vi "Advanced Auto Code.vi"   [LabVIEW 2017]
uses:
  <vilib>/Rock Robotics/WPI/ThirdParty/Phoenix-LabVIEW/Motor Controller/Controls/CTRE_Phoenix_MotorControl_RemoteSourceType.ctl
  <vilib>/Rock Robotics/WPI/ThirdParty/Phoenix-LabVIEW/Motor Controller/Controls/CTRE_Phoenix_MotorControl_ControlMode.ctl
  <vilib>/Rock Robotics/WPI/Utilities/WPI_GetSetVariantRefNum.vi
  <vilib>/Rock Robotics/Network Tables/NT Read String.vi
  Robot Global Data.vi
  <vilib>/Rock Robotics/WPI/RobotDrive/WPI_RobotDriveArcadeDrive_Standard(NoSaturation).vi
  <vilib>/addons/control/pid/pid.llb/PID (DBL).vi
  <vilib>/Rock Robotics/WPI/ThirdParty/Phoenix-LabVIEW/Motor Controller/Get/CTRE_Phoenix_MotorController_GetPulseWidthAll.vi
  <vilib>/addons/control/pid/NI_PID_pid.lvlib
types:
  T1 = cluster{"proportional gain (Kc)":dbl, "integral time (Ti, min)":dbl, "derivative time (Td, min)":dbl}
  T2 = enum16{"DemandType_Neutral", "DemandType_AuxPID", "DemandType_ArbitraryFeedForward"}
  T3 = typedef "CTRE_Phoenix_MotorControl_RemoteSourceType.ctl" = enum16{"Off", "Talon SRX Selected Sensor", "Pigeon IMU Yaw", "Pigeon IMU Pitch", "Pigeon IMU Roll", "CANifier Quadrature", "CANifier PWM Input 0", "CANifier PWM Input 1", "CANifier PWM Input 2", "CANifier PWM Input 3", "Gadgeteer Pigeon Yaw", "Gadgeteer Pigeon Pitch", "Gadgeteer Pigeon Roll"}
  T4 = typedef "WPI_MotorControlDeviceRef.ctl" = cluster{"DeviceStatus":errorcluster, "Type":T5, "PWM":cluster{"PWM Channel":T6, "DeadBand":T7}, "CAN":cluster{"Device Number":u8, "SetOutput VI Ref":variant, "GetOutput VI Ref":variant, "Enable VI Ref":variant, "Disable VI Ref":variant, "Data":variant}, "Invert":bool, "DIO PWM":cluster{"PWM \"Enable\" Channel":T6, "DIOChannel":T8, "PWM Rate":dbl}}
  T5 = typedef "WPI_MotorControlType.ctl" = enum16{"PWM", "CAN", "DIO PWM"}
  T6 = typedef "FPGA_DIOPWMChannel.ctl" = enum8{"PWM 0", "PWM 1", "PWM 2", "PWM 3", "PWM 4", "PWM 5", "PWM 6", "PWM 7", "PWM 8", "PWM 9", "PWM MXP 0", "PWM MXP 1", "PWM MXP 2", "PWM MXP 3", "PWM MXP 4", "PWM MXP 5", "PWM MXP 6", "PWM MXP 7", "PWM MXP 8", "PWM MXP 9", "Invalid"}
  T7 = typedef "WPI_PWMDeadband.ctl" = cluster{"Name":string, "maxPositivePwm":i32, "minPositivePwm":i32, "centerPwm":i32, "maxNegativePwm":i32, "minNegativePwm":i32, "angularRange":u16}
  T8 = typedef "FPGA_DIOChannel.ctl" = enum8{"DIO 0", "DIO 1", "DIO 2", "DIO 3", "DIO 4", "DIO 5", "DIO 6", "DIO 7", "DIO 8", "DIO 9", "DIO MXP 0", "DIO MXP 1", "DIO MXP 2", "DIO MXP 3", "DIO MXP 4", "DIO MXP 5", "DIO MXP 6", "DIO MXP 7", "DIO MXP 8", "DIO MXP 9", "DIO MXP 10", "DIO MXP 11", "DIO MXP 12", "DIO MXP 13", "DIO MXP 14", "DIO MXP 15", "SPI Port CS1", "SPI Port CS2", "SPI Port CS3", "SPI Port MISO", "SPI Port MOSI", "Invalid"}
  T9 = typedef "WPI_AnalogChannelDevRef.ctl" = cluster{"DevStatus":errorcluster, "Analog Channel":T10}
  T10 = typedef "FPGA_AIChannel.ctl" = enum8{"AI 0", "AI 1", "AI 2", "AI 3", "AI MXP 0", "AI MXP 1", "AI MXP 2", "AI MXP 3", "Invalid"}
  T11 = typedef "WPI_SwitchDevRef.ctl" = cluster{"DevStatus":errorcluster, "DIO Channel":T8, "CntIndex":T12, "Normally Closed":bool}
  T12 = typedef "FPGA_CounterCtrSystemIndex.ctl" = enum8{"Ctr 0", "Ctr 1", "Ctr 2", "Ctr 3", "Ctr 4", "Ctr 5", "Ctr 6", "Ctr 7", "Invalid"}
  T13 = typedef "WPI_RobotDriveDevRef.ctl" = cluster{"DevStatus":errorcluster, "Motors[]":T4[], "Square Inputs":bool, "Max Output":dbl}
  T14 = typedef "CTRE_Phoenix_MotorControl_ControlMode.ctl" = u16
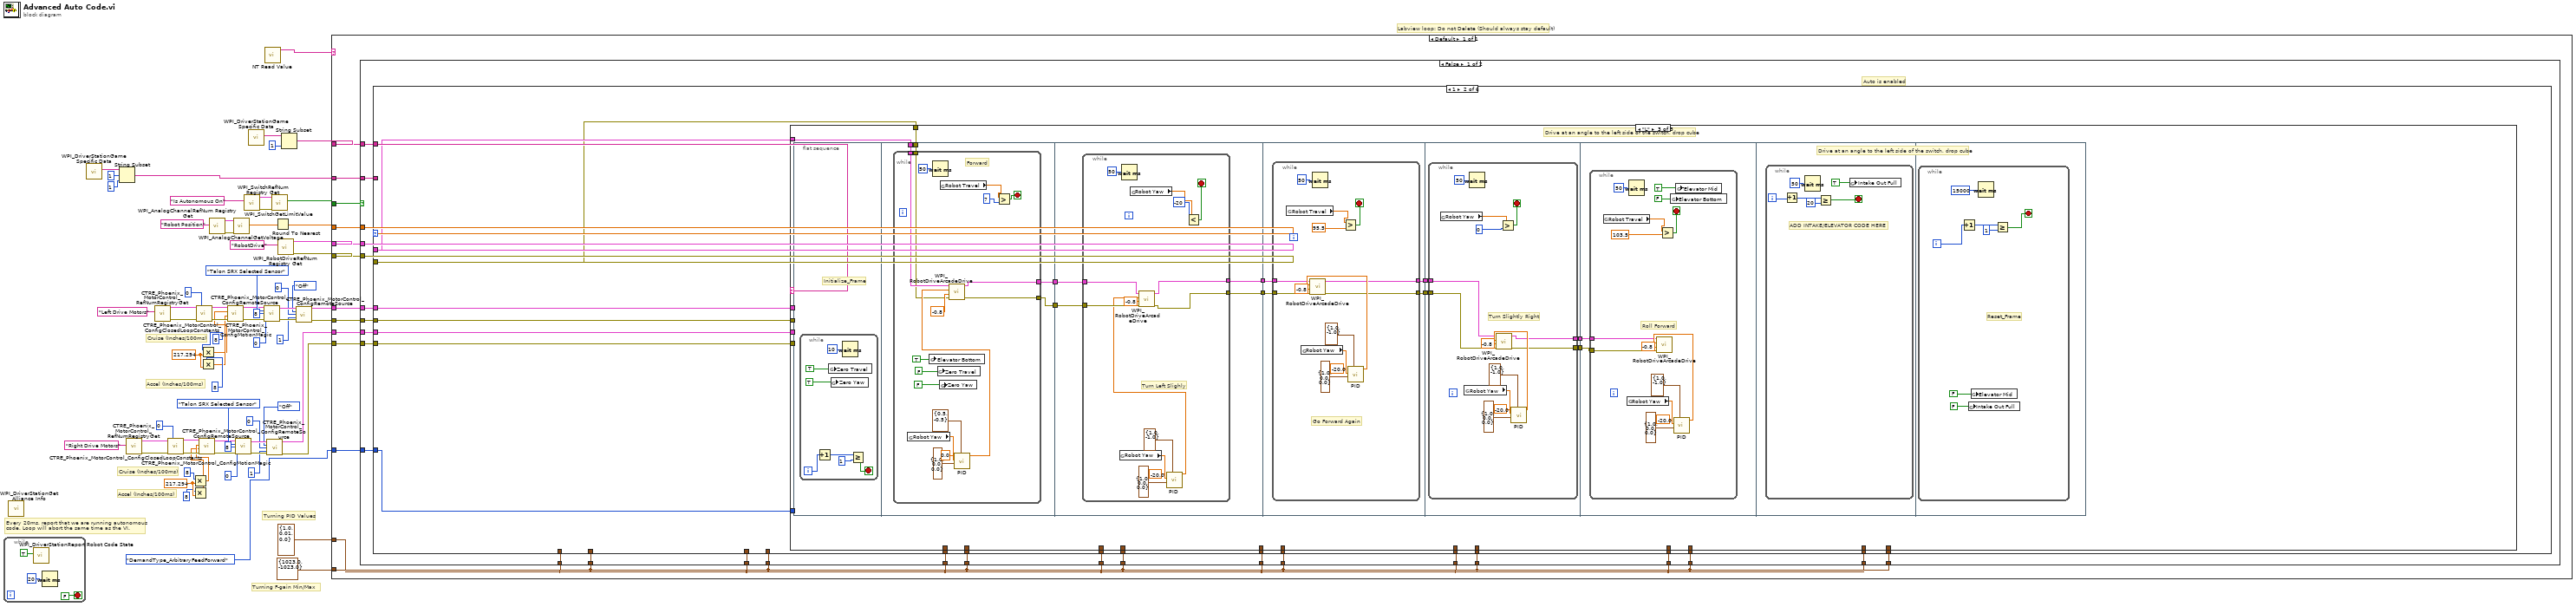
[diagram p0: block diagram]
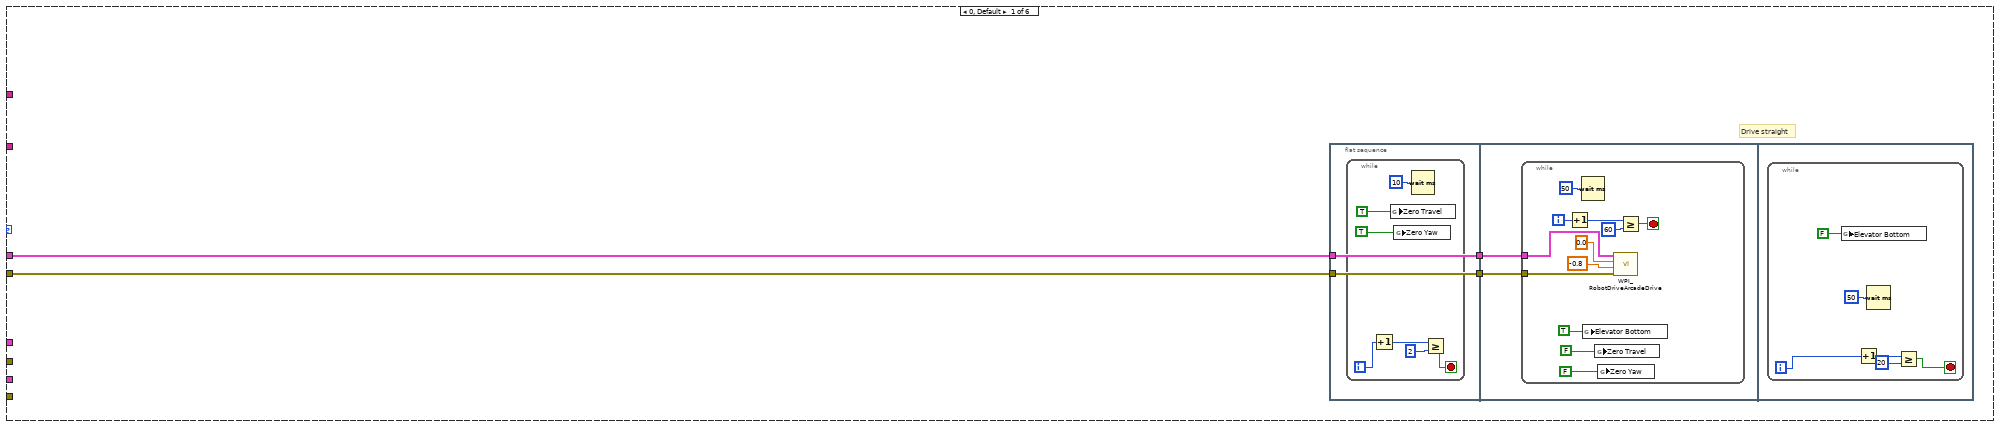
[diagram p2: hidden frame]
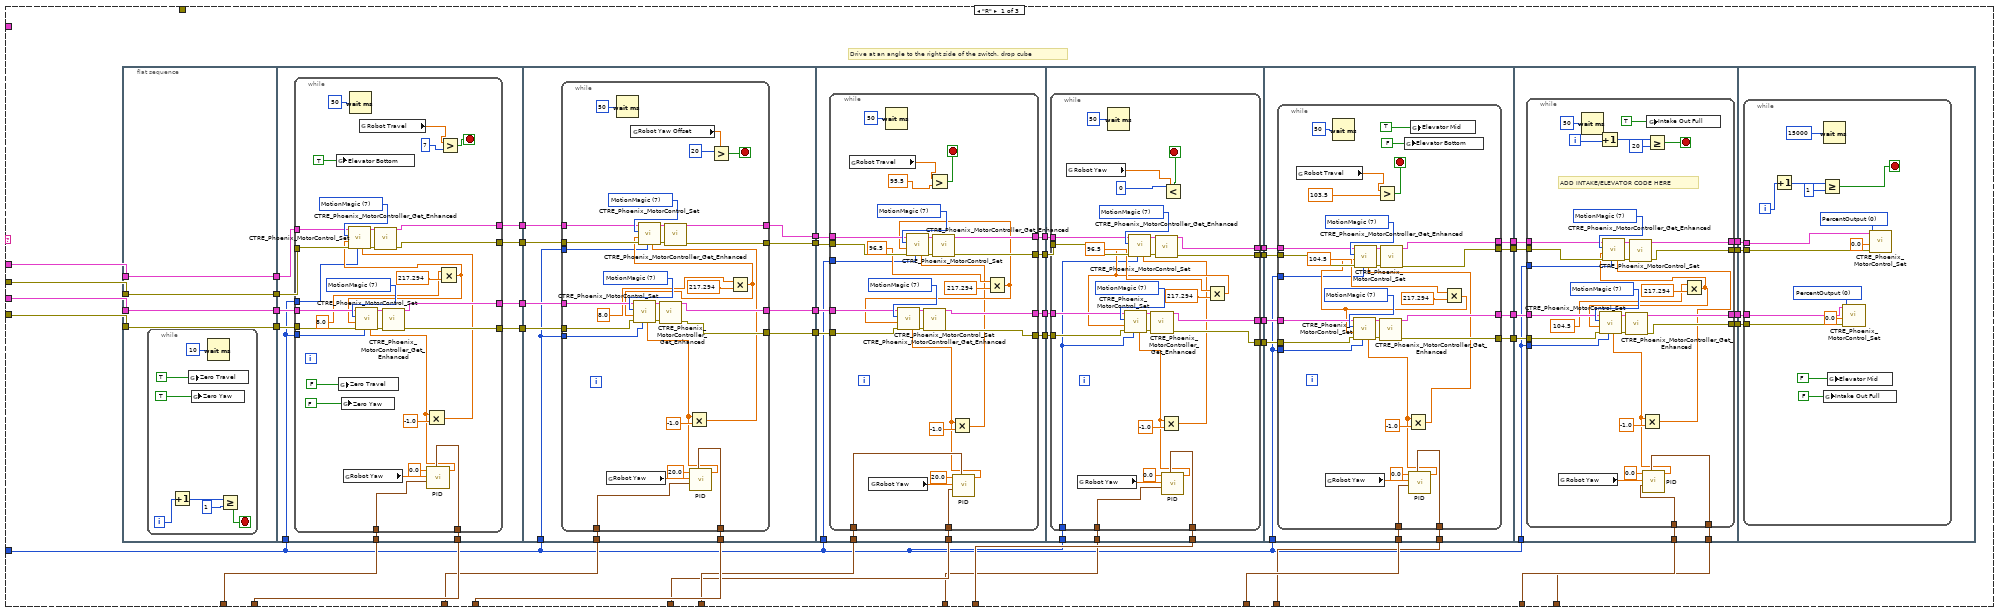
[diagram p3: hidden frame]
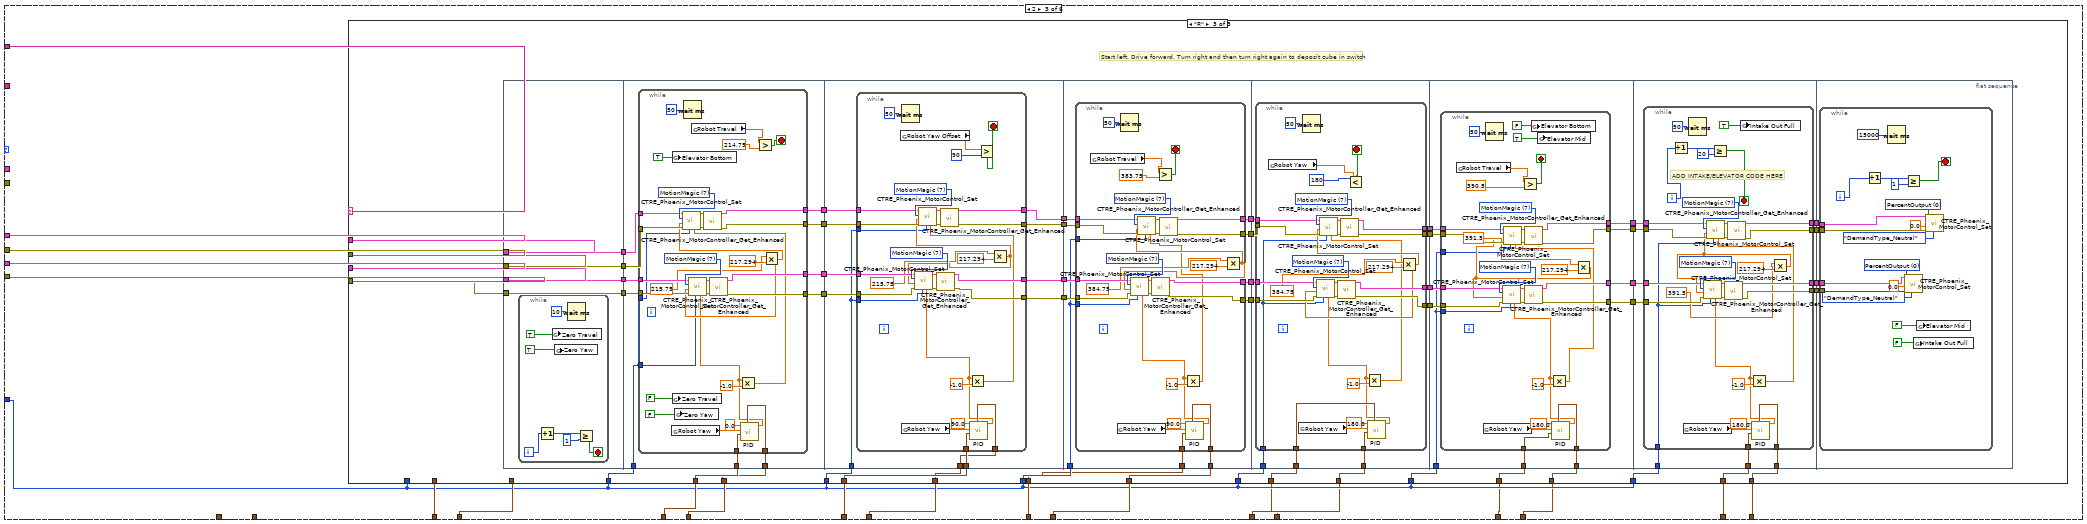
[diagram p5: hidden frame]
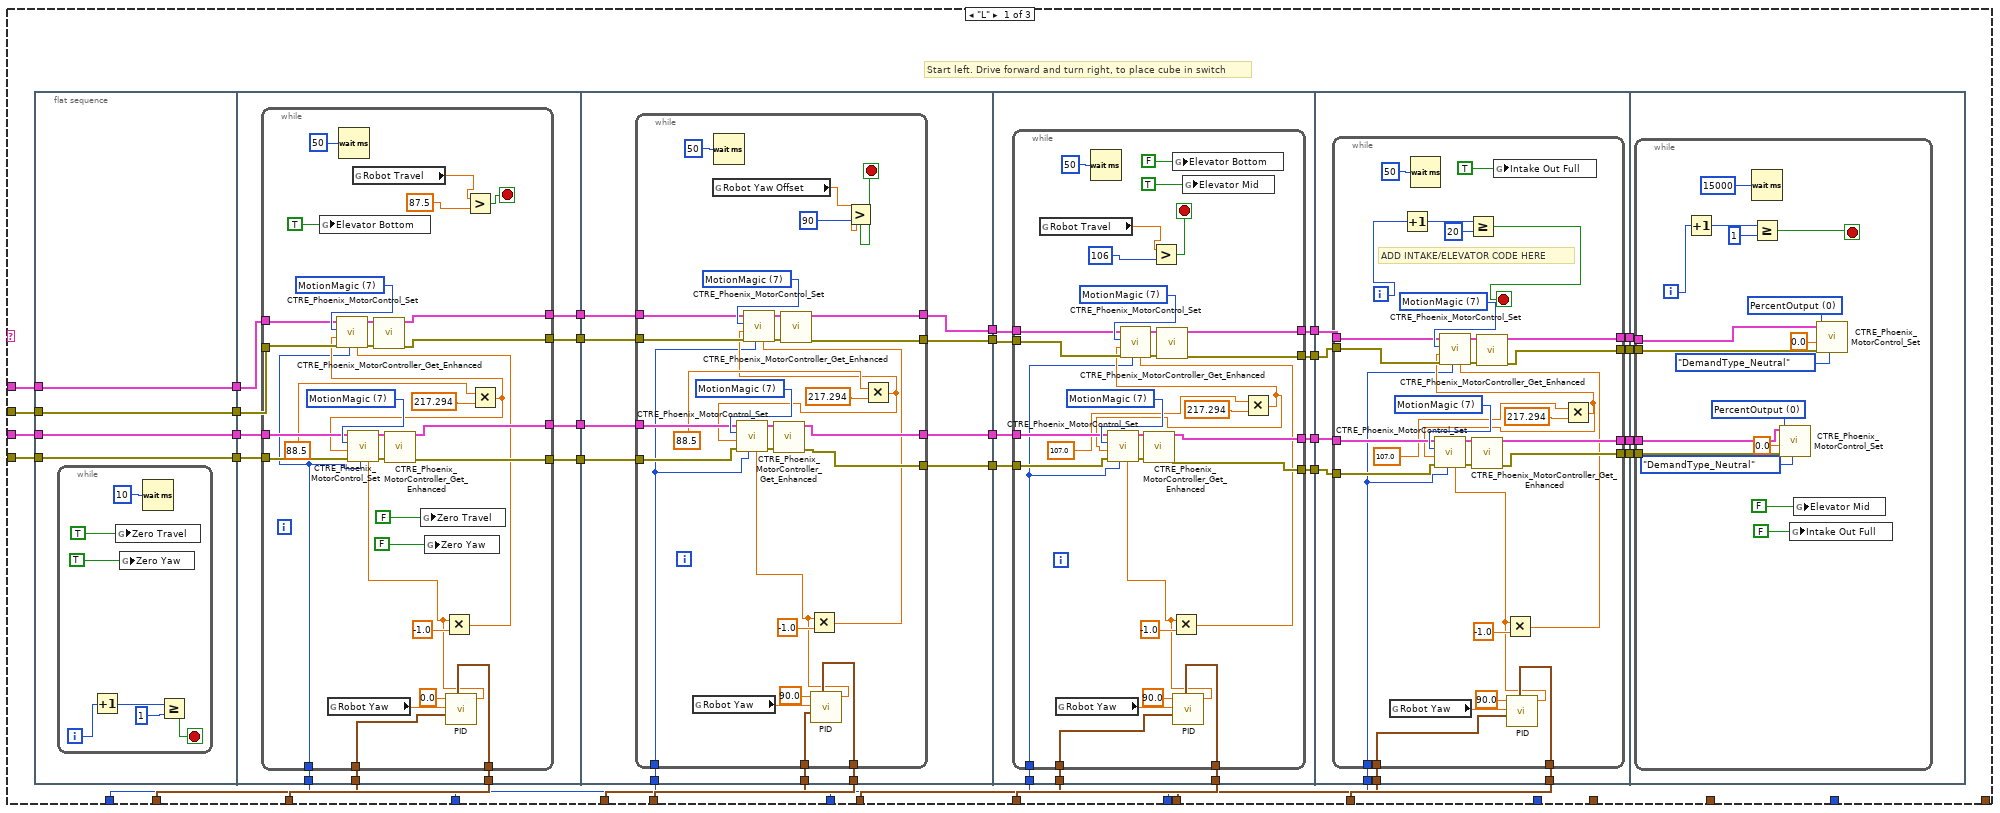
[diagram p6: hidden frame]
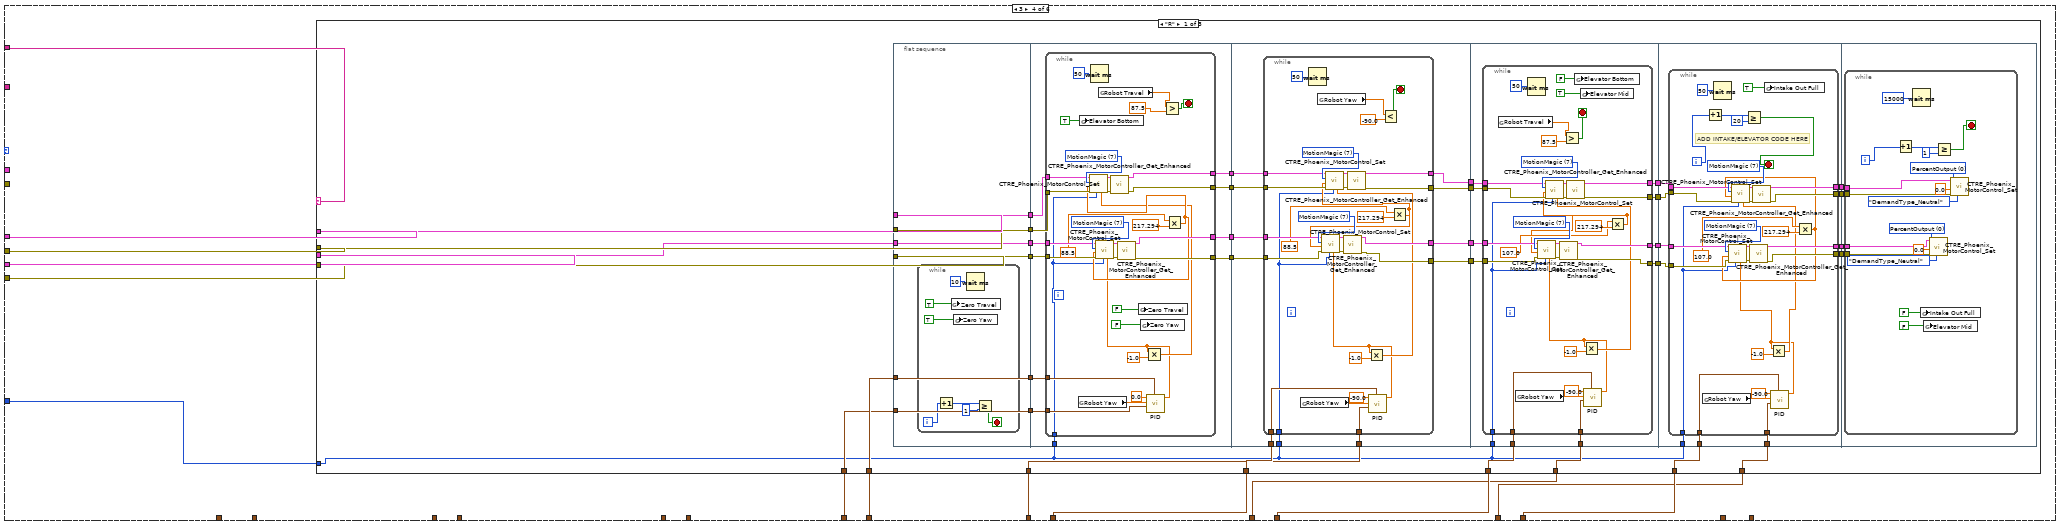
[diagram p8: hidden frame]
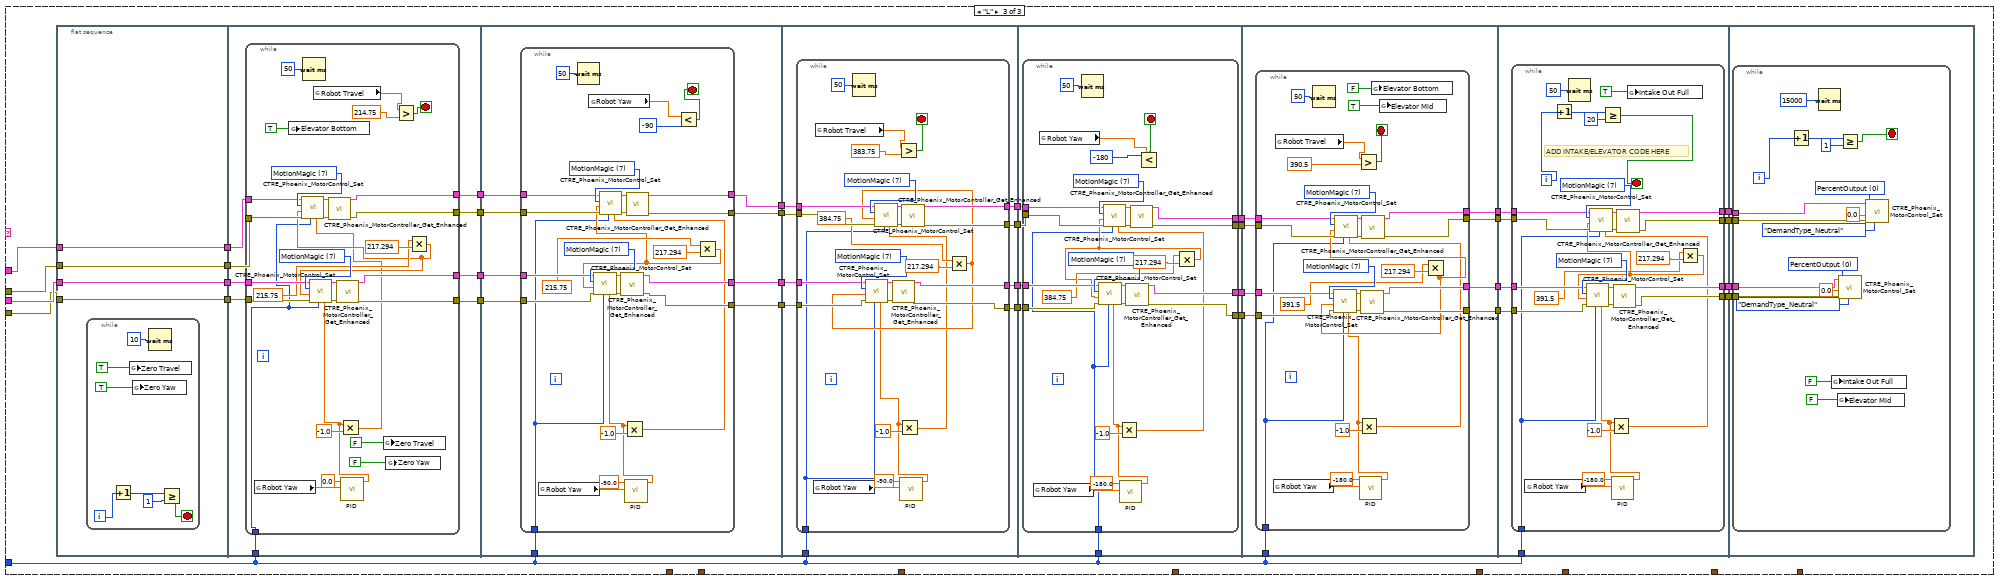
[diagram p10: hidden frame]
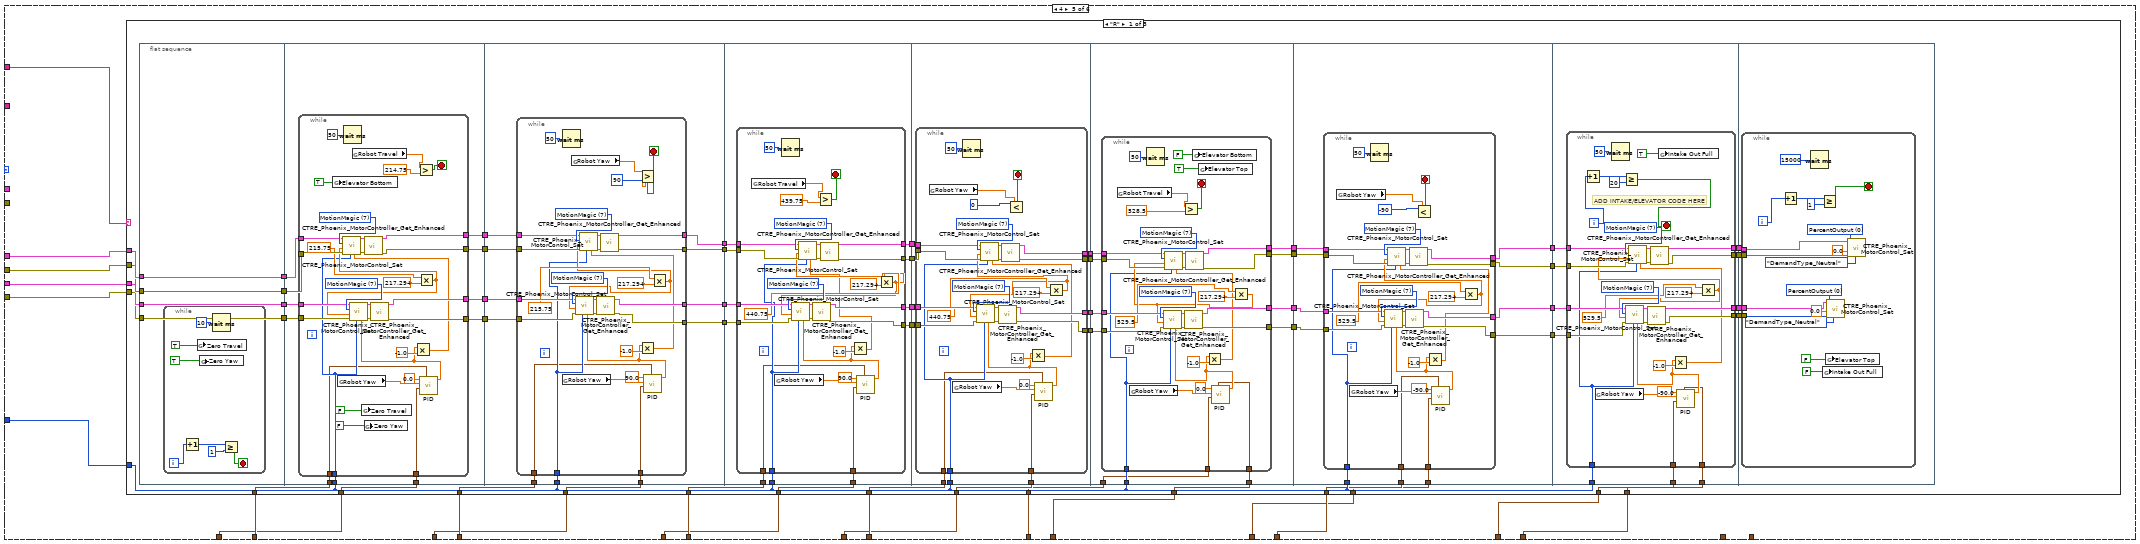
[diagram p11: hidden frame]
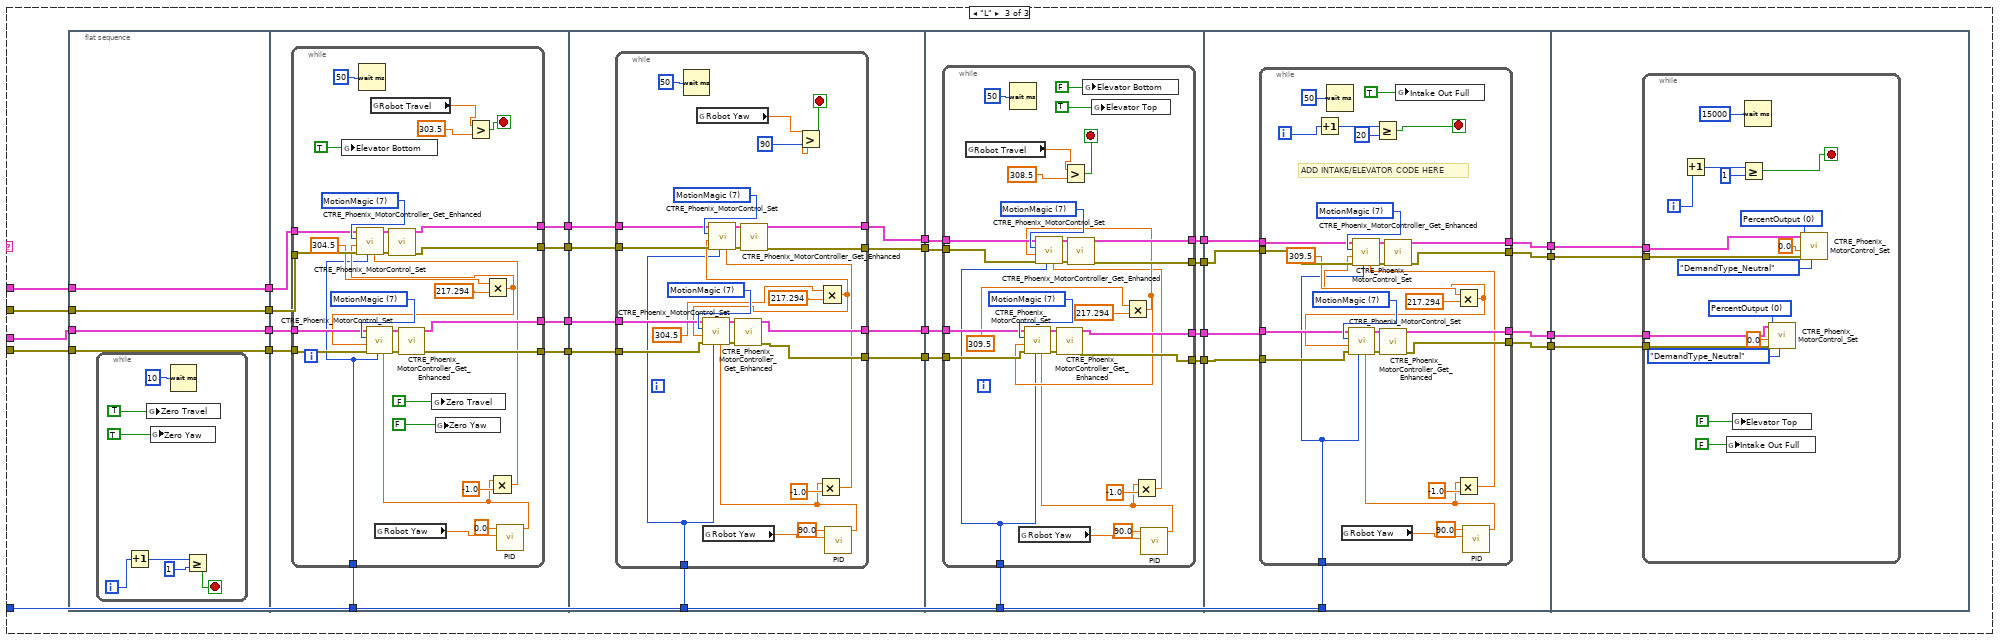
[diagram p13: hidden frame]
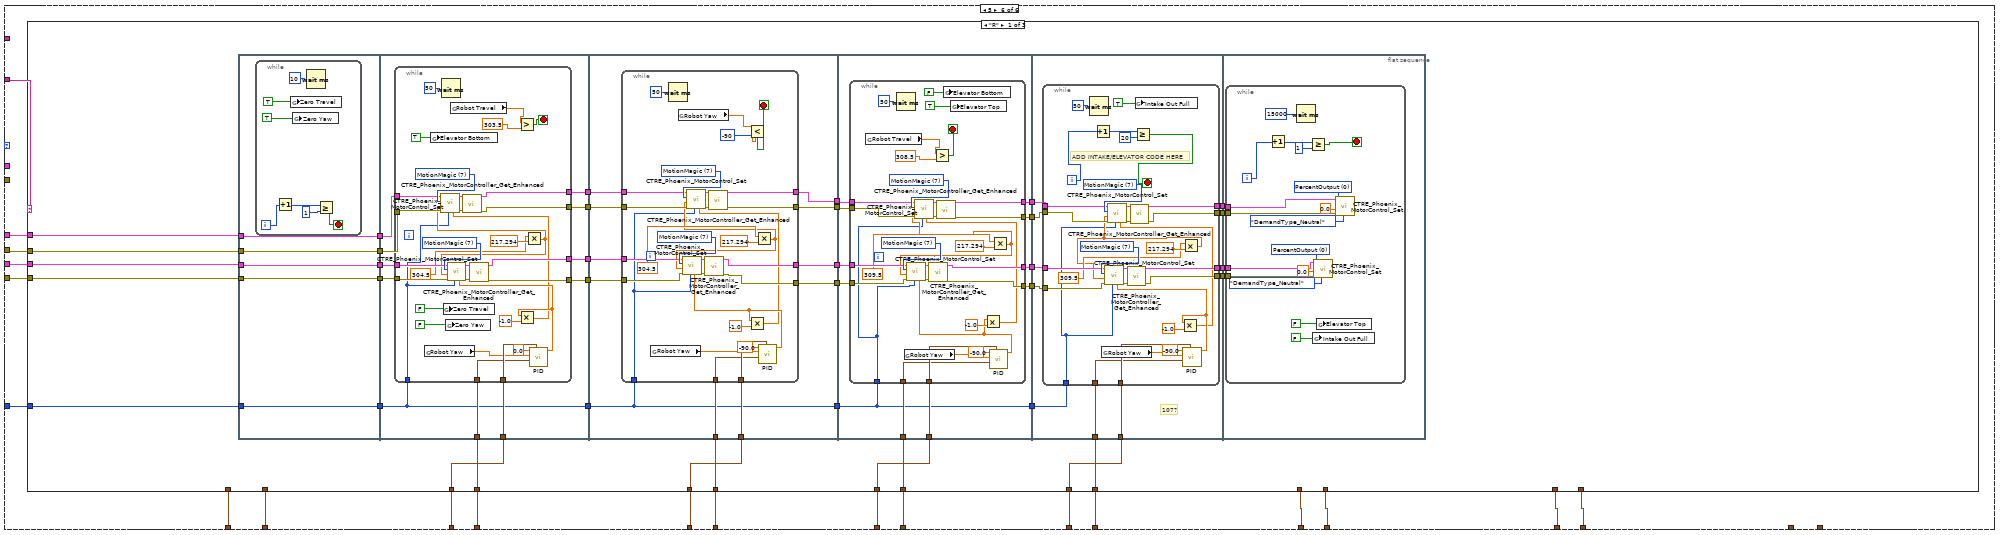
[diagram p14: hidden frame]
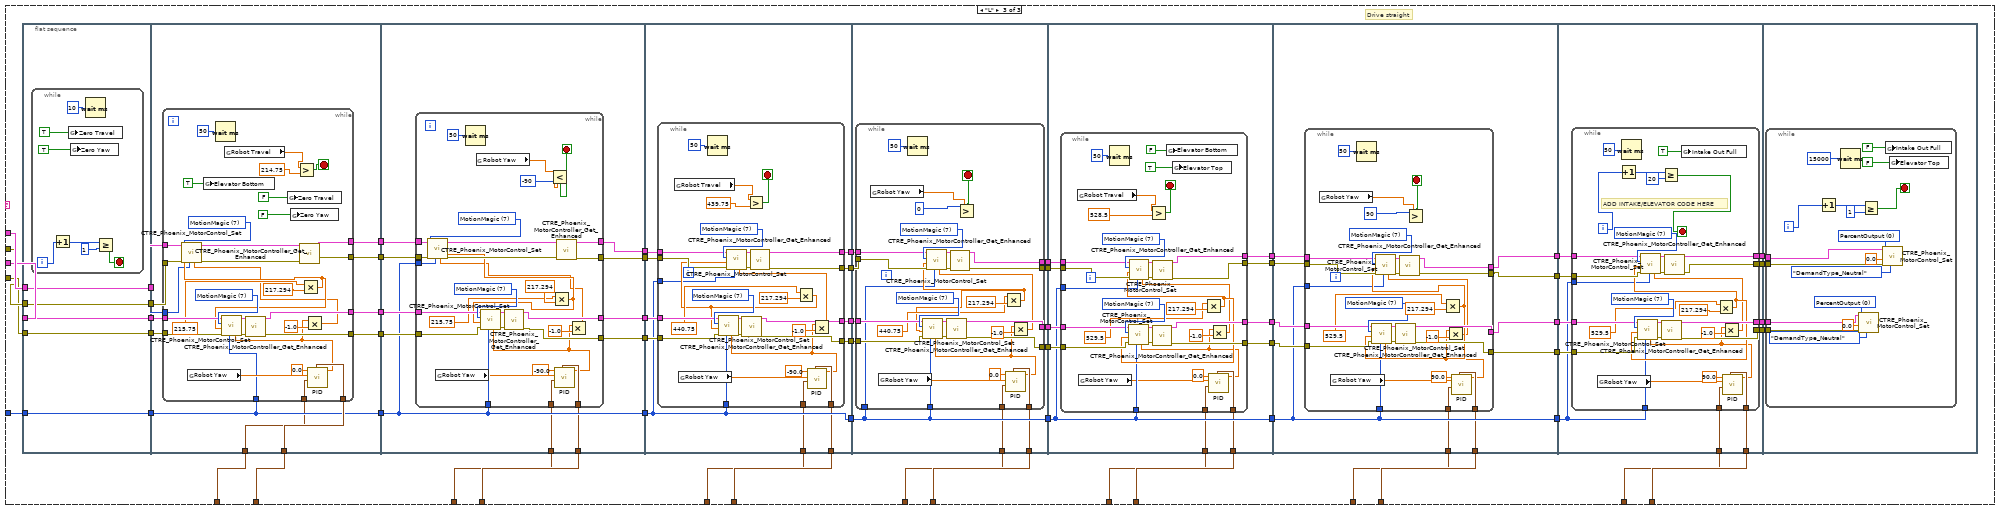
[diagram p16: hidden frame]
diagram:
  w8 = 217.294 ("y")
  w12 = 217.294 ("y")
  # "Turning F-gain Min/Max"
  # "Turning PID Values"
  # "Cruise (Inches/100ms)"
  # "Accel (Inches/100ms)"
  # "Cruise (Inches/100ms)"
  # "Accel (Inches/100ms)"
  # "Labview loop: Do not Delete (Should always stay default)"
  # "Every 20ms, report that we are running autonomous\ncode. Loop will abort the same time as the VI."
  n1 = while {
    stop <- FALSE stop-if-true
    n2 = call <vilib>:"WPI_DriverStationReport Robot Code State.vi"("Autonomous"=TRUE) -> ()  [unwired: 10 in, 1 out]
    n3 = Wait (ms)(milliseconds to wait=u32 20) -> ()  [unwired: 1 out]
  }
  n4 = call <vilib>:"WPI_DriverStationGet Alliance Info.vi"() -> ()  [unwired: 12 out]
  n5 = call <vilib>:"WPI_DriverStationGame Specific Data.vi"() -> ("Game Specific Data"=w60:string)  [unwired: 11 in]
  n6 = String Subset(string=w60, offset (0)=1, length (rest)=1 ("length (rest)")) -> (substring=w59:string)
  n7 = call <vilib>:"CTRE_Phoenix_MotorControl_RefNumRegistryGet.vi"("refnum name"="Right Drive Motors") -> ("error out"=w30:errorcluster, "PhoenixMotorControlDevRef"=w28:T4)  [unwired: 9 in]
  n8 = call <vilib>:"CTRE_Phoenix_MotorControl_RefNumRegistryGet.vi"("refnum name"="Left Drive Motors") -> ("error out"=w48:errorcluster, "PhoenixMotorControlDevRef"=w46:T4)  [unwired: 9 in]
  n9 = call <vilib>:"CTRE_Phoenix_MotorControl_ConfigClosedLoopConstants.vi"("PhoenixMotorControlDevRef"=w28, "slotIdx"=0, "error in (no error)"=w30) -> ("PhoenixMotorControlDevRef"=w27:T4, "error out"=w29:errorcluster)  [unwired: 11 in]
  n10 = Multiply(x=8 ("Cruise Velocity"), y=w8) -> (x*y=w5:dbl)
  n11 = Multiply(x=8 ("Acceleration"), y=w8) -> (x*y=w4:dbl)
  n12 = call <vilib>:"CTRE_Phoenix_MotorControl_ConfigClosedLoopConstants.vi"("PhoenixMotorControlDevRef"=w46, "slotIdx"=0, "error in (no error)"=w48) -> ("PhoenixMotorControlDevRef"=w45:T4, "error out"=w47:errorcluster)  [unwired: 11 in]
  n13 = call <vilib>:"CTRE_Phoenix_MotorControl_ConfigMotionMagic.vi"("error in (no error)"=w29, "Acceleration"=w4, "Cruise Velocity"=w5, "PhoenixMotorControlDevRef"=w27) -> ("error out"=w16:errorcluster, "PhoenixMotorControlDevRef"=w17:T4)  [unwired: 6 in]
  n14 = Multiply(x=8 ("Cruise Velocity"), y=w12) -> (x*y=w9:dbl)
  n15 = Multiply(x=8 ("Acceleration"), y=w12) -> (x*y=w10:dbl)
  n16 = call <vilib>:"WPI_AnalogChannelRefNum Registry Get.vi"("refnum name"="Robot Position") -> ("error out"=w58:errorcluster, "AIDeviceRef"=w57:T9)  [unwired: 9 in]
  n17 = call <vilib>:"CTRE_Phoenix_MotorControl_ConfigMotionMagic.vi"("error in (no error)"=w47, "Acceleration"=w10, "Cruise Velocity"=w9, "PhoenixMotorControlDevRef"=w45) -> ("error out"=w34:errorcluster, "PhoenixMotorControlDevRef"=w35:T4)  [unwired: 6 in]
  n18 = call <vilib>:"WPI_AnalogChannelGetVoltage.vi"("error in (no error)"=w58, "AIDeviceRef"=w57) -> ("Voltage"=w56:dbl)  [unwired: 7 in, 2 out]
  n19 = call <vilib>:"CTRE_Phoenix_MotorControl_ConfigRemoteSource.vi"("PhoenixMotorControlDevRef"=w17, "Remote Device Type"=CTRE_Phoenix_MotorControl_RemoteSourceType."Talon SRX Selected Sensor", "Remote Device ID"=u8 8, "Source Index (0/1)"=u32 0, "error in (no error)"=w16) -> ("PhoenixMotorControlDevRef"=w22:T4, "error out"=w21:errorcluster)  [unwired: 9 in]
  n20 = call <vilib>:"WPI_SwitchRefNum Registry Get.vi"("refnum name"="Is Autonomous On") -> ("error out"=w65:errorcluster, "SwitchDevRef"=w64:T11)  [unwired: 9 in]
  n21 = call <vilib>:"WPI_DriverStationGame Specific Data.vi"() -> ("Game Specific Data"=w62:string)  [unwired: 11 in]
  n22 = call <vilib>:"CTRE_Phoenix_MotorControl_ConfigRemoteSource.vi"("PhoenixMotorControlDevRef"=w35, "Remote Device Type"=CTRE_Phoenix_MotorControl_RemoteSourceType."Talon SRX Selected Sensor", "Remote Device ID"=u8 8, "Source Index (0/1)"=u32 0, "error in (no error)"=w34) -> ("PhoenixMotorControlDevRef"=w40:T4, "error out"=w39:errorcluster)  [unwired: 9 in]
  n23 = call-poly <vilib>:"NT Read Value.vi"() -> ("String"=w68:string)  [unwired: 10 in, 1 out]
  n24 = call <vilib>:"CTRE_Phoenix_MotorControl_ConfigRemoteSource.vi"("PhoenixMotorControlDevRef"=w22, "Remote Device Type"=CTRE_Phoenix_MotorControl_RemoteSourceType."Off", "Remote Device ID"=u8 0, "Source Index (0/1)"=u32 1, "error in (no error)"=w21) -> ("PhoenixMotorControlDevRef"=w15:T4, "error out"=w14:errorcluster)  [unwired: 9 in]
  n25 = call <vilib>:"WPI_SwitchGetLimitValue.vi"("error in (no error)"=w65, "SwitchDevRef"=w64) -> ("Switch Pressed"=w54:bool)  [unwired: 7 in, 2 out]
  n26 = Round To Nearest(number=w56) -> (nearest integer value=w55:dbl)
  n27 = call <vilib>:"WPI_RobotDriveRefNum Registry Get.vi"("refnum name"="RobotDrive") -> ("error out"=w50:errorcluster, "RobotDriveDevRef"=w51:T13)  [unwired: 1 in, 8 out]
  n28 = String Subset(string=w62, length (rest)=1 ("length (rest)")) -> (substring=w66:string)  [unwired: 1 in]
  n29 = call <vilib>:"CTRE_Phoenix_MotorControl_ConfigRemoteSource.vi"("PhoenixMotorControlDevRef"=w40, "Remote Device Type"=CTRE_Phoenix_MotorControl_RemoteSourceType."Off", "Remote Device ID"=u8 0, "Source Index (0/1)"=u32 1, "error in (no error)"=w39) -> ("PhoenixMotorControlDevRef"=w33:T4, "error out"=w32:errorcluster)  [unwired: 9 in]
  n30 = case shown="Default" w68 {
    tunnel: w66 -> [w85]
    tunnel: w54 -> [w84]
    tunnel: w59 -> [w83]
    tunnel: w55 -> [w82]
    tunnel: w51 -> [w81]
    tunnel: w50 -> [w80]
    tunnel: w33 -> [w79]
    tunnel: w32 -> [w78]
    tunnel: w15 -> [w77]
    tunnel: w14 -> [w76]
    tunnel: cluster{"output high":dbl, "output low":dbl} {"output high"=1023.0, "output low"=-1023.0} ("output range") -> [w74]
    tunnel: T2."DemandType_ArbitraryFeedForward" ("DemandType") -> [w75]
    tunnel: T1 {"proportional gain (Kc)"=1.0, "integral time (Ti, min)"=0.01, "derivative time (Td, min)"=0.0} ("PID gains") -> [w73]
    frame Default {
      n31 = case shown="False" w84 {
        tunnel: w85 -> [w108 _]
        tunnel: w83 -> [w103 _]
        tunnel: w82 -> [w111 _]
        tunnel: w81 -> [w110 _]
        tunnel: w80 -> [w109 _]
        tunnel: w79 -> [w107 _]
        tunnel: w78 -> [w106 _]
        tunnel: w77 -> [w105 _]
        tunnel: w76 -> [w104 _]
        tunnel: w74 -> [w102 _]
        tunnel: w75 -> [w101 _]
        tunnel: w74 -> [w100 _]
        tunnel: w74 -> [w99 _]
        tunnel: w74 -> [w98 _]
        tunnel: w74 -> [w97 _]
        tunnel: w74 -> [w96 _]
        tunnel: w74 -> [w95 _]
        tunnel: w73 -> [w94 _]
        tunnel: w73 -> [w93 _]
        tunnel: w73 -> [w92 _]
        tunnel: w73 -> [w91 _]
        tunnel: w73 -> [w90 _]
        tunnel: w73 -> [w89 _]
        tunnel: w73 -> [w88 _]
        tunnel: w74 -> [w87 _]
        tunnel: w73 -> [w86 _]
        frame False {
          # "Auto is enabled"
          n32 = case shown="1" w111 {
            tunnel: w110 -> [w115 w146 _ _ _ _]
            tunnel: w109 -> [w114 w145 _ _ _ _]
            tunnel: w108 -> [_ w164 w631 w1213 w1757 _]
            tunnel: w107 -> [_ w163 w630 w1212 w1756 w2354]
            tunnel: w106 -> [_ w162 w629 w1211 w1755 w2353]
            tunnel: w105 -> [_ w161 w628 w1210 w1754 w2352]
            tunnel: w104 -> [_ w160 w627 w1209 w1753 w2351]
            tunnel: w103 -> [_ _ _ _ _ w2355]
            tunnel: w102 -> [_ w158 w625 _ w1747 w2350]
            tunnel: w101 -> [_ w159 w618 w1208 w1752 w2349]
            tunnel: w100 -> [_ w156 w624 w1201 w1745 w2348]
            tunnel: w99 -> [_ w154 w623 w1203 w1743 w2347]
            tunnel: w98 -> [_ w152 w616 w1205 w1741 w2346]
            tunnel: w97 -> [_ w149 w614 w1207 w1739 w2345]
            tunnel: w96 -> [_ _ _ _ w1751 w2344]
            tunnel: w95 -> [_ _ w626 _ w1749 w2343]
            tunnel: w94 -> [_ w150 w615 w1206 w1738 w2342]
            tunnel: w93 -> [_ _ _ _ w1750 w2341]
            tunnel: w92 -> [_ _ w619 _ w1748 w2340]
            tunnel: w91 -> [_ w155 w621 w1200 w1744 w2339]
            tunnel: w90 -> [_ w153 w622 w1202 w1742 w2338]
            tunnel: w89 -> [_ w151 w617 w1204 w1740 w2337]
            tunnel: w88 -> [_ w157 w620 _ w1746 w2336]
            tunnel: w87 -> [_ w147 w613 _ _ _]
            tunnel: w86 -> [_ w148 w612 _ _ _]
            frame 0, Default {
              # "Drive straight"
              n33 = flat-sequence {
                tunnel: w114 -> [w116]
                tunnel: w115 -> [w117]
                tunnel: [w117] -> w113
                tunnel: [w116] -> w112
                tunnel: w113 -> [w126]
                tunnel: w112 -> [w125]
                frame #0 {
                  n34 = while {
                    i -> [w119]
                    stop <- w120 stop-if-true
                    n35 = Increment(x=w119) -> (x+1=w121:i32)
                    n36 = global write "Robot Global Data.vi" "Zero Travel"(TRUE) -> ()
                    n37 = global write "Robot Global Data.vi" "Zero Yaw"(TRUE) -> ()
                    n38 = Wait (ms)(milliseconds to wait=u32 10) -> ()  [unwired: 1 out]
                    n39 = Greater Or Equal?(x=w121, y=2) -> (x >= y?=w120:bool)
                  }
                }
                frame #1 {
                  n40 = while {
                    tunnel: w126 -> [w133]
                    tunnel: w125 -> [w132]
                    i -> [w136]
                    stop <- w137 stop-if-true
                    n41 = Increment(x=w136) -> (x+1=w134:i32)
                    n42 = Wait (ms)(milliseconds to wait=u32 50) -> ()  [unwired: 1 out]
                    n43 = global write "Robot Global Data.vi" "Elevator Bottom"(TRUE) -> ()
                    n44 = global write "Robot Global Data.vi" "Zero Travel"(FALSE) -> ()
                    n45 = global write "Robot Global Data.vi" "Zero Yaw"(FALSE) -> ()
                    n46 = call-poly <vilib>:"WPI_RobotDriveArcadeDrive.vi"("error in (no error)"=w132, "Y axis value"=-0.8, "X axis value"=0.0, "RobotDriveDevRef"=w133) -> ()  [unwired: 5 in, 3 out]
                    n47 = Greater Or Equal?(x=w134, y=60) -> (x >= y?=w137:bool)
                  }
                }
                frame #2 {
                  n48 = while {
                    i -> [w142]
                    stop <- w140 stop-if-true
                    n49 = global write "Robot Global Data.vi" "Elevator Bottom"(FALSE) -> ()
                    n50 = Increment(x=w142) -> (x+1=w141:i32)
                    n51 = Wait (ms)(milliseconds to wait=u32 50) -> ()  [unwired: 1 out]
                    n52 = Greater Or Equal?(x=w141, y=20) -> (x >= y?=w140:bool)
                  }
                }
              }
            }
            frame 1 {
              n53 = case shown="\"L\"" w164 {
                tunnel: w163 -> [w191 _ _]
                tunnel: w162 -> [w190 _ _]
                tunnel: w161 -> [w189 _ _]
                tunnel: w160 -> [w188 _ _]
                tunnel: w159 -> [w169 _ _]
                tunnel: w158 -> [w181 _ _]
                tunnel: w157 -> [w180 _ _]
                tunnel: w156 -> [w179 _ _]
                tunnel: w155 -> [w178 _ _]
                tunnel: w154 -> [w177 _ _]
                tunnel: w153 -> [w176 _ _]
                tunnel: w152 -> [w175 _ _]
                tunnel: w151 -> [w174 _ _]
                tunnel: w150 -> [w173 _ _]
                tunnel: w149 -> [w172 _ _]
                tunnel: w148 -> [w171 _ _]
                tunnel: w147 -> [w170 _ _]
                tunnel: w146 -> [_ _ w492]
                tunnel: w145 -> [_ _ w491]
                frame "R" {
                  # "Drive at an angle to the right side of the switch, drop cube"
                  n54 = flat-sequence {
                    tunnel: w188 -> [w210]
                    tunnel: w189 -> [w211]
                    tunnel: w190 -> [w212]
                    tunnel: w191 -> [w213]
                    tunnel: [w213] -> w168
                    tunnel: [w212] -> w167
                    tunnel: [w211] -> w166
                    tunnel: [w210] -> w165
                    tunnel: [w229] -> w209
                    tunnel: [w228] -> w208
                    tunnel: [w225] -> w183
                    tunnel: [w224] -> w182
                    tunnel: w181 -> [w223]
                    tunnel: w180 -> [w222]
                    tunnel: w169 -> [w221]
                    tunnel: w168 -> [w231]
                    tunnel: w167 -> [w230]
                    tunnel: w166 -> [w227]
                    tunnel: w165 -> [w226]
                    tunnel: w209 -> [w275]
                    tunnel: w208 -> [w274]
                    tunnel: [w273] -> w207
                    tunnel: [w272] -> w206
                    tunnel: [w271] -> w185
                    tunnel: [w270] -> w184
                    tunnel: w183 -> [w269]
                    tunnel: w182 -> [w268]
                    tunnel: w179 -> [w267]
                    tunnel: w178 -> [w266]
                    tunnel: w169 -> [w265]
                    tunnel: w207 -> [w316]
                    tunnel: w206 -> [w315]
                    tunnel: [w314] -> w205
                    tunnel: [w313] -> w204
                    tunnel: [w312] -> w187
                    tunnel: [w311] -> w186
                    tunnel: w185 -> [w310]
                    tunnel: w184 -> [w309]
                    tunnel: w169 -> [w308]
                    tunnel: w177 -> [w307]
                    tunnel: w176 -> [w306]
                    tunnel: w205 -> [w356]
                    tunnel: w204 -> [w355]
                    tunnel: [w354] -> w203
                    tunnel: [w353] -> w202
                    tunnel: [w352] -> w201
                    tunnel: [w351] -> w200
                    tunnel: w187 -> [w350]
                    tunnel: w186 -> [w349]
                    tunnel: w169 -> [w348]
                    tunnel: w175 -> [w347]
                    tunnel: w174 -> [w346]
                    tunnel: w203 -> [w396]
                    tunnel: w202 -> [w395]
                    tunnel: [w394] -> w199
                    tunnel: [w393] -> w198
                    tunnel: w201 -> [w392]
                    tunnel: w200 -> [w391]
                    tunnel: [w390] -> w197
                    tunnel: [w389] -> w196
                    tunnel: w169 -> [w388]
                    tunnel: w173 -> [w387]
                    tunnel: w172 -> [w386]
                    tunnel: w199 -> [w439]
                    tunnel: w198 -> [w438]
                    tunnel: [w437] -> w195
                    tunnel: [w436] -> w194
                    tunnel: w197 -> [w435]
                    tunnel: w196 -> [w434]
                    tunnel: [w433] -> w193
                    tunnel: [w432] -> w192
                    tunnel: w169 -> [w431]
                    tunnel: w171 -> [w430]
                    tunnel: w170 -> [w429]
                    tunnel: w195 -> [w475]
                    tunnel: w194 -> [w474]
                    tunnel: w193 -> [w473]
                    tunnel: w192 -> [w472]
                    frame #0 {
                      n55 = while {
                        i -> [w215]
                        stop <- w216 stop-if-true
                        n56 = Increment(x=w215) -> (x+1=w217:i32)
                        n57 = global write "Robot Global Data.vi" "Zero Travel"(TRUE) -> ()
                        n58 = global write "Robot Global Data.vi" "Zero Yaw"(TRUE) -> ()
                        n59 = Wait (ms)(milliseconds to wait=u32 10) -> ()  [unwired: 1 out]
                        n60 = Greater Or Equal?(x=w217, y=1) -> (x >= y?=w216:bool)
                      }
                    }
                    frame #1 {
                      n61 = while {
                        tunnel: w231 -> [w259]
                        tunnel: w230 -> [w258]
                        tunnel: [w257] -> w229
                        tunnel: [w256] -> w228
                        tunnel: w227 -> [w250]
                        tunnel: w226 -> [w249]
                        tunnel: [w248] -> w225
                        tunnel: [w247] -> w224
                        tunnel: w223 -> [w239]
                        tunnel: w222 -> [w238]
                        tunnel: w221 -> [w237]
                        tunnel: w221 -> [w236]
                        stop <- w254 stop-if-true
                        w251 = T14 7 items=["PercentOutput"=0, "Position"=1, "Velocity"=2, "Current"=3, "Follower"=5, "MotionProfile"=6, "MotionMagic"=7, "MotionMagicArc"=8, "MotionProfileArc"=10, "Disabled"=15] ("Control Mode")
                        w260 = T14 7 items=["PercentOutput"=0, "Position"=1, "Velocity"=2, "Current"=3, "Follower"=5, "MotionProfile"=6, "MotionMagic"=7, "MotionMagicArc"=8, "MotionProfileArc"=10, "Disabled"=15] ("Control Mode")
                        n62 = global write "Robot Global Data.vi" "Elevator Bottom"(TRUE) -> ()
                        n63 = global write "Robot Global Data.vi" "Zero Travel"(FALSE) -> ()
                        n64 = global write "Robot Global Data.vi" "Zero Yaw"(FALSE) -> ()
                        n65 = global read "Robot Global Data.vi" "Robot Yaw"() -> (w242:dbl)
                        n66 = Wait (ms)(milliseconds to wait=u32 50) -> ()  [unwired: 1 out]
                        n67 = global read "Robot Global Data.vi" "Robot Travel"() -> (w255:dbl)
                        n68 = call-poly <vilib>:"PID.vi"("output range"=w239, "PID gains"=w238, "process variable"=w242, "setpoint"=0.0) -> ("output"=w235:dbl)  [unwired: 6 in, 1 out]
                        n69 = Multiply(x=w235, y=-1.0) -> (x*y=w234:dbl)
                        n70 = Multiply(x=8.0 ("Output"), y=217.294) -> (x*y=w244:dbl)
                        n71 = call <vilib>:"CTRE_Phoenix_MotorControl_Set.vi"("Demand1"=w234, "DemandType"=w237, "error in (no error)"=w258, "Output"=w244, "Control Mode"=w260, "PhoenixMotorControlDevRef"=w259) -> ("error out"=w262:errorcluster, "PhoenixMotorControlDevRef"=w261:T4)  [unwired: 4 in]
                        n72 = call <vilib>:"CTRE_Phoenix_MotorControl_Set.vi"("Demand1"=w235, "DemandType"=w236, "error in (no error)"=w249, "Output"=w244, "Control Mode"=w251, "PhoenixMotorControlDevRef"=w250) -> ("error out"=w253:errorcluster, "PhoenixMotorControlDevRef"=w252:T4)  [unwired: 4 in]
                        n73 = call-poly <vilib>:"CTRE_Phoenix_MotorController_Get_Enhanced.vi"("PhoenixMotorControlDevRef"=w261, "error in"=w262) -> ("PhoenixMotorControlDevRef"=w257:T4, "error out"=w256:errorcluster)  [unwired: 8 in, 4 out]
                        n74 = call-poly <vilib>:"CTRE_Phoenix_MotorController_Get_Enhanced.vi"("PhoenixMotorControlDevRef"=w252, "error in"=w253) -> ("PhoenixMotorControlDevRef"=w248:T4, "error out"=w247:errorcluster)  [unwired: 8 in, 4 out]
                        n75 = Greater?(x=w255, y=7) -> (0:w254:bool)
                      }
                    }
                    frame #2 {
                      n76 = while {
                        tunnel: w275 -> [w301]
                        tunnel: w274 -> [w300]
                        tunnel: [w299] -> w273
                        tunnel: [w298] -> w272
                        tunnel: [w294] -> w271
                        tunnel: [w293] -> w270
                        tunnel: w269 -> [w292]
                        tunnel: w268 -> [w291]
                        tunnel: w267 -> [w281]
                        tunnel: w266 -> [w280]
                        tunnel: w265 -> [w279]
                        tunnel: w265 -> [w278]
                        stop <- w290 stop-if-true
                        w295 = T14 7 items=["PercentOutput"=0, "Position"=1, "Velocity"=2, "Current"=3, "Follower"=5, "MotionProfile"=6, "MotionMagic"=7, "MotionMagicArc"=8, "MotionProfileArc"=10, "Disabled"=15] ("Control Mode")
                        w302 = T14 7 items=["PercentOutput"=0, "Position"=1, "Velocity"=2, "Current"=3, "Follower"=5, "MotionProfile"=6, "MotionMagic"=7, "MotionMagicArc"=8, "MotionProfileArc"=10, "Disabled"=15] ("Control Mode")
                        n77 = global read "Robot Global Data.vi" "Robot Yaw"() -> (w284:dbl)
                        n78 = Wait (ms)(milliseconds to wait=u32 50) -> ()  [unwired: 1 out]
                        n79 = global read "Robot Global Data.vi" "Robot Yaw Offset"() -> (w288:dbl)
                        n80 = call-poly <vilib>:"PID.vi"("output range"=w281, "PID gains"=w280, "process variable"=w284, "setpoint"=20.0) -> ("output"=w277:dbl)  [unwired: 6 in, 1 out]
                        n81 = Multiply(x=w277, y=-1.0) -> (x*y=w276:dbl)
                        n82 = Greater?(x=w288, y=20) -> (0:w290:bool)
                        n83 = Multiply(x=8.0 ("Output"), y=217.294) -> (x*y=w285:dbl)
                        n84 = call <vilib>:"CTRE_Phoenix_MotorControl_Set.vi"("Demand1"=w277, "DemandType"=w278, "error in (no error)"=w291, "Output"=w285, "Control Mode"=w295, "PhoenixMotorControlDevRef"=w292) -> ("error out"=w297:errorcluster, "PhoenixMotorControlDevRef"=w296:T4)  [unwired: 4 in]
                        n85 = call <vilib>:"CTRE_Phoenix_MotorControl_Set.vi"("Demand1"=w276, "DemandType"=w279, "error in (no error)"=w300, "Output"=w285, "Control Mode"=w302, "PhoenixMotorControlDevRef"=w301) -> ("error out"=w304:errorcluster, "PhoenixMotorControlDevRef"=w303:T4)  [unwired: 4 in]
                        n86 = call-poly <vilib>:"CTRE_Phoenix_MotorController_Get_Enhanced.vi"("PhoenixMotorControlDevRef"=w296, "error in"=w297) -> ("PhoenixMotorControlDevRef"=w294:T4, "error out"=w293:errorcluster)  [unwired: 8 in, 4 out]
                        n87 = call-poly <vilib>:"CTRE_Phoenix_MotorController_Get_Enhanced.vi"("PhoenixMotorControlDevRef"=w303, "error in"=w304) -> ("PhoenixMotorControlDevRef"=w299:T4, "error out"=w298:errorcluster)  [unwired: 8 in, 4 out]
                      }
                    }
                    frame #3 {
                      n88 = while {
                        tunnel: w316 -> [w341]
                        tunnel: w315 -> [w340]
                        tunnel: [w337] -> w314
                        tunnel: [w336] -> w313
                        tunnel: [w332] -> w312
                        tunnel: [w331] -> w311
                        tunnel: w310 -> [w330]
                        tunnel: w309 -> [w329]
                        tunnel: w308 -> [w321]
                        tunnel: w307 -> [w320]
                        tunnel: w306 -> [w319]
                        stop <- w338 stop-if-true
                        w333 = T14 7 items=["PercentOutput"=0, "Position"=1, "Velocity"=2, "Current"=3, "Follower"=5, "MotionProfile"=6, "MotionMagic"=7, "MotionMagicArc"=8, "MotionProfileArc"=10, "Disabled"=15] ("Control Mode")
                        w342 = T14 7 items=["PercentOutput"=0, "Position"=1, "Velocity"=2, "Current"=3, "Follower"=5, "MotionProfile"=6, "MotionMagic"=7, "MotionMagicArc"=8, "MotionProfileArc"=10, "Disabled"=15] ("Control Mode")
                        n89 = global read "Robot Global Data.vi" "Robot Travel"() -> (w339:dbl)
                        n90 = global read "Robot Global Data.vi" "Robot Yaw"() -> (w324:dbl)
                        n91 = Wait (ms)(milliseconds to wait=u32 50) -> ()  [unwired: 1 out]
                        n92 = Greater?(x=w339, y=95.5) -> (0:w338:bool)
                        n93 = call-poly <vilib>:"PID.vi"("output range"=w320, "PID gains"=w319, "process variable"=w324, "setpoint"=20.0) -> ("output"=w318:dbl)  [unwired: 6 in, 1 out]
                        n94 = Multiply(x=w318, y=-1.0) -> (x*y=w317:dbl)
                        n95 = Multiply(x=96.5 ("Output"), y=217.294) -> (x*y=w326:dbl)
                        n96 = call <vilib>:"CTRE_Phoenix_MotorControl_Set.vi"("Demand1"=w318, "error in (no error)"=w329, "Output"=w326, "Control Mode"=w333, "PhoenixMotorControlDevRef"=w330) -> ("error out"=w335:errorcluster, "PhoenixMotorControlDevRef"=w334:T4)  [unwired: 5 in]
                        n97 = call <vilib>:"CTRE_Phoenix_MotorControl_Set.vi"("Demand1"=w317, "DemandType"=w321, "error in (no error)"=w340, "Output"=w326, "Control Mode"=w342, "PhoenixMotorControlDevRef"=w341) -> ("error out"=w344:errorcluster, "PhoenixMotorControlDevRef"=w343:T4)  [unwired: 4 in]
                        n98 = call-poly <vilib>:"CTRE_Phoenix_MotorController_Get_Enhanced.vi"("PhoenixMotorControlDevRef"=w334, "error in"=w335) -> ("PhoenixMotorControlDevRef"=w332:T4, "error out"=w331:errorcluster)  [unwired: 8 in, 4 out]
                        n99 = call-poly <vilib>:"CTRE_Phoenix_MotorController_Get_Enhanced.vi"("PhoenixMotorControlDevRef"=w343, "error in"=w344) -> ("PhoenixMotorControlDevRef"=w337:T4, "error out"=w336:errorcluster)  [unwired: 8 in, 4 out]
                      }
                    }
                    frame #4 {
                      n100 = while {
                        tunnel: w356 -> [w381]
                        tunnel: w355 -> [w380]
                        tunnel: [w379] -> w354
                        tunnel: [w378] -> w353
                        tunnel: [w374] -> w352
                        tunnel: [w373] -> w351
                        tunnel: w350 -> [w372]
                        tunnel: w349 -> [w371]
                        tunnel: w348 -> [w361]
                        tunnel: w347 -> [w360]
                        tunnel: w346 -> [w359]
                        stop <- w368 stop-if-true
                        w375 = T14 7 items=["PercentOutput"=0, "Position"=1, "Velocity"=2, "Current"=3, "Follower"=5, "MotionProfile"=6, "MotionMagic"=7, "MotionMagicArc"=8, "MotionProfileArc"=10, "Disabled"=15] ("Control Mode")
                        w382 = T14 7 items=["PercentOutput"=0, "Position"=1, "Velocity"=2, "Current"=3, "Follower"=5, "MotionProfile"=6, "MotionMagic"=7, "MotionMagicArc"=8, "MotionProfileArc"=10, "Disabled"=15] ("Control Mode")
                        n101 = global read "Robot Global Data.vi" "Robot Yaw"() -> (w369:dbl)
                        n102 = global read "Robot Global Data.vi" "Robot Yaw"() -> (w364:dbl)
                        n103 = Wait (ms)(milliseconds to wait=u32 50) -> ()  [unwired: 1 out]
                        n104 = call-poly <vilib>:"PID.vi"("output range"=w360, "PID gains"=w359, "process variable"=w364, "setpoint"=0.0) -> ("output"=w358:dbl)  [unwired: 6 in, 1 out]
                        n105 = Multiply(x=w358, y=-1.0) -> (x*y=w357:dbl)
                        n106 = Less?(x=w369, y=0) -> (x < y?=w368:bool)
                        n107 = Multiply(x=96.5 ("Output"), y=217.294) -> (x*y=w365:dbl)
                        n108 = call <vilib>:"CTRE_Phoenix_MotorControl_Set.vi"("Demand1"=w358, "DemandType"=w361, "error in (no error)"=w371, "Output"=w365, "Control Mode"=w375, "PhoenixMotorControlDevRef"=w372) -> ("error out"=w377:errorcluster, "PhoenixMotorControlDevRef"=w376:T4)  [unwired: 4 in]
                        n109 = call <vilib>:"CTRE_Phoenix_MotorControl_Set.vi"("Demand1"=w357, "DemandType"=w361, "error in (no error)"=w380, "Output"=w365, "Control Mode"=w382, "PhoenixMotorControlDevRef"=w381) -> ("error out"=w384:errorcluster, "PhoenixMotorControlDevRef"=w383:T4)  [unwired: 4 in]
                        n110 = call-poly <vilib>:"CTRE_Phoenix_MotorController_Get_Enhanced.vi"("PhoenixMotorControlDevRef"=w376, "error in"=w377) -> ("PhoenixMotorControlDevRef"=w374:T4, "error out"=w373:errorcluster)  [unwired: 8 in, 4 out]
                        n111 = call-poly <vilib>:"CTRE_Phoenix_MotorController_Get_Enhanced.vi"("PhoenixMotorControlDevRef"=w383, "error in"=w384) -> ("PhoenixMotorControlDevRef"=w379:T4, "error out"=w378:errorcluster)  [unwired: 8 in, 4 out]
                      }
                    }
                    frame #5 {
                      n112 = while {
                        tunnel: w396 -> [w424]
                        tunnel: w395 -> [w423]
                        tunnel: [w420] -> w394
                        tunnel: [w419] -> w393
                        tunnel: w392 -> [w415]
                        tunnel: w391 -> [w414]
                        tunnel: [w413] -> w390
                        tunnel: [w412] -> w389
                        tunnel: w388 -> [w404]
                        tunnel: w388 -> [w403]
                        tunnel: w387 -> [w402]
                        tunnel: w386 -> [w401]
                        stop <- w421 stop-if-true
                        w416 = T14 7 items=["PercentOutput"=0, "Position"=1, "Velocity"=2, "Current"=3, "Follower"=5, "MotionProfile"=6, "MotionMagic"=7, "MotionMagicArc"=8, "MotionProfileArc"=10, "Disabled"=15] ("Control Mode")
                        w425 = T14 7 items=["PercentOutput"=0, "Position"=1, "Velocity"=2, "Current"=3, "Follower"=5, "MotionProfile"=6, "MotionMagic"=7, "MotionMagicArc"=8, "MotionProfileArc"=10, "Disabled"=15] ("Control Mode")
                        n113 = global read "Robot Global Data.vi" "Robot Travel"() -> (w422:dbl)
                        n114 = global read "Robot Global Data.vi" "Robot Yaw"() -> (w407:dbl)
                        n115 = Wait (ms)(milliseconds to wait=u32 50) -> ()  [unwired: 1 out]
                        n116 = Greater?(x=w422, y=103.5) -> (0:w421:bool)
                        n117 = global write "Robot Global Data.vi" "Elevator Bottom"(FALSE) -> ()
                        n118 = call-poly <vilib>:"PID.vi"("output range"=w401, "PID gains"=w402, "process variable"=w407, "setpoint"=0.0) -> ("output"=w400:dbl)  [unwired: 6 in, 1 out]
                        n119 = Multiply(x=w400, y=-1.0) -> (x*y=w399:dbl)
                        n120 = global write "Robot Global Data.vi" "Elevator Mid"(TRUE) -> ()
                        n121 = Multiply(x=104.5 ("Output"), y=217.294) -> (x*y=w409:dbl)
                        n122 = call <vilib>:"CTRE_Phoenix_MotorControl_Set.vi"("Demand1"=w400, "DemandType"=w403, "error in (no error)"=w414, "Output"=w409, "Control Mode"=w416, "PhoenixMotorControlDevRef"=w415) -> ("error out"=w418:errorcluster, "PhoenixMotorControlDevRef"=w417:T4)  [unwired: 4 in]
                        n123 = call <vilib>:"CTRE_Phoenix_MotorControl_Set.vi"("Demand1"=w399, "DemandType"=w404, "error in (no error)"=w423, "Output"=w409, "Control Mode"=w425, "PhoenixMotorControlDevRef"=w424) -> ("error out"=w427:errorcluster, "PhoenixMotorControlDevRef"=w426:T4)  [unwired: 4 in]
                        n124 = call-poly <vilib>:"CTRE_Phoenix_MotorController_Get_Enhanced.vi"("PhoenixMotorControlDevRef"=w417, "error in"=w418) -> ("PhoenixMotorControlDevRef"=w413:T4, "error out"=w412:errorcluster)  [unwired: 8 in, 4 out]
                        n125 = call-poly <vilib>:"CTRE_Phoenix_MotorController_Get_Enhanced.vi"("PhoenixMotorControlDevRef"=w426, "error in"=w427) -> ("PhoenixMotorControlDevRef"=w420:T4, "error out"=w419:errorcluster)  [unwired: 8 in, 4 out]
                      }
                    }
                    frame #6 {
                      n126 = while {
                        tunnel: w439 -> [w467]
                        tunnel: w438 -> [w466]
                        tunnel: [w465] -> w437
                        tunnel: [w464] -> w436
                        tunnel: w435 -> [w460]
                        tunnel: w434 -> [w459]
                        tunnel: [w458] -> w433
                        tunnel: [w457] -> w432
                        tunnel: w431 -> [w446]
                        tunnel: w431 -> [w445]
                        tunnel: w430 -> [w444]
                        tunnel: w429 -> [w443]
                        i -> [w453]
                        stop <- w454 stop-if-true
                        w461 = T14 7 items=["PercentOutput"=0, "Position"=1, "Velocity"=2, "Current"=3, "Follower"=5, "MotionProfile"=6, "MotionMagic"=7, "MotionMagicArc"=8, "MotionProfileArc"=10, "Disabled"=15] ("Control Mode")
                        w468 = T14 7 items=["PercentOutput"=0, "Position"=1, "Velocity"=2, "Current"=3, "Follower"=5, "MotionProfile"=6, "MotionMagic"=7, "MotionMagicArc"=8, "MotionProfileArc"=10, "Disabled"=15] ("Control Mode")
                        # "ADD INTAKE/ELEVATOR CODE HERE"
                        n127 = global read "Robot Global Data.vi" "Robot Yaw"() -> (w449:dbl)
                        n128 = Wait (ms)(milliseconds to wait=u32 50) -> ()  [unwired: 1 out]
                        n129 = Increment(x=w453) -> (x+1=w455:i32)
                        n130 = call-poly <vilib>:"PID.vi"("output range"=w443, "PID gains"=w444, "process variable"=w449, "setpoint"=0.0) -> ("output"=w442:dbl)  [unwired: 6 in, 1 out]
                        n131 = Multiply(x=w442, y=-1.0) -> (x*y=w441:dbl)
                        n132 = Greater Or Equal?(x=w455, y=20) -> (x >= y?=w454:bool)
                        n133 = global write "Robot Global Data.vi" "Intake Out Full"(TRUE) -> ()
                        n134 = Multiply(x=104.5 ("Output"), y=217.294) -> (x*y=w450:dbl)
                        n135 = call <vilib>:"CTRE_Phoenix_MotorControl_Set.vi"("Demand1"=w442, "DemandType"=w445, "error in (no error)"=w459, "Output"=w450, "Control Mode"=w461, "PhoenixMotorControlDevRef"=w460) -> ("error out"=w463:errorcluster, "PhoenixMotorControlDevRef"=w462:T4)  [unwired: 4 in]
                        n136 = call <vilib>:"CTRE_Phoenix_MotorControl_Set.vi"("Demand1"=w441, "DemandType"=w446, "error in (no error)"=w466, "Output"=w450, "Control Mode"=w468, "PhoenixMotorControlDevRef"=w467) -> ("error out"=w470:errorcluster, "PhoenixMotorControlDevRef"=w469:T4)  [unwired: 4 in]
                        n137 = call-poly <vilib>:"CTRE_Phoenix_MotorController_Get_Enhanced.vi"("PhoenixMotorControlDevRef"=w462, "error in"=w463) -> ("PhoenixMotorControlDevRef"=w458:T4, "error out"=w457:errorcluster)  [unwired: 8 in, 4 out]
                        n138 = call-poly <vilib>:"CTRE_Phoenix_MotorController_Get_Enhanced.vi"("PhoenixMotorControlDevRef"=w469, "error in"=w470) -> ("PhoenixMotorControlDevRef"=w465:T4, "error out"=w464:errorcluster)  [unwired: 8 in, 4 out]
                      }
                    }
                    frame #7 {
                      n139 = while {
                        tunnel: w475 -> [w488]
                        tunnel: w474 -> [w487]
                        tunnel: w473 -> [w485]
                        tunnel: w472 -> [w484]
                        i -> [w478]
                        stop <- w479 stop-if-true
                        w486 = T14 0 items=["PercentOutput"=0, "Position"=1, "Velocity"=2, "Current"=3, "Follower"=5, "MotionProfile"=6, "MotionMagic"=7, "MotionMagicArc"=8, "MotionProfileArc"=10, "Disabled"=15] ("Control Mode")
                        w489 = T14 0 items=["PercentOutput"=0, "Position"=1, "Velocity"=2, "Current"=3, "Follower"=5, "MotionProfile"=6, "MotionMagic"=7, "MotionMagicArc"=8, "MotionProfileArc"=10, "Disabled"=15] ("Control Mode")
                        n140 = Increment(x=w478) -> (x+1=w480:i32)
                        n141 = Greater Or Equal?(x=w480, y=1) -> (x >= y?=w479:bool)
                        n142 = Wait (ms)(milliseconds to wait=u32 15000) -> ()  [unwired: 1 out]
                        n143 = global write "Robot Global Data.vi" "Intake Out Full"(FALSE) -> ()
                        n144 = global write "Robot Global Data.vi" "Elevator Mid"(FALSE) -> ()
                        n145 = call <vilib>:"CTRE_Phoenix_MotorControl_Set.vi"("error in (no error)"=w484, "Output"=0.0, "Control Mode"=w486, "PhoenixMotorControlDevRef"=w485) -> ()  [unwired: 6 in, 2 out]
                        n146 = call <vilib>:"CTRE_Phoenix_MotorControl_Set.vi"("error in (no error)"=w487, "Output"=0.0, "Control Mode"=w489, "PhoenixMotorControlDevRef"=w488) -> ()  [unwired: 6 in, 2 out]
                      }
                    }
                  }
                }
                frame Default {
                }
                frame "L" {
                  # "Drive at an angle to the left side of the switch, drop cube"
                  # "Drive at an angle to the left side of the switch, drop cube"
                  n147 = flat-sequence {
                    tunnel: [w511] -> w500
                    tunnel: [w510] -> w499
                    tunnel: w492 -> [w509]
                    tunnel: w491 -> [w508]
                    tunnel: w500 -> [w532]
                    tunnel: w499 -> [w531]
                    tunnel: [w530] -> w498
                    tunnel: [w529] -> w497
                    tunnel: w498 -> [w550]
                    tunnel: w497 -> [w549]
                    tunnel: [w548] -> w496
                    tunnel: [w547] -> w495
                    tunnel: w496 -> [w568]
                    tunnel: w495 -> [w567]
                    tunnel: [w566] -> w494
                    tunnel: [w565] -> w493
                    tunnel: w494 -> [w584]
                    tunnel: w493 -> [w583]
                    frame #0 {
                      # "Initialize_Frame"
                      n148 = while {
                        i -> [w502]
                        stop <- w503 stop-if-true
                        n149 = Increment(x=w502) -> (x+1=w504:i32)
                        n150 = global write "Robot Global Data.vi" "Zero Travel"(TRUE) -> ()
                        n151 = global write "Robot Global Data.vi" "Zero Yaw"(TRUE) -> ()
                        n152 = Wait (ms)(milliseconds to wait=u32 10) -> ()  [unwired: 1 out]
                        n153 = Greater Or Equal?(x=w504, y=1) -> (x >= y?=w503:bool)
                      }
                    }
                    frame #1 {
                      n154 = while {
                        tunnel: [w520] -> w511
                        tunnel: [w519] -> w510
                        tunnel: w509 -> [w513]
                        tunnel: w508 -> [w512]
                        stop <- w525 stop-if-true
                        # "Forward"
                        n155 = global read "Robot Global Data.vi" "Robot Yaw"() -> (w517:dbl)
                        n156 = global write "Robot Global Data.vi" "Elevator Bottom"(TRUE) -> ()
                        n157 = Wait (ms)(milliseconds to wait=u32 50) -> ()  [unwired: 1 out]
                        n158 = global write "Robot Global Data.vi" "Zero Travel"(FALSE) -> ()
                        n159 = global write "Robot Global Data.vi" "Zero Yaw"(FALSE) -> ()
                        n160 = global read "Robot Global Data.vi" "Robot Travel"() -> (w526:dbl)
                        n161 = call-poly <vilib>:"PID.vi"("output range"=cluster{"output high":dbl, "output low":dbl} {"output high"=0.5, "output low"=-0.5}, "PID gains"=T1 {"proportional gain (Kc)"=1.0, "integral time (Ti, min)"=0.0, "derivative time (Td, min)"=0.0}, "process variable"=w517, "setpoint"=0.0) -> ("output"=w515:dbl)  [unwired: 6 in, 1 out]
                        n162 = call-poly <vilib>:"WPI_RobotDriveArcadeDrive.vi"("error in (no error)"=w512, "Y axis value"=-0.8, "X axis value"=w515, "RobotDriveDevRef"=w513) -> ("error out"=w519:errorcluster, "RobotDriveDevRef"=w520:T13)  [unwired: 5 in, 1 out]
                        n163 = Greater?(x=w526, y=7) -> (0:w525:bool)
                      }
                    }
                    frame #2 {
                      n164 = while {
                        tunnel: w532 -> [w541]
                        tunnel: w531 -> [w540]
                        tunnel: [w534] -> w530
                        tunnel: [w533] -> w529
                        stop <- w544 stop-if-true
                        # "Turn Left Slighly"
                        n165 = global read "Robot Global Data.vi" "Robot Yaw"() -> (w539:dbl)
                        n166 = Wait (ms)(milliseconds to wait=u32 50) -> ()  [unwired: 1 out]
                        n167 = global read "Robot Global Data.vi" "Robot Yaw"() -> (w543:dbl)
                        n168 = call-poly <vilib>:"PID.vi"("output range"=cluster{"output high":dbl, "output low":dbl} {"output high"=1.0, "output low"=-1.0}, "PID gains"=T1 {"proportional gain (Kc)"=1.0, "integral time (Ti, min)"=0.0, "derivative time (Td, min)"=0.0}, "process variable"=w539, "setpoint"=-20.0) -> ("output"=w535:dbl)  [unwired: 6 in, 1 out]
                        n169 = call-poly <vilib>:"WPI_RobotDriveArcadeDrive.vi"("error in (no error)"=w540, "Y axis value"=-0.8, "X axis value"=w535, "RobotDriveDevRef"=w541) -> ("error out"=w533:errorcluster, "RobotDriveDevRef"=w534:T13)  [unwired: 5 in, 1 out]
                        n170 = Less?(x=w543, y=-20) -> (x < y?=w544:bool)
                      }
                    }
                    frame #3 {
                      n171 = while {
                        tunnel: w550 -> [w554]
                        tunnel: w549 -> [w553]
                        tunnel: [w552] -> w548
                        tunnel: [w551] -> w547
                        stop <- w562 stop-if-true
                        # "Go Forward Again"
                        n172 = global read "Robot Global Data.vi" "Robot Travel"() -> (w563:dbl)
                        n173 = global read "Robot Global Data.vi" "Robot Yaw"() -> (w559:dbl)
                        n174 = Wait (ms)(milliseconds to wait=u32 50) -> ()  [unwired: 1 out]
                        n175 = Greater?(x=w563, y=95.5) -> (0:w562:bool)
                        n176 = call-poly <vilib>:"PID.vi"("output range"=cluster{"output high":dbl, "output low":dbl} {"output high"=1.0, "output low"=-1.0}, "PID gains"=T1 {"proportional gain (Kc)"=1.0, "integral time (Ti, min)"=0.0, "derivative time (Td, min)"=0.0}, "process variable"=w559, "setpoint"=-20.0) -> ("output"=w555:dbl)  [unwired: 6 in, 1 out]
                        n177 = call-poly <vilib>:"WPI_RobotDriveArcadeDrive.vi"("error in (no error)"=w553, "Y axis value"=-0.8, "X axis value"=w555, "RobotDriveDevRef"=w554) -> ("error out"=w551:errorcluster, "RobotDriveDevRef"=w552:T13)  [unwired: 5 in, 1 out]
                      }
                    }
                    frame #4 {
                      n178 = while {
                        tunnel: w568 -> [w572]
                        tunnel: w567 -> [w571]
                        tunnel: [w570] -> w566
                        tunnel: [w569] -> w565
                        stop <- w581 stop-if-true
                        # "Turn Slightly Right"
                        n179 = global read "Robot Global Data.vi" "Robot Yaw"() -> (w580:dbl)
                        n180 = global read "Robot Global Data.vi" "Robot Yaw"() -> (w577:dbl)
                        n181 = Wait (ms)(milliseconds to wait=u32 50) -> ()  [unwired: 1 out]
                        n182 = Greater?(x=w580, y=0) -> (0:w581:bool)
                        n183 = call-poly <vilib>:"PID.vi"("output range"=cluster{"output high":dbl, "output low":dbl} {"output high"=1.0, "output low"=-1.0}, "PID gains"=T1 {"proportional gain (Kc)"=1.0, "integral time (Ti, min)"=0.0, "derivative time (Td, min)"=0.0}, "process variable"=w577, "setpoint"=-20.0) -> ("output"=w573:dbl)  [unwired: 6 in, 1 out]
                        n184 = call-poly <vilib>:"WPI_RobotDriveArcadeDrive.vi"("error in (no error)"=w571, "Y axis value"=-0.8, "X axis value"=w573, "RobotDriveDevRef"=w572) -> ("error out"=w569:errorcluster, "RobotDriveDevRef"=w570:T13)  [unwired: 5 in, 1 out]
                      }
                    }
                    frame #5 {
                      n185 = while {
                        tunnel: w584 -> [w586]
                        tunnel: w583 -> [w585]
                        stop <- w596 stop-if-true
                        # "Roll Forward"
                        n186 = global read "Robot Global Data.vi" "Robot Travel"() -> (w597:dbl)
                        n187 = global read "Robot Global Data.vi" "Robot Yaw"() -> (w591:dbl)
                        n188 = Wait (ms)(milliseconds to wait=u32 50) -> ()  [unwired: 1 out]
                        n189 = Greater?(x=w597, y=103.5) -> (0:w596:bool)
                        n190 = global write "Robot Global Data.vi" "Elevator Bottom"(FALSE) -> ()
                        n191 = call-poly <vilib>:"PID.vi"("output range"=cluster{"output high":dbl, "output low":dbl} {"output high"=1.0, "output low"=-1.0}, "PID gains"=T1 {"proportional gain (Kc)"=1.0, "integral time (Ti, min)"=0.0, "derivative time (Td, min)"=0.0}, "process variable"=w591, "setpoint"=-20.0) -> ("output"=w587:dbl)  [unwired: 6 in, 1 out]
                        n192 = call-poly <vilib>:"WPI_RobotDriveArcadeDrive.vi"("error in (no error)"=w585, "Y axis value"=-0.8, "X axis value"=w587, "RobotDriveDevRef"=w586) -> ()  [unwired: 5 in, 3 out]
                        n193 = global write "Robot Global Data.vi" "Elevator Mid"(TRUE) -> ()
                      }
                    }
                    frame #6 {
                      n194 = while {
                        i -> [w600]
                        stop <- w601 stop-if-true
                        # "ADD INTAKE/ELEVATOR CODE HERE"
                        n195 = Increment(x=w600) -> (x+1=w602:i32)
                        n196 = Wait (ms)(milliseconds to wait=u32 50) -> ()  [unwired: 1 out]
                        n197 = Greater Or Equal?(x=w602, y=20) -> (x >= y?=w601:bool)
                        n198 = global write "Robot Global Data.vi" "Intake Out Full"(TRUE) -> ()
                      }
                    }
                    frame #7 {
                      n199 = while {
                        i -> [w607]
                        stop <- w608 stop-if-true
                        # "Reset_Frame"
                        n200 = Increment(x=w607) -> (x+1=w609:i32)
                        n201 = global write "Robot Global Data.vi" "Intake Out Full"(FALSE) -> ()
                        n202 = global write "Robot Global Data.vi" "Elevator Mid"(FALSE) -> ()
                        n203 = Wait (ms)(milliseconds to wait=u32 15000) -> ()  [unwired: 1 out]
                        n204 = Greater Or Equal?(x=w609, y=1) -> (x >= y?=w608:bool)
                      }
                    }
                  }
                }
              }
            }
            frame 2 {
              n205 = case shown="\"R\"" w631 {
                tunnel: w630 -> [w655 _ w892]
                tunnel: w629 -> [w654 _ w891]
                tunnel: w628 -> [w653 _ w890]
                tunnel: w627 -> [w652 _ w889]
                tunnel: w626 -> [w647 _ _]
                tunnel: w625 -> [w646 _ w881]
                tunnel: w624 -> [w645 _ w879]
                tunnel: w623 -> [w644 _ w877]
                tunnel: w622 -> [w643 _ w878]
                tunnel: w621 -> [w642 _ w880]
                tunnel: w620 -> [w641 _ w882]
                tunnel: w619 -> [w640 _ _]
                tunnel: w618 -> [w639 _ w885]
                tunnel: w618 -> [w638 _ w884]
                tunnel: w618 -> [w637 _ w883]
                tunnel: w618 -> [w636 _ _]
                tunnel: w618 -> [_ _ w888]
                tunnel: w618 -> [_ _ w887]
                tunnel: w618 -> [_ _ w886]
                tunnel: w617 -> [_ _ w876]
                tunnel: w616 -> [_ _ w875]
                tunnel: w615 -> [_ _ w874]
                tunnel: w614 -> [_ _ w873]
                tunnel: w613 -> [_ _ w872]
                tunnel: w612 -> [_ _ w871]
                frame "L" {
                  # "Start left. Drive forward and turn right, to place cube in switch"
                  n206 = flat-sequence {
                    tunnel: w652 -> [w668]
                    tunnel: w653 -> [w669]
                    tunnel: w654 -> [w670]
                    tunnel: w655 -> [w671]
                    tunnel: [w671] -> w635
                    tunnel: [w670] -> w634
                    tunnel: [w669] -> w633
                    tunnel: [w668] -> w632
                    tunnel: [w687] -> w667
                    tunnel: [w686] -> w666
                    tunnel: [w683] -> w665
                    tunnel: [w682] -> w664
                    tunnel: w647 -> [w681]
                    tunnel: w640 -> [w680]
                    tunnel: w636 -> [w679]
                    tunnel: w635 -> [w689]
                    tunnel: w634 -> [w688]
                    tunnel: w633 -> [w685]
                    tunnel: w632 -> [w684]
                    tunnel: w667 -> [w732]
                    tunnel: w666 -> [w731]
                    tunnel: [w730] -> w663
                    tunnel: [w729] -> w662
                    tunnel: [w728] -> w661
                    tunnel: [w727] -> w660
                    tunnel: w665 -> [w726]
                    tunnel: w664 -> [w725]
                    tunnel: w646 -> [w724]
                    tunnel: w641 -> [w723]
                    tunnel: w637 -> [w722]
                    tunnel: w663 -> [w772]
                    tunnel: w662 -> [w771]
                    tunnel: w661 -> [w770]
                    tunnel: w660 -> [w769]
                    tunnel: [w768] -> w651
                    tunnel: [w767] -> w650
                    tunnel: [w766] -> w649
                    tunnel: [w765] -> w648
                    tunnel: w645 -> [w764]
                    tunnel: w642 -> [w763]
                    tunnel: w638 -> [w762]
                    tunnel: [w814] -> w659
                    tunnel: [w813] -> w658
                    tunnel: [w812] -> w657
                    tunnel: [w811] -> w656
                    tunnel: w651 -> [w810]
                    tunnel: w650 -> [w809]
                    tunnel: w649 -> [w808]
                    tunnel: w648 -> [w807]
                    tunnel: w644 -> [w806]
                    tunnel: w643 -> [w805]
                    tunnel: w639 -> [w804]
                    tunnel: w659 -> [w849]
                    tunnel: w658 -> [w848]
                    tunnel: w657 -> [w847]
                    tunnel: w656 -> [w846]
                    frame #0 {
                      n207 = while {
                        i -> [w673]
                        stop <- w674 stop-if-true
                        n208 = Increment(x=w673) -> (x+1=w675:i32)
                        n209 = global write "Robot Global Data.vi" "Zero Travel"(TRUE) -> ()
                        n210 = global write "Robot Global Data.vi" "Zero Yaw"(TRUE) -> ()
                        n211 = Wait (ms)(milliseconds to wait=u32 10) -> ()  [unwired: 1 out]
                        n212 = Greater Or Equal?(x=w675, y=1) -> (x >= y?=w674:bool)
                      }
                    }
                    frame #1 {
                      n213 = while {
                        tunnel: w689 -> [w716]
                        tunnel: w688 -> [w715]
                        tunnel: [w714] -> w687
                        tunnel: [w713] -> w686
                        tunnel: w685 -> [w707]
                        tunnel: w684 -> [w706]
                        tunnel: [w705] -> w683
                        tunnel: [w704] -> w682
                        tunnel: w681 -> [w696]
                        tunnel: w680 -> [w695]
                        tunnel: w679 -> [w694]
                        stop <- w711 stop-if-true
                        w708 = T14 7 items=["PercentOutput"=0, "Position"=1, "Velocity"=2, "Current"=3, "Follower"=5, "MotionProfile"=6, "MotionMagic"=7, "MotionMagicArc"=8, "MotionProfileArc"=10, "Disabled"=15] ("Control Mode")
                        w717 = T14 7 items=["PercentOutput"=0, "Position"=1, "Velocity"=2, "Current"=3, "Follower"=5, "MotionProfile"=6, "MotionMagic"=7, "MotionMagicArc"=8, "MotionProfileArc"=10, "Disabled"=15] ("Control Mode")
                        n214 = global write "Robot Global Data.vi" "Elevator Bottom"(TRUE) -> ()
                        n215 = global read "Robot Global Data.vi" "Robot Yaw"() -> (w699:dbl)
                        n216 = Wait (ms)(milliseconds to wait=u32 50) -> ()  [unwired: 1 out]
                        n217 = global read "Robot Global Data.vi" "Robot Travel"() -> (w712:dbl)
                        n218 = global write "Robot Global Data.vi" "Zero Travel"(FALSE) -> ()
                        n219 = global write "Robot Global Data.vi" "Zero Yaw"(FALSE) -> ()
                        n220 = call-poly <vilib>:"PID.vi"("output range"=w696, "PID gains"=w695, "process variable"=w699, "setpoint"=0.0) -> ("output"=w692:dbl)  [unwired: 6 in, 1 out]
                        n221 = Multiply(x=w692, y=-1.0) -> (x*y=w693:dbl)
                        n222 = Greater?(x=w712, y=87.5) -> (0:w711:bool)
                        n223 = Multiply(x=88.5 ("Output"), y=217.294) -> (x*y=w701:dbl)
                        n224 = call <vilib>:"CTRE_Phoenix_MotorControl_Set.vi"("Demand1"=w693, "DemandType"=w694, "error in (no error)"=w715, "Output"=w701, "Control Mode"=w717, "PhoenixMotorControlDevRef"=w716) -> ("error out"=w719:errorcluster, "PhoenixMotorControlDevRef"=w718:T4)  [unwired: 4 in]
                        n225 = call <vilib>:"CTRE_Phoenix_MotorControl_Set.vi"("Demand1"=w692, "DemandType"=w694, "error in (no error)"=w706, "Output"=w701, "Control Mode"=w708, "PhoenixMotorControlDevRef"=w707) -> ("error out"=w710:errorcluster, "PhoenixMotorControlDevRef"=w709:T4)  [unwired: 4 in]
                        n226 = call-poly <vilib>:"CTRE_Phoenix_MotorController_Get_Enhanced.vi"("PhoenixMotorControlDevRef"=w718, "error in"=w719) -> ("PhoenixMotorControlDevRef"=w714:T4, "error out"=w713:errorcluster)  [unwired: 8 in, 4 out]
                        n227 = call-poly <vilib>:"CTRE_Phoenix_MotorController_Get_Enhanced.vi"("PhoenixMotorControlDevRef"=w709, "error in"=w710) -> ("PhoenixMotorControlDevRef"=w705:T4, "error out"=w704:errorcluster)  [unwired: 8 in, 4 out]
                      }
                    }
                    frame #2 {
                      n228 = while {
                        tunnel: w732 -> [w757]
                        tunnel: w731 -> [w756]
                        tunnel: [w755] -> w730
                        tunnel: [w754] -> w729
                        tunnel: [w750] -> w728
                        tunnel: [w749] -> w727
                        tunnel: w726 -> [w748]
                        tunnel: w725 -> [w747]
                        tunnel: w724 -> [w737]
                        tunnel: w723 -> [w736]
                        tunnel: w722 -> [w735]
                        stop <- w746 stop-if-true
                        w751 = T14 7 items=["PercentOutput"=0, "Position"=1, "Velocity"=2, "Current"=3, "Follower"=5, "MotionProfile"=6, "MotionMagic"=7, "MotionMagicArc"=8, "MotionProfileArc"=10, "Disabled"=15] ("Control Mode")
                        w758 = T14 7 items=["PercentOutput"=0, "Position"=1, "Velocity"=2, "Current"=3, "Follower"=5, "MotionProfile"=6, "MotionMagic"=7, "MotionMagicArc"=8, "MotionProfileArc"=10, "Disabled"=15] ("Control Mode")
                        n229 = global read "Robot Global Data.vi" "Robot Yaw"() -> (w740:dbl)
                        n230 = global read "Robot Global Data.vi" "Robot Yaw Offset"() -> (w744:dbl)
                        n231 = Wait (ms)(milliseconds to wait=u32 50) -> ()  [unwired: 1 out]
                        n232 = call-poly <vilib>:"PID.vi"("output range"=w737, "PID gains"=w736, "process variable"=w740, "setpoint"=90.0) -> ("output"=w733:dbl)  [unwired: 6 in, 1 out]
                        n233 = Multiply(x=w733, y=-1.0) -> (x*y=w734:dbl)
                        n234 = Greater?(x=w744, y=90) -> (0:w746:bool)
                        n235 = Multiply(x=88.5 ("Output"), y=217.294) -> (x*y=w741:dbl)
                        n236 = call <vilib>:"CTRE_Phoenix_MotorControl_Set.vi"("Demand1"=w733, "DemandType"=w735, "error in (no error)"=w747, "Output"=w741, "Control Mode"=w751, "PhoenixMotorControlDevRef"=w748) -> ("error out"=w753:errorcluster, "PhoenixMotorControlDevRef"=w752:T4)  [unwired: 4 in]
                        n237 = call <vilib>:"CTRE_Phoenix_MotorControl_Set.vi"("Demand1"=w734, "DemandType"=w735, "error in (no error)"=w756, "Output"=w741, "Control Mode"=w758, "PhoenixMotorControlDevRef"=w757) -> ("error out"=w760:errorcluster, "PhoenixMotorControlDevRef"=w759:T4)  [unwired: 4 in]
                        n238 = call-poly <vilib>:"CTRE_Phoenix_MotorController_Get_Enhanced.vi"("PhoenixMotorControlDevRef"=w752, "error in"=w753) -> ("PhoenixMotorControlDevRef"=w750:T4, "error out"=w749:errorcluster)  [unwired: 8 in, 4 out]
                        n239 = call-poly <vilib>:"CTRE_Phoenix_MotorController_Get_Enhanced.vi"("PhoenixMotorControlDevRef"=w759, "error in"=w760) -> ("PhoenixMotorControlDevRef"=w755:T4, "error out"=w754:errorcluster)  [unwired: 8 in, 4 out]
                      }
                    }
                    frame #3 {
                      n240 = while {
                        tunnel: w772 -> [w799]
                        tunnel: w771 -> [w798]
                        tunnel: [w795] -> w768
                        tunnel: [w794] -> w766
                        tunnel: [w790] -> w767
                        tunnel: [w789] -> w765
                        tunnel: w770 -> [w788]
                        tunnel: w769 -> [w787]
                        tunnel: w764 -> [w777]
                        tunnel: w763 -> [w776]
                        tunnel: w762 -> [w775]
                        stop <- w796 stop-if-true
                        w791 = T14 7 items=["PercentOutput"=0, "Position"=1, "Velocity"=2, "Current"=3, "Follower"=5, "MotionProfile"=6, "MotionMagic"=7, "MotionMagicArc"=8, "MotionProfileArc"=10, "Disabled"=15] ("Control Mode")
                        w800 = T14 7 items=["PercentOutput"=0, "Position"=1, "Velocity"=2, "Current"=3, "Follower"=5, "MotionProfile"=6, "MotionMagic"=7, "MotionMagicArc"=8, "MotionProfileArc"=10, "Disabled"=15] ("Control Mode")
                        n241 = global read "Robot Global Data.vi" "Robot Travel"() -> (w797:dbl)
                        n242 = global read "Robot Global Data.vi" "Robot Yaw"() -> (w780:dbl)
                        n243 = Wait (ms)(milliseconds to wait=u32 50) -> ()  [unwired: 1 out]
                        n244 = Greater?(x=w797, y=106) -> (0:w796:bool)
                        n245 = global write "Robot Global Data.vi" "Elevator Bottom"(FALSE) -> ()
                        n246 = call-poly <vilib>:"PID.vi"("output range"=w777, "PID gains"=w776, "process variable"=w780, "setpoint"=90.0) -> ("output"=w774:dbl)  [unwired: 6 in, 1 out]
                        n247 = Multiply(x=w774, y=-1.0) -> (x*y=w773:dbl)
                        n248 = global write "Robot Global Data.vi" "Elevator Mid"(TRUE) -> ()
                        n249 = Multiply(x=107.0 ("Output"), y=217.294) -> (x*y=w784:dbl)
                        n250 = call <vilib>:"CTRE_Phoenix_MotorControl_Set.vi"("Demand1"=w774, "DemandType"=w775, "error in (no error)"=w787, "Output"=w784, "Control Mode"=w791, "PhoenixMotorControlDevRef"=w788) -> ("error out"=w793:errorcluster, "PhoenixMotorControlDevRef"=w792:T4)  [unwired: 4 in]
                        n251 = call <vilib>:"CTRE_Phoenix_MotorControl_Set.vi"("Demand1"=w773, "DemandType"=w775, "error in (no error)"=w798, "Output"=w784, "Control Mode"=w800, "PhoenixMotorControlDevRef"=w799) -> ("error out"=w802:errorcluster, "PhoenixMotorControlDevRef"=w801:T4)  [unwired: 4 in]
                        n252 = call-poly <vilib>:"CTRE_Phoenix_MotorController_Get_Enhanced.vi"("PhoenixMotorControlDevRef"=w792, "error in"=w793) -> ("PhoenixMotorControlDevRef"=w790:T4, "error out"=w789:errorcluster)  [unwired: 8 in, 4 out]
                        n253 = call-poly <vilib>:"CTRE_Phoenix_MotorController_Get_Enhanced.vi"("PhoenixMotorControlDevRef"=w801, "error in"=w802) -> ("PhoenixMotorControlDevRef"=w795:T4, "error out"=w794:errorcluster)  [unwired: 8 in, 4 out]
                      }
                    }
                    frame #4 {
                      n254 = while {
                        tunnel: w810 -> [w841]
                        tunnel: w808 -> [w840]
                        tunnel: [w839] -> w814
                        tunnel: [w838] -> w813
                        tunnel: w809 -> [w834]
                        tunnel: w807 -> [w833]
                        tunnel: [w832] -> w812
                        tunnel: [w831] -> w811
                        tunnel: w806 -> [w819]
                        tunnel: w805 -> [w818]
                        tunnel: w804 -> [w817]
                        i -> [w827]
                        stop <- w828 stop-if-true
                        w835 = T14 7 items=["PercentOutput"=0, "Position"=1, "Velocity"=2, "Current"=3, "Follower"=5, "MotionProfile"=6, "MotionMagic"=7, "MotionMagicArc"=8, "MotionProfileArc"=10, "Disabled"=15] ("Control Mode")
                        w842 = T14 7 items=["PercentOutput"=0, "Position"=1, "Velocity"=2, "Current"=3, "Follower"=5, "MotionProfile"=6, "MotionMagic"=7, "MotionMagicArc"=8, "MotionProfileArc"=10, "Disabled"=15] ("Control Mode")
                        # "ADD INTAKE/ELEVATOR CODE HERE"
                        n255 = global read "Robot Global Data.vi" "Robot Yaw"() -> (w822:dbl)
                        n256 = Increment(x=w827) -> (x+1=w829:i32)
                        n257 = Wait (ms)(milliseconds to wait=u32 50) -> ()  [unwired: 1 out]
                        n258 = Greater Or Equal?(x=w829, y=20) -> (x >= y?=w828:bool)
                        n259 = global write "Robot Global Data.vi" "Intake Out Full"(TRUE) -> ()
                        n260 = call-poly <vilib>:"PID.vi"("output range"=w819, "PID gains"=w818, "process variable"=w822, "setpoint"=90.0) -> ("output"=w816:dbl)  [unwired: 6 in, 1 out]
                        n261 = Multiply(x=w816, y=-1.0) -> (x*y=w815:dbl)
                        n262 = Multiply(x=107.0 ("Output"), y=217.294) -> (x*y=w824:dbl)
                        n263 = call <vilib>:"CTRE_Phoenix_MotorControl_Set.vi"("Demand1"=w816, "DemandType"=w817, "error in (no error)"=w833, "Output"=w824, "Control Mode"=w835, "PhoenixMotorControlDevRef"=w834) -> ("error out"=w837:errorcluster, "PhoenixMotorControlDevRef"=w836:T4)  [unwired: 4 in]
                        n264 = call <vilib>:"CTRE_Phoenix_MotorControl_Set.vi"("Demand1"=w815, "DemandType"=w817, "error in (no error)"=w840, "Output"=w824, "Control Mode"=w842, "PhoenixMotorControlDevRef"=w841) -> ("error out"=w844:errorcluster, "PhoenixMotorControlDevRef"=w843:T4)  [unwired: 4 in]
                        n265 = call-poly <vilib>:"CTRE_Phoenix_MotorController_Get_Enhanced.vi"("PhoenixMotorControlDevRef"=w836, "error in"=w837) -> ("PhoenixMotorControlDevRef"=w832:T4, "error out"=w831:errorcluster)  [unwired: 8 in, 4 out]
                        n266 = call-poly <vilib>:"CTRE_Phoenix_MotorController_Get_Enhanced.vi"("PhoenixMotorControlDevRef"=w843, "error in"=w844) -> ("PhoenixMotorControlDevRef"=w839:T4, "error out"=w838:errorcluster)  [unwired: 8 in, 4 out]
                      }
                    }
                    frame #5 {
                      n267 = while {
                        tunnel: w849 -> [w864]
                        tunnel: w848 -> [w863]
                        tunnel: w847 -> [w861]
                        tunnel: w846 -> [w860]
                        i -> [w856]
                        stop <- w857 stop-if-true
                        w862 = T14 0 items=["PercentOutput"=0, "Position"=1, "Velocity"=2, "Current"=3, "Follower"=5, "MotionProfile"=6, "MotionMagic"=7, "MotionMagicArc"=8, "MotionProfileArc"=10, "Disabled"=15] ("Control Mode")
                        w865 = T14 0 items=["PercentOutput"=0, "Position"=1, "Velocity"=2, "Current"=3, "Follower"=5, "MotionProfile"=6, "MotionMagic"=7, "MotionMagicArc"=8, "MotionProfileArc"=10, "Disabled"=15] ("Control Mode")
                        n268 = Increment(x=w856) -> (x+1=w858:i32)
                        n269 = Wait (ms)(milliseconds to wait=u32 15000) -> ()  [unwired: 1 out]
                        n270 = Greater Or Equal?(x=w858, y=1) -> (x >= y?=w857:bool)
                        n271 = call <vilib>:"CTRE_Phoenix_MotorControl_Set.vi"("DemandType"=T2."DemandType_Neutral", "error in (no error)"=w860, "Output"=0.0, "Control Mode"=w862, "PhoenixMotorControlDevRef"=w861) -> ()  [unwired: 5 in, 2 out]
                        n272 = global write "Robot Global Data.vi" "Intake Out Full"(FALSE) -> ()
                        n273 = global write "Robot Global Data.vi" "Elevator Mid"(FALSE) -> ()
                        n274 = call <vilib>:"CTRE_Phoenix_MotorControl_Set.vi"("DemandType"=T2."DemandType_Neutral", "error in (no error)"=w863, "Output"=0.0, "Control Mode"=w865, "PhoenixMotorControlDevRef"=w864) -> ()  [unwired: 5 in, 2 out]
                      }
                    }
                  }
                }
                frame Default {
                }
                frame "R" {
                  # "Start left. Drive forward. Turn right and then turn right again to deposit cube in switch"
                  n275 = flat-sequence {
                    tunnel: w889 -> [w917]
                    tunnel: w890 -> [w918]
                    tunnel: w891 -> [w919]
                    tunnel: w892 -> [w920]
                    tunnel: [w920] -> w870
                    tunnel: [w919] -> w869
                    tunnel: [w918] -> w868
                    tunnel: [w917] -> w867
                    tunnel: [w936] -> w916
                    tunnel: [w935] -> w915
                    tunnel: [w932] -> w914
                    tunnel: [w931] -> w913
                    tunnel: w883 -> [w930]
                    tunnel: w882 -> [w929]
                    tunnel: w881 -> [w928]
                    tunnel: w870 -> [w938]
                    tunnel: w869 -> [w937]
                    tunnel: w868 -> [w934]
                    tunnel: w867 -> [w933]
                    tunnel: w916 -> [w982]
                    tunnel: w915 -> [w981]
                    tunnel: [w980] -> w912
                    tunnel: [w979] -> w911
                    tunnel: [w978] -> w910
                    tunnel: [w977] -> w909
                    tunnel: w914 -> [w976]
                    tunnel: w913 -> [w975]
                    tunnel: w884 -> [w974]
                    tunnel: w880 -> [w973]
                    tunnel: w879 -> [w972]
                    tunnel: w912 -> [w1023]
                    tunnel: w911 -> [w1022]
                    tunnel: [w1021] -> w908
                    tunnel: [w1020] -> w907
                    tunnel: [w1019] -> w906
                    tunnel: [w1018] -> w905
                    tunnel: w910 -> [w1017]
                    tunnel: w909 -> [w1016]
                    tunnel: w885 -> [w1015]
                    tunnel: w878 -> [w1014]
                    tunnel: w877 -> [w1013]
                    tunnel: w908 -> [w1064]
                    tunnel: w907 -> [w1063]
                    tunnel: [w1062] -> w904
                    tunnel: [w1061] -> w903
                    tunnel: [w1060] -> w902
                    tunnel: [w1059] -> w901
                    tunnel: w906 -> [w1058]
                    tunnel: w905 -> [w1057]
                    tunnel: w888 -> [w1056]
                    tunnel: w876 -> [w1055]
                    tunnel: w875 -> [w1054]
                    tunnel: w904 -> [w1104]
                    tunnel: w903 -> [w1103]
                    tunnel: [w1102] -> w900
                    tunnel: [w1101] -> w899
                    tunnel: w902 -> [w1100]
                    tunnel: w901 -> [w1099]
                    tunnel: [w1098] -> w898
                    tunnel: [w1097] -> w897
                    tunnel: w887 -> [w1096]
                    tunnel: w874 -> [w1095]
                    tunnel: w873 -> [w1094]
                    tunnel: w900 -> [w1147]
                    tunnel: w899 -> [w1146]
                    tunnel: [w1145] -> w896
                    tunnel: [w1144] -> w895
                    tunnel: w898 -> [w1143]
                    tunnel: w897 -> [w1142]
                    tunnel: [w1141] -> w894
                    tunnel: [w1140] -> w893
                    tunnel: w886 -> [w1139]
                    tunnel: w872 -> [w1138]
                    tunnel: w871 -> [w1137]
                    tunnel: w896 -> [w1182]
                    tunnel: w895 -> [w1181]
                    tunnel: w894 -> [w1180]
                    tunnel: w893 -> [w1179]
                    frame #0 {
                      n276 = while {
                        i -> [w922]
                        stop <- w923 stop-if-true
                        n277 = Increment(x=w922) -> (x+1=w924:i32)
                        n278 = global write "Robot Global Data.vi" "Zero Travel"(TRUE) -> ()
                        n279 = global write "Robot Global Data.vi" "Zero Yaw"(TRUE) -> ()
                        n280 = Wait (ms)(milliseconds to wait=u32 10) -> ()  [unwired: 1 out]
                        n281 = Greater Or Equal?(x=w924, y=1) -> (x >= y?=w923:bool)
                      }
                    }
                    frame #1 {
                      n282 = while {
                        tunnel: w938 -> [w966]
                        tunnel: w937 -> [w965]
                        tunnel: [w964] -> w936
                        tunnel: [w963] -> w935
                        tunnel: w934 -> [w957]
                        tunnel: w933 -> [w956]
                        tunnel: [w955] -> w932
                        tunnel: [w954] -> w931
                        tunnel: w930 -> [w946]
                        tunnel: w930 -> [w945]
                        tunnel: w929 -> [w944]
                        tunnel: w928 -> [w943]
                        stop <- w961 stop-if-true
                        w958 = T14 7 items=["PercentOutput"=0, "Position"=1, "Velocity"=2, "Current"=3, "Follower"=5, "MotionProfile"=6, "MotionMagic"=7, "MotionMagicArc"=8, "MotionProfileArc"=10, "Disabled"=15] ("Control Mode")
                        w967 = T14 7 items=["PercentOutput"=0, "Position"=1, "Velocity"=2, "Current"=3, "Follower"=5, "MotionProfile"=6, "MotionMagic"=7, "MotionMagicArc"=8, "MotionProfileArc"=10, "Disabled"=15] ("Control Mode")
                        n283 = global read "Robot Global Data.vi" "Robot Yaw"() -> (w950:dbl)
                        n284 = global write "Robot Global Data.vi" "Elevator Bottom"(TRUE) -> ()
                        n285 = global write "Robot Global Data.vi" "Zero Travel"(FALSE) -> ()
                        n286 = global write "Robot Global Data.vi" "Zero Yaw"(FALSE) -> ()
                        n287 = Wait (ms)(milliseconds to wait=u32 50) -> ()  [unwired: 1 out]
                        n288 = global read "Robot Global Data.vi" "Robot Travel"() -> (w962:dbl)
                        n289 = call-poly <vilib>:"PID.vi"("output range"=w943, "PID gains"=w944, "process variable"=w950, "setpoint"=0.0) -> ("output"=w942:dbl)  [unwired: 6 in, 1 out]
                        n290 = Multiply(x=w942, y=-1.0) -> (x*y=w941:dbl)
                        n291 = Greater?(x=w962, y=214.75) -> (0:w961:bool)
                        n292 = Multiply(x=215.75 ("Output"), y=217.294) -> (x*y=w951:dbl)
                        n293 = call <vilib>:"CTRE_Phoenix_MotorControl_Set.vi"("Demand1"=w941, "DemandType"=w946, "error in (no error)"=w965, "Output"=w951, "Control Mode"=w967, "PhoenixMotorControlDevRef"=w966) -> ("error out"=w969:errorcluster, "PhoenixMotorControlDevRef"=w968:T4)  [unwired: 4 in]
                        n294 = call <vilib>:"CTRE_Phoenix_MotorControl_Set.vi"("Demand1"=w942, "DemandType"=w945, "error in (no error)"=w956, "Output"=w951, "Control Mode"=w958, "PhoenixMotorControlDevRef"=w957) -> ("error out"=w960:errorcluster, "PhoenixMotorControlDevRef"=w959:T4)  [unwired: 4 in]
                        n295 = call-poly <vilib>:"CTRE_Phoenix_MotorController_Get_Enhanced.vi"("PhoenixMotorControlDevRef"=w968, "error in"=w969) -> ("PhoenixMotorControlDevRef"=w964:T4, "error out"=w963:errorcluster)  [unwired: 8 in, 4 out]
                        n296 = call-poly <vilib>:"CTRE_Phoenix_MotorController_Get_Enhanced.vi"("PhoenixMotorControlDevRef"=w959, "error in"=w960) -> ("PhoenixMotorControlDevRef"=w955:T4, "error out"=w954:errorcluster)  [unwired: 8 in, 4 out]
                      }
                    }
                    frame #2 {
                      n297 = while {
                        tunnel: w982 -> [w1008]
                        tunnel: w981 -> [w1007]
                        tunnel: [w1006] -> w980
                        tunnel: [w1005] -> w979
                        tunnel: [w1001] -> w978
                        tunnel: [w1000] -> w977
                        tunnel: w976 -> [w999]
                        tunnel: w975 -> [w998]
                        tunnel: w974 -> [w988]
                        tunnel: w974 -> [w987]
                        tunnel: w973 -> [w986]
                        tunnel: w972 -> [w985]
                        stop <- w997 stop-if-true
                        w1002 = T14 7 items=["PercentOutput"=0, "Position"=1, "Velocity"=2, "Current"=3, "Follower"=5, "MotionProfile"=6, "MotionMagic"=7, "MotionMagicArc"=8, "MotionProfileArc"=10, "Disabled"=15] ("Control Mode")
                        w1009 = T14 7 items=["PercentOutput"=0, "Position"=1, "Velocity"=2, "Current"=3, "Follower"=5, "MotionProfile"=6, "MotionMagic"=7, "MotionMagicArc"=8, "MotionProfileArc"=10, "Disabled"=15] ("Control Mode")
                        n298 = global read "Robot Global Data.vi" "Robot Yaw Offset"() -> (w996:dbl)
                        n299 = Wait (ms)(milliseconds to wait=u32 50) -> ()  [unwired: 1 out]
                        n300 = global read "Robot Global Data.vi" "Robot Yaw"() -> (w991:dbl)
                        n301 = call-poly <vilib>:"PID.vi"("output range"=w985, "PID gains"=w986, "process variable"=w991, "setpoint"=90.0) -> ("output"=w984:dbl)  [unwired: 6 in, 1 out]
                        n302 = Multiply(x=w984, y=-1.0) -> (x*y=w983:dbl)
                        n303 = Greater?(x=w996, y=90) -> (0:w997:bool)
                        n304 = Multiply(x=215.75 ("Output"), y=217.294) -> (x*y=w993:dbl)
                        n305 = call <vilib>:"CTRE_Phoenix_MotorControl_Set.vi"("Demand1"=w984, "DemandType"=w987, "error in (no error)"=w998, "Output"=w993, "Control Mode"=w1002, "PhoenixMotorControlDevRef"=w999) -> ("error out"=w1004:errorcluster, "PhoenixMotorControlDevRef"=w1003:T4)  [unwired: 4 in]
                        n306 = call <vilib>:"CTRE_Phoenix_MotorControl_Set.vi"("Demand1"=w983, "DemandType"=w988, "error in (no error)"=w1007, "Output"=w993, "Control Mode"=w1009, "PhoenixMotorControlDevRef"=w1008) -> ("error out"=w1011:errorcluster, "PhoenixMotorControlDevRef"=w1010:T4)  [unwired: 4 in]
                        n307 = call-poly <vilib>:"CTRE_Phoenix_MotorController_Get_Enhanced.vi"("PhoenixMotorControlDevRef"=w1003, "error in"=w1004) -> ("PhoenixMotorControlDevRef"=w1001:T4, "error out"=w1000:errorcluster)  [unwired: 8 in, 4 out]
                        n308 = call-poly <vilib>:"CTRE_Phoenix_MotorController_Get_Enhanced.vi"("PhoenixMotorControlDevRef"=w1010, "error in"=w1011) -> ("PhoenixMotorControlDevRef"=w1006:T4, "error out"=w1005:errorcluster)  [unwired: 8 in, 4 out]
                      }
                    }
                    frame #3 {
                      n309 = while {
                        tunnel: w1023 -> [w1049]
                        tunnel: w1022 -> [w1048]
                        tunnel: [w1045] -> w1021
                        tunnel: [w1044] -> w1020
                        tunnel: [w1040] -> w1019
                        tunnel: [w1039] -> w1018
                        tunnel: w1017 -> [w1038]
                        tunnel: w1016 -> [w1037]
                        tunnel: w1015 -> [w1029]
                        tunnel: w1015 -> [w1028]
                        tunnel: w1014 -> [w1027]
                        tunnel: w1013 -> [w1026]
                        stop <- w1046 stop-if-true
                        w1041 = T14 7 items=["PercentOutput"=0, "Position"=1, "Velocity"=2, "Current"=3, "Follower"=5, "MotionProfile"=6, "MotionMagic"=7, "MotionMagicArc"=8, "MotionProfileArc"=10, "Disabled"=15] ("Control Mode")
                        w1050 = T14 7 items=["PercentOutput"=0, "Position"=1, "Velocity"=2, "Current"=3, "Follower"=5, "MotionProfile"=6, "MotionMagic"=7, "MotionMagicArc"=8, "MotionProfileArc"=10, "Disabled"=15] ("Control Mode")
                        n310 = global read "Robot Global Data.vi" "Robot Travel"() -> (w1047:dbl)
                        n311 = global read "Robot Global Data.vi" "Robot Yaw"() -> (w1033:dbl)
                        n312 = Wait (ms)(milliseconds to wait=u32 50) -> ()  [unwired: 1 out]
                        n313 = Greater?(x=w1047, y=383.75) -> (0:w1046:bool)
                        n314 = call-poly <vilib>:"PID.vi"("output range"=w1026, "PID gains"=w1027, "process variable"=w1033, "setpoint"=90.0) -> ("output"=w1025:dbl)  [unwired: 6 in, 1 out]
                        n315 = Multiply(x=w1025, y=-1.0) -> (x*y=w1024:dbl)
                        n316 = Multiply(x=384.75 ("Output"), y=217.294) -> (x*y=w1034:dbl)
                        n317 = call <vilib>:"CTRE_Phoenix_MotorControl_Set.vi"("Demand1"=w1025, "DemandType"=w1028, "error in (no error)"=w1037, "Output"=w1034, "Control Mode"=w1041, "PhoenixMotorControlDevRef"=w1038) -> ("error out"=w1043:errorcluster, "PhoenixMotorControlDevRef"=w1042:T4)  [unwired: 4 in]
                        n318 = call <vilib>:"CTRE_Phoenix_MotorControl_Set.vi"("Demand1"=w1024, "DemandType"=w1029, "error in (no error)"=w1048, "Output"=w1034, "Control Mode"=w1050, "PhoenixMotorControlDevRef"=w1049) -> ("error out"=w1052:errorcluster, "PhoenixMotorControlDevRef"=w1051:T4)  [unwired: 4 in]
                        n319 = call-poly <vilib>:"CTRE_Phoenix_MotorController_Get_Enhanced.vi"("PhoenixMotorControlDevRef"=w1042, "error in"=w1043) -> ("PhoenixMotorControlDevRef"=w1040:T4, "error out"=w1039:errorcluster)  [unwired: 8 in, 4 out]
                        n320 = call-poly <vilib>:"CTRE_Phoenix_MotorController_Get_Enhanced.vi"("PhoenixMotorControlDevRef"=w1051, "error in"=w1052) -> ("PhoenixMotorControlDevRef"=w1045:T4, "error out"=w1044:errorcluster)  [unwired: 8 in, 4 out]
                      }
                    }
                    frame #4 {
                      n321 = while {
                        tunnel: w1064 -> [w1089]
                        tunnel: w1063 -> [w1088]
                        tunnel: [w1087] -> w1062
                        tunnel: [w1086] -> w1061
                        tunnel: [w1082] -> w1060
                        tunnel: [w1081] -> w1059
                        tunnel: w1058 -> [w1080]
                        tunnel: w1057 -> [w1079]
                        tunnel: w1056 -> [w1069]
                        tunnel: w1055 -> [w1068]
                        tunnel: w1054 -> [w1067]
                        stop <- w1076 stop-if-true
                        w1083 = T14 7 items=["PercentOutput"=0, "Position"=1, "Velocity"=2, "Current"=3, "Follower"=5, "MotionProfile"=6, "MotionMagic"=7, "MotionMagicArc"=8, "MotionProfileArc"=10, "Disabled"=15] ("Control Mode")
                        w1090 = T14 7 items=["PercentOutput"=0, "Position"=1, "Velocity"=2, "Current"=3, "Follower"=5, "MotionProfile"=6, "MotionMagic"=7, "MotionMagicArc"=8, "MotionProfileArc"=10, "Disabled"=15] ("Control Mode")
                        n322 = global read "Robot Global Data.vi" "Robot Yaw"() -> (w1077:dbl)
                        n323 = global read "Robot Global Data.vi" "Robot Yaw"() -> (w1072:dbl)
                        n324 = Wait (ms)(milliseconds to wait=u32 50) -> ()  [unwired: 1 out]
                        n325 = Less?(x=w1077, y=180) -> (x < y?=w1076:bool)
                        n326 = call-poly <vilib>:"PID.vi"("output range"=w1067, "PID gains"=w1068, "process variable"=w1072, "setpoint"=180.0) -> ("output"=w1066:dbl)  [unwired: 6 in, 1 out]
                        n327 = Multiply(x=w1066, y=-1.0) -> (x*y=w1065:dbl)
                        n328 = Multiply(x=384.75 ("Output"), y=217.294) -> (x*y=w1073:dbl)
                        n329 = call <vilib>:"CTRE_Phoenix_MotorControl_Set.vi"("Demand1"=w1066, "DemandType"=w1069, "error in (no error)"=w1079, "Output"=w1073, "Control Mode"=w1083, "PhoenixMotorControlDevRef"=w1080) -> ("error out"=w1085:errorcluster, "PhoenixMotorControlDevRef"=w1084:T4)  [unwired: 4 in]
                        n330 = call <vilib>:"CTRE_Phoenix_MotorControl_Set.vi"("Demand1"=w1065, "DemandType"=w1069, "error in (no error)"=w1088, "Output"=w1073, "Control Mode"=w1090, "PhoenixMotorControlDevRef"=w1089) -> ("error out"=w1092:errorcluster, "PhoenixMotorControlDevRef"=w1091:T4)  [unwired: 4 in]
                        n331 = call-poly <vilib>:"CTRE_Phoenix_MotorController_Get_Enhanced.vi"("PhoenixMotorControlDevRef"=w1084, "error in"=w1085) -> ("PhoenixMotorControlDevRef"=w1082:T4, "error out"=w1081:errorcluster)  [unwired: 8 in, 4 out]
                        n332 = call-poly <vilib>:"CTRE_Phoenix_MotorController_Get_Enhanced.vi"("PhoenixMotorControlDevRef"=w1091, "error in"=w1092) -> ("PhoenixMotorControlDevRef"=w1087:T4, "error out"=w1086:errorcluster)  [unwired: 8 in, 4 out]
                      }
                    }
                    frame #5 {
                      n333 = while {
                        tunnel: w1104 -> [w1132]
                        tunnel: w1103 -> [w1131]
                        tunnel: [w1128] -> w1102
                        tunnel: [w1127] -> w1101
                        tunnel: w1100 -> [w1123]
                        tunnel: w1099 -> [w1122]
                        tunnel: [w1121] -> w1098
                        tunnel: [w1120] -> w1097
                        tunnel: w1096 -> [w1112]
                        tunnel: w1096 -> [w1111]
                        tunnel: w1095 -> [w1108]
                        tunnel: w1094 -> [w1107]
                        stop <- w1129 stop-if-true
                        w1124 = T14 7 items=["PercentOutput"=0, "Position"=1, "Velocity"=2, "Current"=3, "Follower"=5, "MotionProfile"=6, "MotionMagic"=7, "MotionMagicArc"=8, "MotionProfileArc"=10, "Disabled"=15] ("Control Mode")
                        w1133 = T14 7 items=["PercentOutput"=0, "Position"=1, "Velocity"=2, "Current"=3, "Follower"=5, "MotionProfile"=6, "MotionMagic"=7, "MotionMagicArc"=8, "MotionProfileArc"=10, "Disabled"=15] ("Control Mode")
                        n334 = global read "Robot Global Data.vi" "Robot Travel"() -> (w1130:dbl)
                        n335 = global read "Robot Global Data.vi" "Robot Yaw"() -> (w1116:dbl)
                        n336 = Wait (ms)(milliseconds to wait=u32 50) -> ()  [unwired: 1 out]
                        n337 = Greater?(x=w1130, y=390.5) -> (0:w1129:bool)
                        n338 = global write "Robot Global Data.vi" "Elevator Bottom"(FALSE) -> ()
                        n339 = global write "Robot Global Data.vi" "Elevator Mid"(TRUE) -> ()
                        n340 = call-poly <vilib>:"PID.vi"("output range"=w1107, "PID gains"=w1108, "process variable"=w1116, "setpoint"=180.0) -> ("output"=w1106:dbl)  [unwired: 6 in, 1 out]
                        n341 = Multiply(x=w1106, y=-1.0) -> (x*y=w1105:dbl)
                        n342 = Multiply(x=391.5 ("Output"), y=217.294) -> (x*y=w1117:dbl)
                        n343 = call <vilib>:"CTRE_Phoenix_MotorControl_Set.vi"("Demand1"=w1106, "DemandType"=w1111, "error in (no error)"=w1122, "Output"=w1117, "Control Mode"=w1124, "PhoenixMotorControlDevRef"=w1123) -> ("error out"=w1126:errorcluster, "PhoenixMotorControlDevRef"=w1125:T4)  [unwired: 4 in]
                        n344 = call <vilib>:"CTRE_Phoenix_MotorControl_Set.vi"("Demand1"=w1105, "DemandType"=w1112, "error in (no error)"=w1131, "Output"=w1117, "Control Mode"=w1133, "PhoenixMotorControlDevRef"=w1132) -> ("error out"=w1135:errorcluster, "PhoenixMotorControlDevRef"=w1134:T4)  [unwired: 4 in]
                        n345 = call-poly <vilib>:"CTRE_Phoenix_MotorController_Get_Enhanced.vi"("PhoenixMotorControlDevRef"=w1125, "error in"=w1126) -> ("PhoenixMotorControlDevRef"=w1121:T4, "error out"=w1120:errorcluster)  [unwired: 8 in, 4 out]
                        n346 = call-poly <vilib>:"CTRE_Phoenix_MotorController_Get_Enhanced.vi"("PhoenixMotorControlDevRef"=w1134, "error in"=w1135) -> ("PhoenixMotorControlDevRef"=w1128:T4, "error out"=w1127:errorcluster)  [unwired: 8 in, 4 out]
                      }
                    }
                    frame #6 {
                      n347 = while {
                        tunnel: w1147 -> [w1174]
                        tunnel: w1146 -> [w1173]
                        tunnel: [w1172] -> w1145
                        tunnel: [w1171] -> w1144
                        tunnel: w1143 -> [w1167]
                        tunnel: w1142 -> [w1166]
                        tunnel: [w1165] -> w1141
                        tunnel: [w1164] -> w1140
                        tunnel: w1139 -> [w1153]
                        tunnel: w1138 -> [w1151]
                        tunnel: w1137 -> [w1150]
                        i -> [w1160]
                        stop <- w1161 stop-if-true
                        w1168 = T14 7 items=["PercentOutput"=0, "Position"=1, "Velocity"=2, "Current"=3, "Follower"=5, "MotionProfile"=6, "MotionMagic"=7, "MotionMagicArc"=8, "MotionProfileArc"=10, "Disabled"=15] ("Control Mode")
                        w1175 = T14 7 items=["PercentOutput"=0, "Position"=1, "Velocity"=2, "Current"=3, "Follower"=5, "MotionProfile"=6, "MotionMagic"=7, "MotionMagicArc"=8, "MotionProfileArc"=10, "Disabled"=15] ("Control Mode")
                        # "ADD INTAKE/ELEVATOR CODE HERE"
                        n348 = Increment(x=w1160) -> (x+1=w1162:i32)
                        n349 = global read "Robot Global Data.vi" "Robot Yaw"() -> (w1156:dbl)
                        n350 = Wait (ms)(milliseconds to wait=u32 50) -> ()  [unwired: 1 out]
                        n351 = Greater Or Equal?(x=w1162, y=20) -> (x >= y?=w1161:bool)
                        n352 = global write "Robot Global Data.vi" "Intake Out Full"(TRUE) -> ()
                        n353 = call-poly <vilib>:"PID.vi"("output range"=w1151, "PID gains"=w1150, "process variable"=w1156, "setpoint"=180.0) -> ("output"=w1149:dbl)  [unwired: 6 in, 1 out]
                        n354 = Multiply(x=w1149, y=-1.0) -> (x*y=w1148:dbl)
                        n355 = Multiply(x=391.5 ("Output"), y=217.294) -> (x*y=w1157:dbl)
                        n356 = call <vilib>:"CTRE_Phoenix_MotorControl_Set.vi"("Demand1"=w1149, "DemandType"=w1153, "error in (no error)"=w1166, "Output"=w1157, "Control Mode"=w1168, "PhoenixMotorControlDevRef"=w1167) -> ("error out"=w1170:errorcluster, "PhoenixMotorControlDevRef"=w1169:T4)  [unwired: 4 in]
                        n357 = call <vilib>:"CTRE_Phoenix_MotorControl_Set.vi"("Demand1"=w1148, "DemandType"=w1153, "error in (no error)"=w1173, "Output"=w1157, "Control Mode"=w1175, "PhoenixMotorControlDevRef"=w1174) -> ("error out"=w1177:errorcluster, "PhoenixMotorControlDevRef"=w1176:T4)  [unwired: 4 in]
                        n358 = call-poly <vilib>:"CTRE_Phoenix_MotorController_Get_Enhanced.vi"("PhoenixMotorControlDevRef"=w1169, "error in"=w1170) -> ("PhoenixMotorControlDevRef"=w1165:T4, "error out"=w1164:errorcluster)  [unwired: 8 in, 4 out]
                        n359 = call-poly <vilib>:"CTRE_Phoenix_MotorController_Get_Enhanced.vi"("PhoenixMotorControlDevRef"=w1176, "error in"=w1177) -> ("PhoenixMotorControlDevRef"=w1172:T4, "error out"=w1171:errorcluster)  [unwired: 8 in, 4 out]
                      }
                    }
                    frame #7 {
                      n360 = while {
                        tunnel: w1182 -> [w1197]
                        tunnel: w1181 -> [w1196]
                        tunnel: w1180 -> [w1194]
                        tunnel: w1179 -> [w1193]
                        i -> [w1189]
                        stop <- w1190 stop-if-true
                        w1195 = T14 0 items=["PercentOutput"=0, "Position"=1, "Velocity"=2, "Current"=3, "Follower"=5, "MotionProfile"=6, "MotionMagic"=7, "MotionMagicArc"=8, "MotionProfileArc"=10, "Disabled"=15] ("Control Mode")
                        w1198 = T14 0 items=["PercentOutput"=0, "Position"=1, "Velocity"=2, "Current"=3, "Follower"=5, "MotionProfile"=6, "MotionMagic"=7, "MotionMagicArc"=8, "MotionProfileArc"=10, "Disabled"=15] ("Control Mode")
                        n361 = Increment(x=w1189) -> (x+1=w1191:i32)
                        n362 = Wait (ms)(milliseconds to wait=u32 15000) -> ()  [unwired: 1 out]
                        n363 = call <vilib>:"CTRE_Phoenix_MotorControl_Set.vi"("DemandType"=T2."DemandType_Neutral", "error in (no error)"=w1193, "Output"=0.0, "Control Mode"=w1195, "PhoenixMotorControlDevRef"=w1194) -> ()  [unwired: 5 in, 2 out]
                        n364 = Greater Or Equal?(x=w1191, y=1) -> (x >= y?=w1190:bool)
                        n365 = global write "Robot Global Data.vi" "Intake Out Full"(FALSE) -> ()
                        n366 = global write "Robot Global Data.vi" "Elevator Mid"(FALSE) -> ()
                        n367 = call <vilib>:"CTRE_Phoenix_MotorControl_Set.vi"("DemandType"=T2."DemandType_Neutral", "error in (no error)"=w1196, "Output"=0.0, "Control Mode"=w1198, "PhoenixMotorControlDevRef"=w1197) -> ()  [unwired: 5 in, 2 out]
                      }
                    }
                  }
                }
              }
            }
            frame 3 {
              n368 = case shown="\"R\"" w1213 {
                tunnel: w1212 -> [w1232 _ w1458]
                tunnel: w1211 -> [w1231 _ w1457]
                tunnel: w1210 -> [w1230 _ w1456]
                tunnel: w1209 -> [w1229 _ w1455]
                tunnel: w1208 -> [w1220 _ w1454]
                tunnel: w1207 -> [w1228 _ _]
                tunnel: w1206 -> [w1227 _ _]
                tunnel: w1205 -> [w1226 _ _]
                tunnel: w1204 -> [w1225 _ _]
                tunnel: w1203 -> [w1224 _ _]
                tunnel: w1202 -> [w1223 _ _]
                tunnel: w1201 -> [w1222 _ _]
                tunnel: w1200 -> [w1221 _ _]
                frame "R" {
                  n369 = flat-sequence {
                    tunnel: w1221 -> [w1249]
                    tunnel: w1222 -> [w1250]
                    tunnel: w1229 -> [w1251]
                    tunnel: w1230 -> [w1252]
                    tunnel: w1231 -> [w1253]
                    tunnel: w1232 -> [w1254]
                    tunnel: [w1254] -> w1219
                    tunnel: [w1253] -> w1218
                    tunnel: [w1252] -> w1217
                    tunnel: [w1251] -> w1216
                    tunnel: [w1250] -> w1215
                    tunnel: [w1249] -> w1214
                    tunnel: [w1270] -> w1248
                    tunnel: [w1269] -> w1247
                    tunnel: [w1266] -> w1246
                    tunnel: [w1265] -> w1245
                    tunnel: w1220 -> [w1262]
                    tunnel: w1219 -> [w1272]
                    tunnel: w1218 -> [w1271]
                    tunnel: w1217 -> [w1268]
                    tunnel: w1216 -> [w1267]
                    tunnel: w1215 -> [w1264]
                    tunnel: w1214 -> [w1263]
                    tunnel: w1248 -> [w1315]
                    tunnel: w1247 -> [w1314]
                    tunnel: [w1313] -> w1244
                    tunnel: [w1312] -> w1243
                    tunnel: [w1311] -> w1242
                    tunnel: [w1310] -> w1241
                    tunnel: w1246 -> [w1309]
                    tunnel: w1245 -> [w1308]
                    tunnel: w1224 -> [w1307]
                    tunnel: w1223 -> [w1306]
                    tunnel: w1220 -> [w1305]
                    tunnel: w1244 -> [w1355]
                    tunnel: w1243 -> [w1354]
                    tunnel: w1242 -> [w1353]
                    tunnel: w1241 -> [w1352]
                    tunnel: [w1351] -> w1240
                    tunnel: [w1350] -> w1239
                    tunnel: [w1349] -> w1238
                    tunnel: [w1348] -> w1237
                    tunnel: w1226 -> [w1347]
                    tunnel: w1225 -> [w1346]
                    tunnel: w1220 -> [w1345]
                    tunnel: [w1397] -> w1236
                    tunnel: [w1396] -> w1235
                    tunnel: [w1395] -> w1234
                    tunnel: [w1394] -> w1233
                    tunnel: w1240 -> [w1393]
                    tunnel: w1239 -> [w1392]
                    tunnel: w1238 -> [w1391]
                    tunnel: w1237 -> [w1390]
                    tunnel: w1228 -> [w1389]
                    tunnel: w1227 -> [w1388]
                    tunnel: w1220 -> [w1387]
                    tunnel: w1236 -> [w1432]
                    tunnel: w1235 -> [w1431]
                    tunnel: w1234 -> [w1430]
                    tunnel: w1233 -> [w1429]
                    frame #0 {
                      n370 = while {
                        i -> [w1256]
                        stop <- w1257 stop-if-true
                        n371 = Increment(x=w1256) -> (x+1=w1258:i32)
                        n372 = global write "Robot Global Data.vi" "Zero Travel"(TRUE) -> ()
                        n373 = global write "Robot Global Data.vi" "Zero Yaw"(TRUE) -> ()
                        n374 = Wait (ms)(milliseconds to wait=u32 10) -> ()  [unwired: 1 out]
                        n375 = Greater Or Equal?(x=w1258, y=1) -> (x >= y?=w1257:bool)
                      }
                    }
                    frame #1 {
                      n376 = while {
                        tunnel: w1272 -> [w1299]
                        tunnel: w1271 -> [w1298]
                        tunnel: [w1297] -> w1270
                        tunnel: [w1296] -> w1269
                        tunnel: w1268 -> [w1290]
                        tunnel: w1267 -> [w1289]
                        tunnel: [w1288] -> w1266
                        tunnel: [w1287] -> w1265
                        tunnel: w1264 -> [w1279]
                        tunnel: w1263 -> [w1278]
                        tunnel: w1262 -> [w1277]
                        stop <- w1294 stop-if-true
                        w1291 = T14 7 items=["PercentOutput"=0, "Position"=1, "Velocity"=2, "Current"=3, "Follower"=5, "MotionProfile"=6, "MotionMagic"=7, "MotionMagicArc"=8, "MotionProfileArc"=10, "Disabled"=15] ("Control Mode")
                        w1300 = T14 7 items=["PercentOutput"=0, "Position"=1, "Velocity"=2, "Current"=3, "Follower"=5, "MotionProfile"=6, "MotionMagic"=7, "MotionMagicArc"=8, "MotionProfileArc"=10, "Disabled"=15] ("Control Mode")
                        n377 = global read "Robot Global Data.vi" "Robot Yaw"() -> (w1283:dbl)
                        n378 = global write "Robot Global Data.vi" "Elevator Bottom"(TRUE) -> ()
                        n379 = Wait (ms)(milliseconds to wait=u32 50) -> ()  [unwired: 1 out]
                        n380 = global read "Robot Global Data.vi" "Robot Travel"() -> (w1295:dbl)
                        n381 = global write "Robot Global Data.vi" "Zero Travel"(FALSE) -> ()
                        n382 = global write "Robot Global Data.vi" "Zero Yaw"(FALSE) -> ()
                        n383 = call-poly <vilib>:"PID.vi"("output range"=w1279, "PID gains"=w1278, "process variable"=w1283, "setpoint"=0.0) -> ("output"=w1275:dbl)  [unwired: 6 in, 1 out]
                        n384 = Multiply(x=w1275, y=-1.0) -> (x*y=w1276:dbl)
                        n385 = Greater?(x=w1295, y=87.5) -> (0:w1294:bool)
                        n386 = Multiply(x=88.5 ("Output"), y=217.294) -> (x*y=w1284:dbl)
                        n387 = call <vilib>:"CTRE_Phoenix_MotorControl_Set.vi"("Demand1"=w1276, "DemandType"=w1277, "error in (no error)"=w1298, "Output"=w1284, "Control Mode"=w1300, "PhoenixMotorControlDevRef"=w1299) -> ("error out"=w1302:errorcluster, "PhoenixMotorControlDevRef"=w1301:T4)  [unwired: 4 in]
                        n388 = call <vilib>:"CTRE_Phoenix_MotorControl_Set.vi"("Demand1"=w1275, "DemandType"=w1277, "error in (no error)"=w1289, "Output"=w1284, "Control Mode"=w1291, "PhoenixMotorControlDevRef"=w1290) -> ("error out"=w1293:errorcluster, "PhoenixMotorControlDevRef"=w1292:T4)  [unwired: 4 in]
                        n389 = call-poly <vilib>:"CTRE_Phoenix_MotorController_Get_Enhanced.vi"("PhoenixMotorControlDevRef"=w1301, "error in"=w1302) -> ("PhoenixMotorControlDevRef"=w1297:T4, "error out"=w1296:errorcluster)  [unwired: 8 in, 4 out]
                        n390 = call-poly <vilib>:"CTRE_Phoenix_MotorController_Get_Enhanced.vi"("PhoenixMotorControlDevRef"=w1292, "error in"=w1293) -> ("PhoenixMotorControlDevRef"=w1288:T4, "error out"=w1287:errorcluster)  [unwired: 8 in, 4 out]
                      }
                    }
                    frame #2 {
                      n391 = while {
                        tunnel: w1315 -> [w1340]
                        tunnel: w1314 -> [w1339]
                        tunnel: [w1338] -> w1313
                        tunnel: [w1337] -> w1312
                        tunnel: [w1333] -> w1311
                        tunnel: [w1332] -> w1310
                        tunnel: w1309 -> [w1331]
                        tunnel: w1308 -> [w1330]
                        tunnel: w1307 -> [w1320]
                        tunnel: w1306 -> [w1319]
                        tunnel: w1305 -> [w1318]
                        stop <- w1328 stop-if-true
                        w1334 = T14 7 items=["PercentOutput"=0, "Position"=1, "Velocity"=2, "Current"=3, "Follower"=5, "MotionProfile"=6, "MotionMagic"=7, "MotionMagicArc"=8, "MotionProfileArc"=10, "Disabled"=15] ("Control Mode")
                        w1341 = T14 7 items=["PercentOutput"=0, "Position"=1, "Velocity"=2, "Current"=3, "Follower"=5, "MotionProfile"=6, "MotionMagic"=7, "MotionMagicArc"=8, "MotionProfileArc"=10, "Disabled"=15] ("Control Mode")
                        n392 = global read "Robot Global Data.vi" "Robot Yaw"() -> (w1324:dbl)
                        n393 = Wait (ms)(milliseconds to wait=u32 50) -> ()  [unwired: 1 out]
                        n394 = global read "Robot Global Data.vi" "Robot Yaw"() -> (w1329:dbl)
                        n395 = call-poly <vilib>:"PID.vi"("output range"=w1320, "PID gains"=w1319, "process variable"=w1324, "setpoint"=-90.0) -> ("output"=w1316:dbl)  [unwired: 6 in, 1 out]
                        n396 = Multiply(x=w1316, y=-1.0) -> (x*y=w1317:dbl)
                        n397 = Less?(x=w1329, y=-90.0) -> (x < y?=w1328:bool)
                        n398 = Multiply(x=88.5 ("Output"), y=217.294) -> (x*y=w1325:dbl)
                        n399 = call <vilib>:"CTRE_Phoenix_MotorControl_Set.vi"("Demand1"=w1316, "DemandType"=w1318, "error in (no error)"=w1330, "Output"=w1325, "Control Mode"=w1334, "PhoenixMotorControlDevRef"=w1331) -> ("error out"=w1336:errorcluster, "PhoenixMotorControlDevRef"=w1335:T4)  [unwired: 4 in]
                        n400 = call <vilib>:"CTRE_Phoenix_MotorControl_Set.vi"("Demand1"=w1317, "DemandType"=w1318, "error in (no error)"=w1339, "Output"=w1325, "Control Mode"=w1341, "PhoenixMotorControlDevRef"=w1340) -> ("error out"=w1343:errorcluster, "PhoenixMotorControlDevRef"=w1342:T4)  [unwired: 4 in]
                        n401 = call-poly <vilib>:"CTRE_Phoenix_MotorController_Get_Enhanced.vi"("PhoenixMotorControlDevRef"=w1335, "error in"=w1336) -> ("PhoenixMotorControlDevRef"=w1333:T4, "error out"=w1332:errorcluster)  [unwired: 8 in, 4 out]
                        n402 = call-poly <vilib>:"CTRE_Phoenix_MotorController_Get_Enhanced.vi"("PhoenixMotorControlDevRef"=w1342, "error in"=w1343) -> ("PhoenixMotorControlDevRef"=w1338:T4, "error out"=w1337:errorcluster)  [unwired: 8 in, 4 out]
                      }
                    }
                    frame #3 {
                      n403 = while {
                        tunnel: w1355 -> [w1382]
                        tunnel: w1354 -> [w1381]
                        tunnel: [w1378] -> w1351
                        tunnel: [w1377] -> w1349
                        tunnel: [w1373] -> w1350
                        tunnel: [w1372] -> w1348
                        tunnel: w1353 -> [w1371]
                        tunnel: w1352 -> [w1370]
                        tunnel: w1347 -> [w1362]
                        tunnel: w1346 -> [w1361]
                        tunnel: w1345 -> [w1360]
                        stop <- w1379 stop-if-true
                        w1374 = T14 7 items=["PercentOutput"=0, "Position"=1, "Velocity"=2, "Current"=3, "Follower"=5, "MotionProfile"=6, "MotionMagic"=7, "MotionMagicArc"=8, "MotionProfileArc"=10, "Disabled"=15] ("Control Mode")
                        w1383 = T14 7 items=["PercentOutput"=0, "Position"=1, "Velocity"=2, "Current"=3, "Follower"=5, "MotionProfile"=6, "MotionMagic"=7, "MotionMagicArc"=8, "MotionProfileArc"=10, "Disabled"=15] ("Control Mode")
                        n404 = global read "Robot Global Data.vi" "Robot Travel"() -> (w1380:dbl)
                        n405 = global read "Robot Global Data.vi" "Robot Yaw"() -> (w1366:dbl)
                        n406 = Wait (ms)(milliseconds to wait=u32 50) -> ()  [unwired: 1 out]
                        n407 = Greater?(x=w1380, y=87.5) -> (0:w1379:bool)
                        n408 = global write "Robot Global Data.vi" "Elevator Bottom"(FALSE) -> ()
                        n409 = global write "Robot Global Data.vi" "Elevator Mid"(TRUE) -> ()
                        n410 = call-poly <vilib>:"PID.vi"("output range"=w1362, "PID gains"=w1361, "process variable"=w1366, "setpoint"=-90.0) -> ("output"=w1358:dbl)  [unwired: 6 in, 1 out]
                        n411 = Multiply(x=w1358, y=-1.0) -> (x*y=w1359:dbl)
                        n412 = Multiply(x=107.0 ("Output"), y=217.294) -> (x*y=w1367:dbl)
                        n413 = call <vilib>:"CTRE_Phoenix_MotorControl_Set.vi"("Demand1"=w1358, "DemandType"=w1360, "error in (no error)"=w1370, "Output"=w1367, "Control Mode"=w1374, "PhoenixMotorControlDevRef"=w1371) -> ("error out"=w1376:errorcluster, "PhoenixMotorControlDevRef"=w1375:T4)  [unwired: 4 in]
                        n414 = call <vilib>:"CTRE_Phoenix_MotorControl_Set.vi"("Demand1"=w1359, "DemandType"=w1360, "error in (no error)"=w1381, "Output"=w1367, "Control Mode"=w1383, "PhoenixMotorControlDevRef"=w1382) -> ("error out"=w1385:errorcluster, "PhoenixMotorControlDevRef"=w1384:T4)  [unwired: 4 in]
                        n415 = call-poly <vilib>:"CTRE_Phoenix_MotorController_Get_Enhanced.vi"("PhoenixMotorControlDevRef"=w1375, "error in"=w1376) -> ("PhoenixMotorControlDevRef"=w1373:T4, "error out"=w1372:errorcluster)  [unwired: 8 in, 4 out]
                        n416 = call-poly <vilib>:"CTRE_Phoenix_MotorController_Get_Enhanced.vi"("PhoenixMotorControlDevRef"=w1384, "error in"=w1385) -> ("PhoenixMotorControlDevRef"=w1378:T4, "error out"=w1377:errorcluster)  [unwired: 8 in, 4 out]
                      }
                    }
                    frame #4 {
                      n417 = while {
                        tunnel: w1393 -> [w1424]
                        tunnel: w1391 -> [w1423]
                        tunnel: [w1422] -> w1397
                        tunnel: [w1421] -> w1396
                        tunnel: w1392 -> [w1417]
                        tunnel: w1390 -> [w1416]
                        tunnel: [w1415] -> w1395
                        tunnel: [w1414] -> w1394
                        tunnel: w1389 -> [w1403]
                        tunnel: w1388 -> [w1402]
                        tunnel: w1387 -> [w1401]
                        i -> [w1411]
                        stop <- w1410 stop-if-true
                        w1418 = T14 7 items=["PercentOutput"=0, "Position"=1, "Velocity"=2, "Current"=3, "Follower"=5, "MotionProfile"=6, "MotionMagic"=7, "MotionMagicArc"=8, "MotionProfileArc"=10, "Disabled"=15] ("Control Mode")
                        w1425 = T14 7 items=["PercentOutput"=0, "Position"=1, "Velocity"=2, "Current"=3, "Follower"=5, "MotionProfile"=6, "MotionMagic"=7, "MotionMagicArc"=8, "MotionProfileArc"=10, "Disabled"=15] ("Control Mode")
                        # "ADD INTAKE/ELEVATOR CODE HERE"
                        n418 = global read "Robot Global Data.vi" "Robot Yaw"() -> (w1406:dbl)
                        n419 = Increment(x=w1411) -> (x+1=w1412:i32)
                        n420 = Wait (ms)(milliseconds to wait=u32 50) -> ()  [unwired: 1 out]
                        n421 = Greater Or Equal?(x=w1412, y=20) -> (x >= y?=w1410:bool)
                        n422 = global write "Robot Global Data.vi" "Intake Out Full"(TRUE) -> ()
                        n423 = call-poly <vilib>:"PID.vi"("output range"=w1403, "PID gains"=w1402, "process variable"=w1406, "setpoint"=-90.0) -> ("output"=w1399:dbl)  [unwired: 6 in, 1 out]
                        n424 = Multiply(x=w1399, y=-1.0) -> (x*y=w1400:dbl)
                        n425 = Multiply(x=107.0 ("Output"), y=217.294) -> (x*y=w1407:dbl)
                        n426 = call <vilib>:"CTRE_Phoenix_MotorControl_Set.vi"("Demand1"=w1399, "DemandType"=w1401, "error in (no error)"=w1416, "Output"=w1407, "Control Mode"=w1418, "PhoenixMotorControlDevRef"=w1417) -> ("error out"=w1420:errorcluster, "PhoenixMotorControlDevRef"=w1419:T4)  [unwired: 4 in]
                        n427 = call <vilib>:"CTRE_Phoenix_MotorControl_Set.vi"("Demand1"=w1400, "DemandType"=w1401, "error in (no error)"=w1423, "Output"=w1407, "Control Mode"=w1425, "PhoenixMotorControlDevRef"=w1424) -> ("error out"=w1427:errorcluster, "PhoenixMotorControlDevRef"=w1426:T4)  [unwired: 4 in]
                        n428 = call-poly <vilib>:"CTRE_Phoenix_MotorController_Get_Enhanced.vi"("PhoenixMotorControlDevRef"=w1419, "error in"=w1420) -> ("PhoenixMotorControlDevRef"=w1415:T4, "error out"=w1414:errorcluster)  [unwired: 8 in, 4 out]
                        n429 = call-poly <vilib>:"CTRE_Phoenix_MotorController_Get_Enhanced.vi"("PhoenixMotorControlDevRef"=w1426, "error in"=w1427) -> ("PhoenixMotorControlDevRef"=w1422:T4, "error out"=w1421:errorcluster)  [unwired: 8 in, 4 out]
                      }
                    }
                    frame #5 {
                      n430 = while {
                        tunnel: w1432 -> [w1447]
                        tunnel: w1431 -> [w1446]
                        tunnel: w1430 -> [w1444]
                        tunnel: w1429 -> [w1443]
                        i -> [w1439]
                        stop <- w1440 stop-if-true
                        w1445 = T14 0 items=["PercentOutput"=0, "Position"=1, "Velocity"=2, "Current"=3, "Follower"=5, "MotionProfile"=6, "MotionMagic"=7, "MotionMagicArc"=8, "MotionProfileArc"=10, "Disabled"=15] ("Control Mode")
                        w1448 = T14 0 items=["PercentOutput"=0, "Position"=1, "Velocity"=2, "Current"=3, "Follower"=5, "MotionProfile"=6, "MotionMagic"=7, "MotionMagicArc"=8, "MotionProfileArc"=10, "Disabled"=15] ("Control Mode")
                        n431 = Increment(x=w1439) -> (x+1=w1441:i32)
                        n432 = Wait (ms)(milliseconds to wait=u32 15000) -> ()  [unwired: 1 out]
                        n433 = global write "Robot Global Data.vi" "Intake Out Full"(FALSE) -> ()
                        n434 = global write "Robot Global Data.vi" "Elevator Mid"(FALSE) -> ()
                        n435 = call <vilib>:"CTRE_Phoenix_MotorControl_Set.vi"("DemandType"=T2."DemandType_Neutral", "error in (no error)"=w1443, "Output"=0.0, "Control Mode"=w1445, "PhoenixMotorControlDevRef"=w1444) -> ()  [unwired: 5 in, 2 out]
                        n436 = Greater Or Equal?(x=w1441, y=1) -> (x >= y?=w1440:bool)
                        n437 = call <vilib>:"CTRE_Phoenix_MotorControl_Set.vi"("DemandType"=T2."DemandType_Neutral", "error in (no error)"=w1446, "Output"=0.0, "Control Mode"=w1448, "PhoenixMotorControlDevRef"=w1447) -> ()  [unwired: 5 in, 2 out]
                      }
                    }
                  }
                }
                frame Default {
                }
                frame "L" {
                  n438 = flat-sequence {
                    tunnel: w1455 -> [w1483]
                    tunnel: w1457 -> [w1484]
                    tunnel: w1456 -> [w1485]
                    tunnel: w1458 -> [w1486]
                    tunnel: [w1486] -> w1453
                    tunnel: [w1485] -> w1452
                    tunnel: [w1484] -> w1451
                    tunnel: [w1483] -> w1450
                    tunnel: [w1501] -> w1482
                    tunnel: [w1500] -> w1481
                    tunnel: [w1498] -> w1480
                    tunnel: [w1497] -> w1479
                    tunnel: w1454 -> [w1494]
                    tunnel: w1453 -> [w1502]
                    tunnel: w1452 -> [w1499]
                    tunnel: w1451 -> [w1496]
                    tunnel: w1450 -> [w1495]
                    tunnel: w1482 -> [w1541]
                    tunnel: w1481 -> [w1540]
                    tunnel: [w1539] -> w1478
                    tunnel: [w1538] -> w1477
                    tunnel: [w1537] -> w1476
                    tunnel: [w1536] -> w1475
                    tunnel: w1480 -> [w1535]
                    tunnel: w1479 -> [w1534]
                    tunnel: w1454 -> [w1533]
                    tunnel: w1478 -> [w1577]
                    tunnel: w1477 -> [w1576]
                    tunnel: [w1575] -> w1474
                    tunnel: [w1574] -> w1473
                    tunnel: [w1573] -> w1472
                    tunnel: [w1572] -> w1471
                    tunnel: w1476 -> [w1571]
                    tunnel: w1475 -> [w1570]
                    tunnel: w1454 -> [w1569]
                    tunnel: w1474 -> [w1613]
                    tunnel: w1473 -> [w1612]
                    tunnel: [w1611] -> w1470
                    tunnel: [w1610] -> w1469
                    tunnel: [w1609] -> w1468
                    tunnel: [w1608] -> w1467
                    tunnel: w1472 -> [w1607]
                    tunnel: w1471 -> [w1606]
                    tunnel: w1454 -> [w1605]
                    tunnel: w1470 -> [w1649]
                    tunnel: w1469 -> [w1648]
                    tunnel: [w1647] -> w1466
                    tunnel: [w1646] -> w1465
                    tunnel: w1468 -> [w1645]
                    tunnel: w1467 -> [w1644]
                    tunnel: [w1643] -> w1464
                    tunnel: [w1642] -> w1463
                    tunnel: w1454 -> [w1641]
                    tunnel: w1466 -> [w1687]
                    tunnel: w1465 -> [w1686]
                    tunnel: [w1685] -> w1462
                    tunnel: [w1684] -> w1461
                    tunnel: w1464 -> [w1683]
                    tunnel: w1463 -> [w1682]
                    tunnel: [w1681] -> w1460
                    tunnel: [w1680] -> w1459
                    tunnel: w1454 -> [w1679]
                    tunnel: w1462 -> [w1720]
                    tunnel: w1461 -> [w1719]
                    tunnel: w1460 -> [w1718]
                    tunnel: w1459 -> [w1717]
                    frame #0 {
                      n439 = while {
                        i -> [w1488]
                        stop <- w1489 stop-if-true
                        n440 = Increment(x=w1488) -> (x+1=w1490:i32)
                        n441 = global write "Robot Global Data.vi" "Zero Travel"(TRUE) -> ()
                        n442 = global write "Robot Global Data.vi" "Zero Yaw"(TRUE) -> ()
                        n443 = Wait (ms)(milliseconds to wait=u32 10) -> ()  [unwired: 1 out]
                        n444 = Greater Or Equal?(x=w1490, y=1) -> (x >= y?=w1489:bool)
                      }
                    }
                    frame #1 {
                      n445 = while {
                        tunnel: w1502 -> [w1527]
                        tunnel: w1496 -> [w1526]
                        tunnel: [w1525] -> w1501
                        tunnel: [w1524] -> w1500
                        tunnel: w1499 -> [w1518]
                        tunnel: w1495 -> [w1517]
                        tunnel: [w1516] -> w1498
                        tunnel: [w1515] -> w1497
                        tunnel: w1494 -> [w1507]
                        stop <- w1522 stop-if-true
                        w1519 = T14 7 items=["PercentOutput"=0, "Position"=1, "Velocity"=2, "Current"=3, "Follower"=5, "MotionProfile"=6, "MotionMagic"=7, "MotionMagicArc"=8, "MotionProfileArc"=10, "Disabled"=15] ("Control Mode")
                        w1528 = T14 7 items=["PercentOutput"=0, "Position"=1, "Velocity"=2, "Current"=3, "Follower"=5, "MotionProfile"=6, "MotionMagic"=7, "MotionMagicArc"=8, "MotionProfileArc"=10, "Disabled"=15] ("Control Mode")
                        n446 = global read "Robot Global Data.vi" "Robot Yaw"() -> (w1511:dbl)
                        n447 = global write "Robot Global Data.vi" "Elevator Bottom"(TRUE) -> ()
                        n448 = Wait (ms)(milliseconds to wait=u32 50) -> ()  [unwired: 1 out]
                        n449 = global read "Robot Global Data.vi" "Robot Travel"() -> (w1523:dbl)
                        n450 = call-poly <vilib>:"PID.vi"("process variable"=w1511, "setpoint"=0.0) -> ("output"=w1505:dbl)  [unwired: 8 in, 1 out]
                        n451 = Multiply(x=w1505, y=-1.0) -> (x*y=w1506:dbl)
                        n452 = global write "Robot Global Data.vi" "Zero Travel"(FALSE) -> ()
                        n453 = global write "Robot Global Data.vi" "Zero Yaw"(FALSE) -> ()
                        n454 = Greater?(x=w1523, y=214.75) -> (0:w1522:bool)
                        n455 = Multiply(x=215.75 ("Output"), y=217.294) -> (x*y=w1512:dbl)
                        n456 = call <vilib>:"CTRE_Phoenix_MotorControl_Set.vi"("Demand1"=w1506, "DemandType"=w1507, "error in (no error)"=w1526, "Output"=w1512, "Control Mode"=w1528, "PhoenixMotorControlDevRef"=w1527) -> ("error out"=w1530:errorcluster, "PhoenixMotorControlDevRef"=w1529:T4)  [unwired: 4 in]
                        n457 = call <vilib>:"CTRE_Phoenix_MotorControl_Set.vi"("Demand1"=w1505, "DemandType"=w1507, "error in (no error)"=w1517, "Output"=w1512, "Control Mode"=w1519, "PhoenixMotorControlDevRef"=w1518) -> ("error out"=w1521:errorcluster, "PhoenixMotorControlDevRef"=w1520:T4)  [unwired: 4 in]
                        n458 = call-poly <vilib>:"CTRE_Phoenix_MotorController_Get_Enhanced.vi"("PhoenixMotorControlDevRef"=w1529, "error in"=w1530) -> ("PhoenixMotorControlDevRef"=w1525:T4, "error out"=w1524:errorcluster)  [unwired: 8 in, 4 out]
                        n459 = call-poly <vilib>:"CTRE_Phoenix_MotorController_Get_Enhanced.vi"("PhoenixMotorControlDevRef"=w1520, "error in"=w1521) -> ("PhoenixMotorControlDevRef"=w1516:T4, "error out"=w1515:errorcluster)  [unwired: 8 in, 4 out]
                      }
                    }
                    frame #2 {
                      n460 = while {
                        tunnel: w1541 -> [w1564]
                        tunnel: w1540 -> [w1563]
                        tunnel: [w1562] -> w1539
                        tunnel: [w1561] -> w1538
                        tunnel: [w1557] -> w1537
                        tunnel: [w1556] -> w1536
                        tunnel: w1535 -> [w1555]
                        tunnel: w1534 -> [w1554]
                        tunnel: w1533 -> [w1544]
                        stop <- w1552 stop-if-true
                        w1558 = T14 7 items=["PercentOutput"=0, "Position"=1, "Velocity"=2, "Current"=3, "Follower"=5, "MotionProfile"=6, "MotionMagic"=7, "MotionMagicArc"=8, "MotionProfileArc"=10, "Disabled"=15] ("Control Mode")
                        w1565 = T14 7 items=["PercentOutput"=0, "Position"=1, "Velocity"=2, "Current"=3, "Follower"=5, "MotionProfile"=6, "MotionMagic"=7, "MotionMagicArc"=8, "MotionProfileArc"=10, "Disabled"=15] ("Control Mode")
                        n461 = global read "Robot Global Data.vi" "Robot Yaw"() -> (w1547:dbl)
                        n462 = Wait (ms)(milliseconds to wait=u32 50) -> ()  [unwired: 1 out]
                        n463 = global read "Robot Global Data.vi" "Robot Yaw"() -> (w1553:dbl)
                        n464 = call-poly <vilib>:"PID.vi"("process variable"=w1547, "setpoint"=-90.0) -> ("output"=w1542:dbl)  [unwired: 8 in, 1 out]
                        n465 = Multiply(x=w1542, y=-1.0) -> (x*y=w1543:dbl)
                        n466 = Less?(x=w1553, y=-90) -> (x < y?=w1552:bool)
                        n467 = Multiply(x=215.75 ("Output"), y=217.294) -> (x*y=w1548:dbl)
                        n468 = call <vilib>:"CTRE_Phoenix_MotorControl_Set.vi"("Demand1"=w1542, "DemandType"=w1544, "error in (no error)"=w1554, "Output"=w1548, "Control Mode"=w1558, "PhoenixMotorControlDevRef"=w1555) -> ("error out"=w1560:errorcluster, "PhoenixMotorControlDevRef"=w1559:T4)  [unwired: 4 in]
                        n469 = call <vilib>:"CTRE_Phoenix_MotorControl_Set.vi"("Demand1"=w1543, "DemandType"=w1544, "error in (no error)"=w1563, "Output"=w1548, "Control Mode"=w1565, "PhoenixMotorControlDevRef"=w1564) -> ("error out"=w1567:errorcluster, "PhoenixMotorControlDevRef"=w1566:T4)  [unwired: 4 in]
                        n470 = call-poly <vilib>:"CTRE_Phoenix_MotorController_Get_Enhanced.vi"("PhoenixMotorControlDevRef"=w1559, "error in"=w1560) -> ("PhoenixMotorControlDevRef"=w1557:T4, "error out"=w1556:errorcluster)  [unwired: 8 in, 4 out]
                        n471 = call-poly <vilib>:"CTRE_Phoenix_MotorController_Get_Enhanced.vi"("PhoenixMotorControlDevRef"=w1566, "error in"=w1567) -> ("PhoenixMotorControlDevRef"=w1562:T4, "error out"=w1561:errorcluster)  [unwired: 8 in, 4 out]
                      }
                    }
                    frame #3 {
                      n472 = while {
                        tunnel: w1577 -> [w1600]
                        tunnel: w1576 -> [w1599]
                        tunnel: [w1596] -> w1575
                        tunnel: [w1595] -> w1574
                        tunnel: [w1591] -> w1573
                        tunnel: [w1590] -> w1572
                        tunnel: w1571 -> [w1589]
                        tunnel: w1570 -> [w1588]
                        tunnel: w1569 -> [w1581]
                        stop <- w1597 stop-if-true
                        w1592 = T14 7 items=["PercentOutput"=0, "Position"=1, "Velocity"=2, "Current"=3, "Follower"=5, "MotionProfile"=6, "MotionMagic"=7, "MotionMagicArc"=8, "MotionProfileArc"=10, "Disabled"=15] ("Control Mode")
                        w1601 = T14 7 items=["PercentOutput"=0, "Position"=1, "Velocity"=2, "Current"=3, "Follower"=5, "MotionProfile"=6, "MotionMagic"=7, "MotionMagicArc"=8, "MotionProfileArc"=10, "Disabled"=15] ("Control Mode")
                        n473 = global read "Robot Global Data.vi" "Robot Yaw"() -> (w1584:dbl)
                        n474 = global read "Robot Global Data.vi" "Robot Travel"() -> (w1598:dbl)
                        n475 = Wait (ms)(milliseconds to wait=u32 50) -> ()  [unwired: 1 out]
                        n476 = Greater?(x=w1598, y=383.75) -> (0:w1597:bool)
                        n477 = call-poly <vilib>:"PID.vi"("process variable"=w1584, "setpoint"=-90.0) -> ("output"=w1578:dbl)  [unwired: 8 in, 1 out]
                        n478 = Multiply(x=w1578, y=-1.0) -> (x*y=w1579:dbl)
                        n479 = Multiply(x=384.75 ("Output"), y=217.294) -> (x*y=w1585:dbl)
                        n480 = call <vilib>:"CTRE_Phoenix_MotorControl_Set.vi"("Demand1"=w1578, "DemandType"=w1581, "error in (no error)"=w1588, "Output"=w1585, "Control Mode"=w1592, "PhoenixMotorControlDevRef"=w1589) -> ("error out"=w1594:errorcluster, "PhoenixMotorControlDevRef"=w1593:T4)  [unwired: 4 in]
                        n481 = call <vilib>:"CTRE_Phoenix_MotorControl_Set.vi"("Demand1"=w1579, "DemandType"=w1581, "error in (no error)"=w1599, "Output"=w1585, "Control Mode"=w1601, "PhoenixMotorControlDevRef"=w1600) -> ("error out"=w1603:errorcluster, "PhoenixMotorControlDevRef"=w1602:T4)  [unwired: 4 in]
                        n482 = call-poly <vilib>:"CTRE_Phoenix_MotorController_Get_Enhanced.vi"("PhoenixMotorControlDevRef"=w1593, "error in"=w1594) -> ("PhoenixMotorControlDevRef"=w1591:T4, "error out"=w1590:errorcluster)  [unwired: 8 in, 4 out]
                        n483 = call-poly <vilib>:"CTRE_Phoenix_MotorController_Get_Enhanced.vi"("PhoenixMotorControlDevRef"=w1602, "error in"=w1603) -> ("PhoenixMotorControlDevRef"=w1596:T4, "error out"=w1595:errorcluster)  [unwired: 8 in, 4 out]
                      }
                    }
                    frame #4 {
                      n484 = while {
                        tunnel: w1613 -> [w1636]
                        tunnel: w1612 -> [w1635]
                        tunnel: [w1634] -> w1611
                        tunnel: [w1633] -> w1610
                        tunnel: [w1629] -> w1609
                        tunnel: [w1628] -> w1608
                        tunnel: w1607 -> [w1627]
                        tunnel: w1606 -> [w1626]
                        tunnel: w1605 -> [w1616]
                        stop <- w1623 stop-if-true
                        w1630 = T14 7 items=["PercentOutput"=0, "Position"=1, "Velocity"=2, "Current"=3, "Follower"=5, "MotionProfile"=6, "MotionMagic"=7, "MotionMagicArc"=8, "MotionProfileArc"=10, "Disabled"=15] ("Control Mode")
                        w1637 = T14 7 items=["PercentOutput"=0, "Position"=1, "Velocity"=2, "Current"=3, "Follower"=5, "MotionProfile"=6, "MotionMagic"=7, "MotionMagicArc"=8, "MotionProfileArc"=10, "Disabled"=15] ("Control Mode")
                        n485 = global read "Robot Global Data.vi" "Robot Yaw"() -> (w1619:dbl)
                        n486 = global read "Robot Global Data.vi" "Robot Yaw"() -> (w1624:dbl)
                        n487 = Wait (ms)(milliseconds to wait=u32 50) -> ()  [unwired: 1 out]
                        n488 = call-poly <vilib>:"PID.vi"("process variable"=w1619, "setpoint"=-180.0) -> ("output"=w1614:dbl)  [unwired: 8 in, 1 out]
                        n489 = Multiply(x=w1614, y=-1.0) -> (x*y=w1615:dbl)
                        n490 = Less?(x=w1624, y=-180) -> (x < y?=w1623:bool)
                        n491 = Multiply(x=384.75 ("Output"), y=217.294) -> (x*y=w1620:dbl)
                        n492 = call <vilib>:"CTRE_Phoenix_MotorControl_Set.vi"("Demand1"=w1614, "DemandType"=w1616, "error in (no error)"=w1626, "Output"=w1620, "Control Mode"=w1630, "PhoenixMotorControlDevRef"=w1627) -> ("error out"=w1632:errorcluster, "PhoenixMotorControlDevRef"=w1631:T4)  [unwired: 4 in]
                        n493 = call <vilib>:"CTRE_Phoenix_MotorControl_Set.vi"("Demand1"=w1615, "DemandType"=w1616, "error in (no error)"=w1635, "Output"=w1620, "Control Mode"=w1637, "PhoenixMotorControlDevRef"=w1636) -> ("error out"=w1639:errorcluster, "PhoenixMotorControlDevRef"=w1638:T4)  [unwired: 4 in]
                        n494 = call-poly <vilib>:"CTRE_Phoenix_MotorController_Get_Enhanced.vi"("PhoenixMotorControlDevRef"=w1631, "error in"=w1632) -> ("PhoenixMotorControlDevRef"=w1629:T4, "error out"=w1628:errorcluster)  [unwired: 8 in, 4 out]
                        n495 = call-poly <vilib>:"CTRE_Phoenix_MotorController_Get_Enhanced.vi"("PhoenixMotorControlDevRef"=w1638, "error in"=w1639) -> ("PhoenixMotorControlDevRef"=w1634:T4, "error out"=w1633:errorcluster)  [unwired: 8 in, 4 out]
                      }
                    }
                    frame #5 {
                      n496 = while {
                        tunnel: w1649 -> [w1674]
                        tunnel: w1648 -> [w1673]
                        tunnel: [w1670] -> w1647
                        tunnel: [w1669] -> w1646
                        tunnel: w1645 -> [w1665]
                        tunnel: w1644 -> [w1664]
                        tunnel: [w1663] -> w1643
                        tunnel: [w1662] -> w1642
                        tunnel: w1641 -> [w1655]
                        stop <- w1671 stop-if-true
                        w1666 = T14 7 items=["PercentOutput"=0, "Position"=1, "Velocity"=2, "Current"=3, "Follower"=5, "MotionProfile"=6, "MotionMagic"=7, "MotionMagicArc"=8, "MotionProfileArc"=10, "Disabled"=15] ("Control Mode")
                        w1675 = T14 7 items=["PercentOutput"=0, "Position"=1, "Velocity"=2, "Current"=3, "Follower"=5, "MotionProfile"=6, "MotionMagic"=7, "MotionMagicArc"=8, "MotionProfileArc"=10, "Disabled"=15] ("Control Mode")
                        n497 = global read "Robot Global Data.vi" "Robot Yaw"() -> (w1658:dbl)
                        n498 = global read "Robot Global Data.vi" "Robot Travel"() -> (w1672:dbl)
                        n499 = Wait (ms)(milliseconds to wait=u32 50) -> ()  [unwired: 1 out]
                        n500 = Greater?(x=w1672, y=390.5) -> (0:w1671:bool)
                        n501 = call-poly <vilib>:"PID.vi"("process variable"=w1658, "setpoint"=-180.0) -> ("output"=w1652:dbl)  [unwired: 8 in, 1 out]
                        n502 = Multiply(x=w1652, y=-1.0) -> (x*y=w1653:dbl)
                        n503 = global write "Robot Global Data.vi" "Elevator Bottom"(FALSE) -> ()
                        n504 = global write "Robot Global Data.vi" "Elevator Mid"(TRUE) -> ()
                        n505 = Multiply(x=391.5 ("Output"), y=217.294) -> (x*y=w1659:dbl)
                        n506 = call <vilib>:"CTRE_Phoenix_MotorControl_Set.vi"("Demand1"=w1652, "DemandType"=w1655, "error in (no error)"=w1664, "Output"=w1659, "Control Mode"=w1666, "PhoenixMotorControlDevRef"=w1665) -> ("error out"=w1668:errorcluster, "PhoenixMotorControlDevRef"=w1667:T4)  [unwired: 4 in]
                        n507 = call <vilib>:"CTRE_Phoenix_MotorControl_Set.vi"("Demand1"=w1653, "DemandType"=w1655, "error in (no error)"=w1673, "Output"=w1659, "Control Mode"=w1675, "PhoenixMotorControlDevRef"=w1674) -> ("error out"=w1677:errorcluster, "PhoenixMotorControlDevRef"=w1676:T4)  [unwired: 4 in]
                        n508 = call-poly <vilib>:"CTRE_Phoenix_MotorController_Get_Enhanced.vi"("PhoenixMotorControlDevRef"=w1667, "error in"=w1668) -> ("PhoenixMotorControlDevRef"=w1663:T4, "error out"=w1662:errorcluster)  [unwired: 8 in, 4 out]
                        n509 = call-poly <vilib>:"CTRE_Phoenix_MotorController_Get_Enhanced.vi"("PhoenixMotorControlDevRef"=w1676, "error in"=w1677) -> ("PhoenixMotorControlDevRef"=w1670:T4, "error out"=w1669:errorcluster)  [unwired: 8 in, 4 out]
                      }
                    }
                    frame #6 {
                      n510 = while {
                        tunnel: w1687 -> [w1712]
                        tunnel: w1686 -> [w1711]
                        tunnel: [w1710] -> w1685
                        tunnel: [w1709] -> w1684
                        tunnel: w1683 -> [w1705]
                        tunnel: w1682 -> [w1704]
                        tunnel: [w1703] -> w1681
                        tunnel: [w1702] -> w1680
                        tunnel: w1679 -> [w1691]
                        i -> [w1699]
                        stop <- w1698 stop-if-true
                        w1706 = T14 7 items=["PercentOutput"=0, "Position"=1, "Velocity"=2, "Current"=3, "Follower"=5, "MotionProfile"=6, "MotionMagic"=7, "MotionMagicArc"=8, "MotionProfileArc"=10, "Disabled"=15] ("Control Mode")
                        w1713 = T14 7 items=["PercentOutput"=0, "Position"=1, "Velocity"=2, "Current"=3, "Follower"=5, "MotionProfile"=6, "MotionMagic"=7, "MotionMagicArc"=8, "MotionProfileArc"=10, "Disabled"=15] ("Control Mode")
                        # "ADD INTAKE/ELEVATOR CODE HERE"
                        n511 = global read "Robot Global Data.vi" "Robot Yaw"() -> (w1694:dbl)
                        n512 = Increment(x=w1699) -> (x+1=w1700:i32)
                        n513 = Wait (ms)(milliseconds to wait=u32 50) -> ()  [unwired: 1 out]
                        n514 = Greater Or Equal?(x=w1700, y=20) -> (x >= y?=w1698:bool)
                        n515 = call-poly <vilib>:"PID.vi"("process variable"=w1694, "setpoint"=-180.0) -> ("output"=w1689:dbl)  [unwired: 8 in, 1 out]
                        n516 = Multiply(x=w1689, y=-1.0) -> (x*y=w1690:dbl)
                        n517 = global write "Robot Global Data.vi" "Intake Out Full"(TRUE) -> ()
                        n518 = Multiply(x=391.5 ("Output"), y=217.294) -> (x*y=w1695:dbl)
                        n519 = call <vilib>:"CTRE_Phoenix_MotorControl_Set.vi"("Demand1"=w1689, "DemandType"=w1691, "error in (no error)"=w1704, "Output"=w1695, "Control Mode"=w1706, "PhoenixMotorControlDevRef"=w1705) -> ("error out"=w1708:errorcluster, "PhoenixMotorControlDevRef"=w1707:T4)  [unwired: 4 in]
                        n520 = call <vilib>:"CTRE_Phoenix_MotorControl_Set.vi"("Demand1"=w1690, "DemandType"=w1691, "error in (no error)"=w1711, "Output"=w1695, "Control Mode"=w1713, "PhoenixMotorControlDevRef"=w1712) -> ("error out"=w1715:errorcluster, "PhoenixMotorControlDevRef"=w1714:T4)  [unwired: 4 in]
                        n521 = call-poly <vilib>:"CTRE_Phoenix_MotorController_Get_Enhanced.vi"("PhoenixMotorControlDevRef"=w1707, "error in"=w1708) -> ("PhoenixMotorControlDevRef"=w1703:T4, "error out"=w1702:errorcluster)  [unwired: 8 in, 4 out]
                        n522 = call-poly <vilib>:"CTRE_Phoenix_MotorController_Get_Enhanced.vi"("PhoenixMotorControlDevRef"=w1714, "error in"=w1715) -> ("PhoenixMotorControlDevRef"=w1710:T4, "error out"=w1709:errorcluster)  [unwired: 8 in, 4 out]
                      }
                    }
                    frame #7 {
                      n523 = while {
                        tunnel: w1720 -> [w1735]
                        tunnel: w1719 -> [w1734]
                        tunnel: w1718 -> [w1732]
                        tunnel: w1717 -> [w1731]
                        i -> [w1727]
                        stop <- w1728 stop-if-true
                        w1733 = T14 0 items=["PercentOutput"=0, "Position"=1, "Velocity"=2, "Current"=3, "Follower"=5, "MotionProfile"=6, "MotionMagic"=7, "MotionMagicArc"=8, "MotionProfileArc"=10, "Disabled"=15] ("Control Mode")
                        w1736 = T14 0 items=["PercentOutput"=0, "Position"=1, "Velocity"=2, "Current"=3, "Follower"=5, "MotionProfile"=6, "MotionMagic"=7, "MotionMagicArc"=8, "MotionProfileArc"=10, "Disabled"=15] ("Control Mode")
                        n524 = Increment(x=w1727) -> (x+1=w1729:i32)
                        n525 = Wait (ms)(milliseconds to wait=u32 15000) -> ()  [unwired: 1 out]
                        n526 = global write "Robot Global Data.vi" "Intake Out Full"(FALSE) -> ()
                        n527 = global write "Robot Global Data.vi" "Elevator Mid"(FALSE) -> ()
                        n528 = Greater Or Equal?(x=w1729, y=1) -> (x >= y?=w1728:bool)
                        n529 = call <vilib>:"CTRE_Phoenix_MotorControl_Set.vi"("DemandType"=T2."DemandType_Neutral", "error in (no error)"=w1731, "Output"=0.0, "Control Mode"=w1733, "PhoenixMotorControlDevRef"=w1732) -> ()  [unwired: 5 in, 2 out]
                        n530 = call <vilib>:"CTRE_Phoenix_MotorControl_Set.vi"("DemandType"=T2."DemandType_Neutral", "error in (no error)"=w1734, "Output"=0.0, "Control Mode"=w1736, "PhoenixMotorControlDevRef"=w1735) -> ()  [unwired: 5 in, 2 out]
                      }
                    }
                  }
                }
              }
            }
            frame 4 {
              n531 = case shown="\"R\"" w1757 {
                tunnel: w1756 -> [w1788 _ w2136]
                tunnel: w1755 -> [w1787 _ w2135]
                tunnel: w1754 -> [w1786 _ w2134]
                tunnel: w1753 -> [w1785 _ w2133]
                tunnel: w1752 -> [w1776 _ w2132]
                tunnel: w1751 -> [w1775 _ _]
                tunnel: w1750 -> [w1774 _ _]
                tunnel: w1749 -> [w1773 _ _]
                tunnel: w1748 -> [w1772 _ _]
                tunnel: w1747 -> [w1771 _ _]
                tunnel: w1746 -> [w1770 _ _]
                tunnel: w1745 -> [w1769 _ _]
                tunnel: w1744 -> [w1768 _ _]
                tunnel: w1743 -> [w1767 _ _]
                tunnel: w1742 -> [w1766 _ _]
                tunnel: w1741 -> [w1765 _ _]
                tunnel: w1740 -> [w1764 _ _]
                tunnel: w1739 -> [w1763 _ _]
                tunnel: w1738 -> [w1762 _ _]
                frame "R" {
                  n532 = flat-sequence {
                    tunnel: w1785 -> [w1809]
                    tunnel: w1786 -> [w1810]
                    tunnel: w1787 -> [w1811]
                    tunnel: w1788 -> [w1812]
                    tunnel: [w1812] -> w1761
                    tunnel: [w1811] -> w1760
                    tunnel: [w1810] -> w1759
                    tunnel: [w1809] -> w1758
                    tunnel: [w1828] -> w1808
                    tunnel: [w1827] -> w1807
                    tunnel: [w1824] -> w1806
                    tunnel: [w1823] -> w1805
                    tunnel: w1776 -> [w1822]
                    tunnel: w1775 -> [w1821]
                    tunnel: w1774 -> [w1820]
                    tunnel: w1761 -> [w1830]
                    tunnel: w1760 -> [w1829]
                    tunnel: w1759 -> [w1826]
                    tunnel: w1758 -> [w1825]
                    tunnel: w1808 -> [w1873]
                    tunnel: w1807 -> [w1872]
                    tunnel: [w1871] -> w1804
                    tunnel: [w1870] -> w1803
                    tunnel: [w1869] -> w1802
                    tunnel: [w1868] -> w1801
                    tunnel: w1806 -> [w1867]
                    tunnel: w1805 -> [w1866]
                    tunnel: w1776 -> [w1865]
                    tunnel: w1773 -> [w1864]
                    tunnel: w1772 -> [w1863]
                    tunnel: w1804 -> [w1913]
                    tunnel: w1803 -> [w1912]
                    tunnel: [w1911] -> w1800
                    tunnel: [w1910] -> w1799
                    tunnel: [w1909] -> w1798
                    tunnel: [w1908] -> w1797
                    tunnel: w1802 -> [w1907]
                    tunnel: w1801 -> [w1906]
                    tunnel: w1776 -> [w1905]
                    tunnel: w1771 -> [w1904]
                    tunnel: w1770 -> [w1903]
                    tunnel: w1800 -> [w1953]
                    tunnel: w1799 -> [w1952]
                    tunnel: [w1951] -> w1796
                    tunnel: [w1950] -> w1795
                    tunnel: [w1949] -> w1794
                    tunnel: [w1948] -> w1793
                    tunnel: w1798 -> [w1947]
                    tunnel: w1797 -> [w1946]
                    tunnel: w1776 -> [w1945]
                    tunnel: w1769 -> [w1944]
                    tunnel: w1768 -> [w1943]
                    tunnel: w1796 -> [w1993]
                    tunnel: w1795 -> [w1992]
                    tunnel: [w1991] -> w1784
                    tunnel: [w1990] -> w1783
                    tunnel: w1794 -> [w1989]
                    tunnel: w1793 -> [w1988]
                    tunnel: [w1987] -> w1782
                    tunnel: [w1986] -> w1781
                    tunnel: w1776 -> [w1985]
                    tunnel: w1767 -> [w1984]
                    tunnel: w1766 -> [w1983]
                    tunnel: w1784 -> [w2035]
                    tunnel: w1783 -> [w2034]
                    tunnel: w1782 -> [w2033]
                    tunnel: w1781 -> [w2032]
                    tunnel: [w2031] -> w1780
                    tunnel: [w2030] -> w1779
                    tunnel: [w2029] -> w1778
                    tunnel: [w2028] -> w1777
                    tunnel: w1776 -> [w2027]
                    tunnel: w1765 -> [w2026]
                    tunnel: w1764 -> [w2025]
                    tunnel: [w2075] -> w1792
                    tunnel: [w2074] -> w1791
                    tunnel: [w2073] -> w1790
                    tunnel: [w2072] -> w1789
                    tunnel: w1780 -> [w2071]
                    tunnel: w1779 -> [w2070]
                    tunnel: w1778 -> [w2069]
                    tunnel: w1777 -> [w2068]
                    tunnel: w1776 -> [w2067]
                    tunnel: w1763 -> [w2066]
                    tunnel: w1762 -> [w2065]
                    tunnel: w1792 -> [w2110]
                    tunnel: w1791 -> [w2109]
                    tunnel: w1790 -> [w2108]
                    tunnel: w1789 -> [w2107]
                    frame #0 {
                      n533 = while {
                        i -> [w1814]
                        stop <- w1815 stop-if-true
                        n534 = Increment(x=w1814) -> (x+1=w1816:i32)
                        n535 = global write "Robot Global Data.vi" "Zero Travel"(TRUE) -> ()
                        n536 = global write "Robot Global Data.vi" "Zero Yaw"(TRUE) -> ()
                        n537 = Wait (ms)(milliseconds to wait=u32 10) -> ()  [unwired: 1 out]
                        n538 = Greater Or Equal?(x=w1816, y=1) -> (x >= y?=w1815:bool)
                      }
                    }
                    frame #1 {
                      n539 = while {
                        tunnel: w1830 -> [w1857]
                        tunnel: w1829 -> [w1856]
                        tunnel: [w1855] -> w1828
                        tunnel: [w1854] -> w1827
                        tunnel: w1826 -> [w1848]
                        tunnel: w1825 -> [w1847]
                        tunnel: [w1846] -> w1824
                        tunnel: [w1845] -> w1823
                        tunnel: w1822 -> [w1837]
                        tunnel: w1821 -> [w1834]
                        tunnel: w1820 -> [w1833]
                        stop <- w1852 stop-if-true
                        w1849 = T14 7 items=["PercentOutput"=0, "Position"=1, "Velocity"=2, "Current"=3, "Follower"=5, "MotionProfile"=6, "MotionMagic"=7, "MotionMagicArc"=8, "MotionProfileArc"=10, "Disabled"=15] ("Control Mode")
                        w1858 = T14 7 items=["PercentOutput"=0, "Position"=1, "Velocity"=2, "Current"=3, "Follower"=5, "MotionProfile"=6, "MotionMagic"=7, "MotionMagicArc"=8, "MotionProfileArc"=10, "Disabled"=15] ("Control Mode")
                        n540 = global write "Robot Global Data.vi" "Elevator Bottom"(TRUE) -> ()
                        n541 = global read "Robot Global Data.vi" "Robot Yaw"() -> (w1840:dbl)
                        n542 = Wait (ms)(milliseconds to wait=u32 50) -> ()  [unwired: 1 out]
                        n543 = global read "Robot Global Data.vi" "Robot Travel"() -> (w1853:dbl)
                        n544 = global write "Robot Global Data.vi" "Zero Travel"(FALSE) -> ()
                        n545 = global write "Robot Global Data.vi" "Zero Yaw"(FALSE) -> ()
                        n546 = Greater?(x=w1853, y=214.75) -> (0:w1852:bool)
                        n547 = Multiply(x=215.75 ("Output"), y=217.294) -> (x*y=w1842:dbl)
                        n548 = call-poly <vilib>:"PID.vi"("output range"=w1834, "PID gains"=w1833, "process variable"=w1840, "setpoint"=0.0) -> ("output"=w1835:dbl)  [unwired: 6 in, 1 out]
                        n549 = call <vilib>:"CTRE_Phoenix_MotorControl_Set.vi"("Demand1"=w1835, "DemandType"=w1837, "error in (no error)"=w1847, "Output"=w1842, "Control Mode"=w1849, "PhoenixMotorControlDevRef"=w1848) -> ("error out"=w1851:errorcluster, "PhoenixMotorControlDevRef"=w1850:T4)  [unwired: 4 in]
                        n550 = call-poly <vilib>:"CTRE_Phoenix_MotorController_Get_Enhanced.vi"("PhoenixMotorControlDevRef"=w1850, "error in"=w1851) -> ("PhoenixMotorControlDevRef"=w1846:T4, "error out"=w1845:errorcluster)  [unwired: 8 in, 4 out]
                        n551 = Multiply(x=w1835, y=-1.0) -> (x*y=w1836:dbl)
                        n552 = call <vilib>:"CTRE_Phoenix_MotorControl_Set.vi"("Demand1"=w1836, "DemandType"=w1837, "error in (no error)"=w1856, "Output"=w1842, "Control Mode"=w1858, "PhoenixMotorControlDevRef"=w1857) -> ("error out"=w1860:errorcluster, "PhoenixMotorControlDevRef"=w1859:T4)  [unwired: 4 in]
                        n553 = call-poly <vilib>:"CTRE_Phoenix_MotorController_Get_Enhanced.vi"("PhoenixMotorControlDevRef"=w1859, "error in"=w1860) -> ("PhoenixMotorControlDevRef"=w1855:T4, "error out"=w1854:errorcluster)  [unwired: 8 in, 4 out]
                      }
                    }
                    frame #2 {
                      n554 = while {
                        tunnel: w1873 -> [w1898]
                        tunnel: w1872 -> [w1897]
                        tunnel: [w1896] -> w1871
                        tunnel: [w1895] -> w1870
                        tunnel: [w1891] -> w1869
                        tunnel: [w1890] -> w1868
                        tunnel: w1867 -> [w1889]
                        tunnel: w1866 -> [w1888]
                        tunnel: w1865 -> [w1878]
                        tunnel: w1864 -> [w1875]
                        tunnel: w1863 -> [w1874]
                        stop <- w1887 stop-if-true
                        w1892 = T14 7 items=["PercentOutput"=0, "Position"=1, "Velocity"=2, "Current"=3, "Follower"=5, "MotionProfile"=6, "MotionMagic"=7, "MotionMagicArc"=8, "MotionProfileArc"=10, "Disabled"=15] ("Control Mode")
                        w1899 = T14 7 items=["PercentOutput"=0, "Position"=1, "Velocity"=2, "Current"=3, "Follower"=5, "MotionProfile"=6, "MotionMagic"=7, "MotionMagicArc"=8, "MotionProfileArc"=10, "Disabled"=15] ("Control Mode")
                        n555 = Wait (ms)(milliseconds to wait=u32 50) -> ()  [unwired: 1 out]
                        n556 = global read "Robot Global Data.vi" "Robot Yaw"() -> (w1881:dbl)
                        n557 = global read "Robot Global Data.vi" "Robot Yaw"() -> (w1885:dbl)
                        n558 = Greater?(x=w1885, y=90) -> (0:w1887:bool)
                        n559 = call-poly <vilib>:"PID.vi"("output range"=w1875, "PID gains"=w1874, "process variable"=w1881, "setpoint"=90.0) -> ("output"=w1876:dbl)  [unwired: 6 in, 1 out]
                        n560 = Multiply(x=w1876, y=-1.0) -> (x*y=w1877:dbl)
                        n561 = Multiply(x=215.75 ("Output"), y=217.294) -> (x*y=w1882:dbl)
                        n562 = call <vilib>:"CTRE_Phoenix_MotorControl_Set.vi"("Demand1"=w1876, "DemandType"=w1878, "error in (no error)"=w1888, "Output"=w1882, "Control Mode"=w1892, "PhoenixMotorControlDevRef"=w1889) -> ("error out"=w1894:errorcluster, "PhoenixMotorControlDevRef"=w1893:T4)  [unwired: 4 in]
                        n563 = call <vilib>:"CTRE_Phoenix_MotorControl_Set.vi"("Demand1"=w1877, "DemandType"=w1878, "error in (no error)"=w1897, "Output"=w1882, "Control Mode"=w1899, "PhoenixMotorControlDevRef"=w1898) -> ("error out"=w1901:errorcluster, "PhoenixMotorControlDevRef"=w1900:T4)  [unwired: 4 in]
                        n564 = call-poly <vilib>:"CTRE_Phoenix_MotorController_Get_Enhanced.vi"("PhoenixMotorControlDevRef"=w1893, "error in"=w1894) -> ("PhoenixMotorControlDevRef"=w1891:T4, "error out"=w1890:errorcluster)  [unwired: 8 in, 4 out]
                        n565 = call-poly <vilib>:"CTRE_Phoenix_MotorController_Get_Enhanced.vi"("PhoenixMotorControlDevRef"=w1900, "error in"=w1901) -> ("PhoenixMotorControlDevRef"=w1896:T4, "error out"=w1895:errorcluster)  [unwired: 8 in, 4 out]
                      }
                    }
                    frame #3 {
                      n566 = while {
                        tunnel: w1913 -> [w1938]
                        tunnel: w1912 -> [w1937]
                        tunnel: [w1934] -> w1911
                        tunnel: [w1933] -> w1910
                        tunnel: [w1929] -> w1909
                        tunnel: [w1928] -> w1908
                        tunnel: w1907 -> [w1927]
                        tunnel: w1906 -> [w1926]
                        tunnel: w1905 -> [w1918]
                        tunnel: w1904 -> [w1915]
                        tunnel: w1903 -> [w1914]
                        stop <- w1935 stop-if-true
                        w1930 = T14 7 items=["PercentOutput"=0, "Position"=1, "Velocity"=2, "Current"=3, "Follower"=5, "MotionProfile"=6, "MotionMagic"=7, "MotionMagicArc"=8, "MotionProfileArc"=10, "Disabled"=15] ("Control Mode")
                        w1939 = T14 7 items=["PercentOutput"=0, "Position"=1, "Velocity"=2, "Current"=3, "Follower"=5, "MotionProfile"=6, "MotionMagic"=7, "MotionMagicArc"=8, "MotionProfileArc"=10, "Disabled"=15] ("Control Mode")
                        n567 = global read "Robot Global Data.vi" "Robot Travel"() -> (w1936:dbl)
                        n568 = global read "Robot Global Data.vi" "Robot Yaw"() -> (w1921:dbl)
                        n569 = Wait (ms)(milliseconds to wait=u32 50) -> ()  [unwired: 1 out]
                        n570 = Greater?(x=w1936, y=439.75) -> (0:w1935:bool)
                        n571 = call-poly <vilib>:"PID.vi"("output range"=w1915, "PID gains"=w1914, "process variable"=w1921, "setpoint"=90.0) -> ("output"=w1916:dbl)  [unwired: 6 in, 1 out]
                        n572 = Multiply(x=w1916, y=-1.0) -> (x*y=w1917:dbl)
                        n573 = Multiply(x=440.75 ("Output"), y=217.294) -> (x*y=w1923:dbl)
                        n574 = call <vilib>:"CTRE_Phoenix_MotorControl_Set.vi"("Demand1"=w1916, "DemandType"=w1918, "error in (no error)"=w1926, "Output"=w1923, "Control Mode"=w1930, "PhoenixMotorControlDevRef"=w1927) -> ("error out"=w1932:errorcluster, "PhoenixMotorControlDevRef"=w1931:T4)  [unwired: 4 in]
                        n575 = call <vilib>:"CTRE_Phoenix_MotorControl_Set.vi"("Demand1"=w1917, "DemandType"=w1918, "error in (no error)"=w1937, "Output"=w1923, "Control Mode"=w1939, "PhoenixMotorControlDevRef"=w1938) -> ("error out"=w1941:errorcluster, "PhoenixMotorControlDevRef"=w1940:T4)  [unwired: 4 in]
                        n576 = call-poly <vilib>:"CTRE_Phoenix_MotorController_Get_Enhanced.vi"("PhoenixMotorControlDevRef"=w1931, "error in"=w1932) -> ("PhoenixMotorControlDevRef"=w1929:T4, "error out"=w1928:errorcluster)  [unwired: 8 in, 4 out]
                        n577 = call-poly <vilib>:"CTRE_Phoenix_MotorController_Get_Enhanced.vi"("PhoenixMotorControlDevRef"=w1940, "error in"=w1941) -> ("PhoenixMotorControlDevRef"=w1934:T4, "error out"=w1933:errorcluster)  [unwired: 8 in, 4 out]
                      }
                    }
                    frame #4 {
                      n578 = while {
                        tunnel: w1953 -> [w1978]
                        tunnel: w1952 -> [w1977]
                        tunnel: [w1976] -> w1951
                        tunnel: [w1975] -> w1950
                        tunnel: [w1971] -> w1949
                        tunnel: [w1970] -> w1948
                        tunnel: w1947 -> [w1969]
                        tunnel: w1946 -> [w1968]
                        tunnel: w1945 -> [w1958]
                        tunnel: w1944 -> [w1955]
                        tunnel: w1943 -> [w1954]
                        stop <- w1965 stop-if-true
                        w1972 = T14 7 items=["PercentOutput"=0, "Position"=1, "Velocity"=2, "Current"=3, "Follower"=5, "MotionProfile"=6, "MotionMagic"=7, "MotionMagicArc"=8, "MotionProfileArc"=10, "Disabled"=15] ("Control Mode")
                        w1979 = T14 7 items=["PercentOutput"=0, "Position"=1, "Velocity"=2, "Current"=3, "Follower"=5, "MotionProfile"=6, "MotionMagic"=7, "MotionMagicArc"=8, "MotionProfileArc"=10, "Disabled"=15] ("Control Mode")
                        n579 = global read "Robot Global Data.vi" "Robot Yaw"() -> (w1966:dbl)
                        n580 = global read "Robot Global Data.vi" "Robot Yaw"() -> (w1961:dbl)
                        n581 = Wait (ms)(milliseconds to wait=u32 50) -> ()  [unwired: 1 out]
                        n582 = Less?(x=w1966, y=0) -> (x < y?=w1965:bool)
                        n583 = call-poly <vilib>:"PID.vi"("output range"=w1955, "PID gains"=w1954, "process variable"=w1961, "setpoint"=0.0) -> ("output"=w1956:dbl)  [unwired: 6 in, 1 out]
                        n584 = Multiply(x=w1956, y=-1.0) -> (x*y=w1957:dbl)
                        n585 = Multiply(x=440.75 ("Output"), y=217.294) -> (x*y=w1962:dbl)
                        n586 = call <vilib>:"CTRE_Phoenix_MotorControl_Set.vi"("Demand1"=w1956, "DemandType"=w1958, "error in (no error)"=w1968, "Output"=w1962, "Control Mode"=w1972, "PhoenixMotorControlDevRef"=w1969) -> ("error out"=w1974:errorcluster, "PhoenixMotorControlDevRef"=w1973:T4)  [unwired: 4 in]
                        n587 = call <vilib>:"CTRE_Phoenix_MotorControl_Set.vi"("Demand1"=w1957, "DemandType"=w1958, "error in (no error)"=w1977, "Output"=w1962, "Control Mode"=w1979, "PhoenixMotorControlDevRef"=w1978) -> ("error out"=w1981:errorcluster, "PhoenixMotorControlDevRef"=w1980:T4)  [unwired: 4 in]
                        n588 = call-poly <vilib>:"CTRE_Phoenix_MotorController_Get_Enhanced.vi"("PhoenixMotorControlDevRef"=w1973, "error in"=w1974) -> ("PhoenixMotorControlDevRef"=w1971:T4, "error out"=w1970:errorcluster)  [unwired: 8 in, 4 out]
                        n589 = call-poly <vilib>:"CTRE_Phoenix_MotorController_Get_Enhanced.vi"("PhoenixMotorControlDevRef"=w1980, "error in"=w1981) -> ("PhoenixMotorControlDevRef"=w1976:T4, "error out"=w1975:errorcluster)  [unwired: 8 in, 4 out]
                      }
                    }
                    frame #5 {
                      n590 = while {
                        tunnel: w1993 -> [w2020]
                        tunnel: w1992 -> [w2019]
                        tunnel: [w2016] -> w1991
                        tunnel: [w2015] -> w1990
                        tunnel: w1989 -> [w2011]
                        tunnel: w1988 -> [w2010]
                        tunnel: [w2009] -> w1987
                        tunnel: [w2008] -> w1986
                        tunnel: w1985 -> [w2000]
                        tunnel: w1984 -> [w1997]
                        tunnel: w1983 -> [w1996]
                        stop <- w2017 stop-if-true
                        w2012 = T14 7 items=["PercentOutput"=0, "Position"=1, "Velocity"=2, "Current"=3, "Follower"=5, "MotionProfile"=6, "MotionMagic"=7, "MotionMagicArc"=8, "MotionProfileArc"=10, "Disabled"=15] ("Control Mode")
                        w2021 = T14 7 items=["PercentOutput"=0, "Position"=1, "Velocity"=2, "Current"=3, "Follower"=5, "MotionProfile"=6, "MotionMagic"=7, "MotionMagicArc"=8, "MotionProfileArc"=10, "Disabled"=15] ("Control Mode")
                        n591 = global read "Robot Global Data.vi" "Robot Travel"() -> (w2018:dbl)
                        n592 = global read "Robot Global Data.vi" "Robot Yaw"() -> (w2003:dbl)
                        n593 = Wait (ms)(milliseconds to wait=u32 50) -> ()  [unwired: 1 out]
                        n594 = Greater?(x=w2018, y=528.5) -> (0:w2017:bool)
                        n595 = global write "Robot Global Data.vi" "Elevator Bottom"(FALSE) -> ()
                        n596 = global write "Robot Global Data.vi" "Elevator Top"(TRUE) -> ()
                        n597 = call-poly <vilib>:"PID.vi"("output range"=w1997, "PID gains"=w1996, "process variable"=w2003, "setpoint"=0.0) -> ("output"=w1998:dbl)  [unwired: 6 in, 1 out]
                        n598 = Multiply(x=w1998, y=-1.0) -> (x*y=w1999:dbl)
                        n599 = Multiply(x=529.5 ("Output"), y=217.294) -> (x*y=w2005:dbl)
                        n600 = call <vilib>:"CTRE_Phoenix_MotorControl_Set.vi"("Demand1"=w1998, "DemandType"=w2000, "error in (no error)"=w2010, "Output"=w2005, "Control Mode"=w2012, "PhoenixMotorControlDevRef"=w2011) -> ("error out"=w2014:errorcluster, "PhoenixMotorControlDevRef"=w2013:T4)  [unwired: 4 in]
                        n601 = call <vilib>:"CTRE_Phoenix_MotorControl_Set.vi"("Demand1"=w1999, "DemandType"=w2000, "error in (no error)"=w2019, "Output"=w2005, "Control Mode"=w2021, "PhoenixMotorControlDevRef"=w2020) -> ("error out"=w2023:errorcluster, "PhoenixMotorControlDevRef"=w2022:T4)  [unwired: 4 in]
                        n602 = call-poly <vilib>:"CTRE_Phoenix_MotorController_Get_Enhanced.vi"("PhoenixMotorControlDevRef"=w2013, "error in"=w2014) -> ("PhoenixMotorControlDevRef"=w2009:T4, "error out"=w2008:errorcluster)  [unwired: 8 in, 4 out]
                        n603 = call-poly <vilib>:"CTRE_Phoenix_MotorController_Get_Enhanced.vi"("PhoenixMotorControlDevRef"=w2022, "error in"=w2023) -> ("PhoenixMotorControlDevRef"=w2016:T4, "error out"=w2015:errorcluster)  [unwired: 8 in, 4 out]
                      }
                    }
                    frame #6 {
                      n604 = while {
                        tunnel: w2035 -> [w2060]
                        tunnel: w2034 -> [w2059]
                        tunnel: [w2058] -> w2031
                        tunnel: [w2057] -> w2030
                        tunnel: [w2053] -> w2029
                        tunnel: [w2052] -> w2028
                        tunnel: w2033 -> [w2051]
                        tunnel: w2032 -> [w2050]
                        tunnel: w2027 -> [w2040]
                        tunnel: w2026 -> [w2037]
                        tunnel: w2025 -> [w2036]
                        stop <- w2047 stop-if-true
                        w2054 = T14 7 items=["PercentOutput"=0, "Position"=1, "Velocity"=2, "Current"=3, "Follower"=5, "MotionProfile"=6, "MotionMagic"=7, "MotionMagicArc"=8, "MotionProfileArc"=10, "Disabled"=15] ("Control Mode")
                        w2061 = T14 7 items=["PercentOutput"=0, "Position"=1, "Velocity"=2, "Current"=3, "Follower"=5, "MotionProfile"=6, "MotionMagic"=7, "MotionMagicArc"=8, "MotionProfileArc"=10, "Disabled"=15] ("Control Mode")
                        n605 = global read "Robot Global Data.vi" "Robot Yaw"() -> (w2048:dbl)
                        n606 = global read "Robot Global Data.vi" "Robot Yaw"() -> (w2043:dbl)
                        n607 = Wait (ms)(milliseconds to wait=u32 50) -> ()  [unwired: 1 out]
                        n608 = Less?(x=w2048, y=-90) -> (x < y?=w2047:bool)
                        n609 = call-poly <vilib>:"PID.vi"("output range"=w2037, "PID gains"=w2036, "process variable"=w2043, "setpoint"=-90.0) -> ("output"=w2038:dbl)  [unwired: 6 in, 1 out]
                        n610 = Multiply(x=w2038, y=-1.0) -> (x*y=w2039:dbl)
                        n611 = Multiply(x=529.5 ("Output"), y=217.294) -> (x*y=w2044:dbl)
                        n612 = call <vilib>:"CTRE_Phoenix_MotorControl_Set.vi"("Demand1"=w2038, "DemandType"=w2040, "error in (no error)"=w2050, "Output"=w2044, "Control Mode"=w2054, "PhoenixMotorControlDevRef"=w2051) -> ("error out"=w2056:errorcluster, "PhoenixMotorControlDevRef"=w2055:T4)  [unwired: 4 in]
                        n613 = call <vilib>:"CTRE_Phoenix_MotorControl_Set.vi"("Demand1"=w2039, "DemandType"=w2040, "error in (no error)"=w2059, "Output"=w2044, "Control Mode"=w2061, "PhoenixMotorControlDevRef"=w2060) -> ("error out"=w2063:errorcluster, "PhoenixMotorControlDevRef"=w2062:T4)  [unwired: 4 in]
                        n614 = call-poly <vilib>:"CTRE_Phoenix_MotorController_Get_Enhanced.vi"("PhoenixMotorControlDevRef"=w2055, "error in"=w2056) -> ("PhoenixMotorControlDevRef"=w2053:T4, "error out"=w2052:errorcluster)  [unwired: 8 in, 4 out]
                        n615 = call-poly <vilib>:"CTRE_Phoenix_MotorController_Get_Enhanced.vi"("PhoenixMotorControlDevRef"=w2062, "error in"=w2063) -> ("PhoenixMotorControlDevRef"=w2058:T4, "error out"=w2057:errorcluster)  [unwired: 8 in, 4 out]
                      }
                    }
                    frame #7 {
                      n616 = while {
                        tunnel: [w2102] -> w2075
                        tunnel: [w2101] -> w2074
                        tunnel: [w2097] -> w2073
                        tunnel: [w2096] -> w2072
                        tunnel: w2071 -> [w2095]
                        tunnel: w2070 -> [w2094]
                        tunnel: w2069 -> [w2093]
                        tunnel: w2068 -> [w2092]
                        tunnel: w2067 -> [w2081]
                        tunnel: w2066 -> [w2078]
                        tunnel: w2065 -> [w2077]
                        i -> [w2088]
                        stop <- w2089 stop-if-true
                        w2098 = T14 7 items=["PercentOutput"=0, "Position"=1, "Velocity"=2, "Current"=3, "Follower"=5, "MotionProfile"=6, "MotionMagic"=7, "MotionMagicArc"=8, "MotionProfileArc"=10, "Disabled"=15] ("Control Mode")
                        w2103 = T14 7 items=["PercentOutput"=0, "Position"=1, "Velocity"=2, "Current"=3, "Follower"=5, "MotionProfile"=6, "MotionMagic"=7, "MotionMagicArc"=8, "MotionProfileArc"=10, "Disabled"=15] ("Control Mode")
                        # "ADD INTAKE/ELEVATOR CODE HERE"
                        n617 = Increment(x=w2088) -> (x+1=w2090:i32)
                        n618 = global read "Robot Global Data.vi" "Robot Yaw"() -> (w2084:dbl)
                        n619 = Wait (ms)(milliseconds to wait=u32 50) -> ()  [unwired: 1 out]
                        n620 = Greater Or Equal?(x=w2090, y=20) -> (x >= y?=w2089:bool)
                        n621 = global write "Robot Global Data.vi" "Intake Out Full"(TRUE) -> ()
                        n622 = call-poly <vilib>:"PID.vi"("output range"=w2078, "PID gains"=w2077, "process variable"=w2084, "setpoint"=-90.0) -> ("output"=w2079:dbl)  [unwired: 6 in, 1 out]
                        n623 = Multiply(x=w2079, y=-1.0) -> (x*y=w2080:dbl)
                        n624 = Multiply(x=529.5 ("Output"), y=217.294) -> (x*y=w2085:dbl)
                        n625 = call <vilib>:"CTRE_Phoenix_MotorControl_Set.vi"("Demand1"=w2079, "DemandType"=w2081, "error in (no error)"=w2092, "Output"=w2085, "Control Mode"=w2098, "PhoenixMotorControlDevRef"=w2093) -> ("error out"=w2100:errorcluster, "PhoenixMotorControlDevRef"=w2099:T4)  [unwired: 4 in]
                        n626 = call <vilib>:"CTRE_Phoenix_MotorControl_Set.vi"("Demand1"=w2080, "DemandType"=w2081, "error in (no error)"=w2094, "Output"=w2085, "Control Mode"=w2103, "PhoenixMotorControlDevRef"=w2095) -> ("error out"=w2105:errorcluster, "PhoenixMotorControlDevRef"=w2104:T4)  [unwired: 4 in]
                        n627 = call-poly <vilib>:"CTRE_Phoenix_MotorController_Get_Enhanced.vi"("PhoenixMotorControlDevRef"=w2099, "error in"=w2100) -> ("PhoenixMotorControlDevRef"=w2097:T4, "error out"=w2096:errorcluster)  [unwired: 8 in, 4 out]
                        n628 = call-poly <vilib>:"CTRE_Phoenix_MotorController_Get_Enhanced.vi"("PhoenixMotorControlDevRef"=w2104, "error in"=w2105) -> ("PhoenixMotorControlDevRef"=w2102:T4, "error out"=w2101:errorcluster)  [unwired: 8 in, 4 out]
                      }
                    }
                    frame #8 {
                      n629 = while {
                        tunnel: w2110 -> [w2125]
                        tunnel: w2109 -> [w2124]
                        tunnel: w2108 -> [w2122]
                        tunnel: w2107 -> [w2121]
                        i -> [w2115]
                        stop <- w2116 stop-if-true
                        w2123 = T14 0 items=["PercentOutput"=0, "Position"=1, "Velocity"=2, "Current"=3, "Follower"=5, "MotionProfile"=6, "MotionMagic"=7, "MotionMagicArc"=8, "MotionProfileArc"=10, "Disabled"=15] ("Control Mode")
                        w2126 = T14 0 items=["PercentOutput"=0, "Position"=1, "Velocity"=2, "Current"=3, "Follower"=5, "MotionProfile"=6, "MotionMagic"=7, "MotionMagicArc"=8, "MotionProfileArc"=10, "Disabled"=15] ("Control Mode")
                        n630 = Increment(x=w2115) -> (x+1=w2117:i32)
                        n631 = Wait (ms)(milliseconds to wait=u32 15000) -> ()  [unwired: 1 out]
                        n632 = Greater Or Equal?(x=w2117, y=1) -> (x >= y?=w2116:bool)
                        n633 = global write "Robot Global Data.vi" "Intake Out Full"(FALSE) -> ()
                        n634 = global write "Robot Global Data.vi" "Elevator Top"(FALSE) -> ()
                        n635 = call <vilib>:"CTRE_Phoenix_MotorControl_Set.vi"("DemandType"=T2."DemandType_Neutral", "error in (no error)"=w2121, "Output"=0.0, "Control Mode"=w2123, "PhoenixMotorControlDevRef"=w2122) -> ()  [unwired: 5 in, 2 out]
                        n636 = call <vilib>:"CTRE_Phoenix_MotorControl_Set.vi"("DemandType"=T2."DemandType_Neutral", "error in (no error)"=w2124, "Output"=0.0, "Control Mode"=w2126, "PhoenixMotorControlDevRef"=w2125) -> ()  [unwired: 5 in, 2 out]
                      }
                    }
                  }
                }
                frame Default {
                }
                frame "L" {
                  n637 = flat-sequence {
                    tunnel: w2133 -> [w2153]
                    tunnel: w2134 -> [w2154]
                    tunnel: w2135 -> [w2155]
                    tunnel: w2136 -> [w2156]
                    tunnel: [w2156] -> w2131
                    tunnel: [w2155] -> w2130
                    tunnel: [w2154] -> w2129
                    tunnel: [w2153] -> w2128
                    tunnel: [w2170] -> w2152
                    tunnel: [w2169] -> w2151
                    tunnel: [w2166] -> w2150
                    tunnel: [w2165] -> w2149
                    tunnel: w2132 -> [w2164]
                    tunnel: w2131 -> [w2172]
                    tunnel: w2130 -> [w2171]
                    tunnel: w2129 -> [w2168]
                    tunnel: w2128 -> [w2167]
                    tunnel: w2152 -> [w2211]
                    tunnel: w2151 -> [w2210]
                    tunnel: [w2209] -> w2148
                    tunnel: [w2208] -> w2147
                    tunnel: [w2207] -> w2146
                    tunnel: [w2206] -> w2145
                    tunnel: w2150 -> [w2205]
                    tunnel: w2149 -> [w2204]
                    tunnel: w2132 -> [w2203]
                    tunnel: w2148 -> [w2247]
                    tunnel: w2147 -> [w2246]
                    tunnel: w2146 -> [w2245]
                    tunnel: w2145 -> [w2244]
                    tunnel: [w2243] -> w2144
                    tunnel: [w2242] -> w2143
                    tunnel: [w2241] -> w2142
                    tunnel: [w2240] -> w2141
                    tunnel: w2132 -> [w2239]
                    tunnel: [w2285] -> w2140
                    tunnel: [w2284] -> w2139
                    tunnel: [w2283] -> w2138
                    tunnel: [w2282] -> w2137
                    tunnel: w2144 -> [w2281]
                    tunnel: w2143 -> [w2280]
                    tunnel: w2142 -> [w2279]
                    tunnel: w2141 -> [w2278]
                    tunnel: w2132 -> [w2277]
                    tunnel: w2140 -> [w2318]
                    tunnel: w2139 -> [w2317]
                    tunnel: w2138 -> [w2316]
                    tunnel: w2137 -> [w2315]
                    frame #0 {
                      n638 = while {
                        i -> [w2158]
                        stop <- w2159 stop-if-true
                        n639 = Increment(x=w2158) -> (x+1=w2160:i32)
                        n640 = global write "Robot Global Data.vi" "Zero Travel"(TRUE) -> ()
                        n641 = global write "Robot Global Data.vi" "Zero Yaw"(TRUE) -> ()
                        n642 = Wait (ms)(milliseconds to wait=u32 10) -> ()  [unwired: 1 out]
                        n643 = Greater Or Equal?(x=w2160, y=1) -> (x >= y?=w2159:bool)
                      }
                    }
                    frame #1 {
                      n644 = while {
                        tunnel: w2172 -> [w2197]
                        tunnel: w2171 -> [w2196]
                        tunnel: [w2195] -> w2170
                        tunnel: [w2194] -> w2169
                        tunnel: w2168 -> [w2188]
                        tunnel: w2167 -> [w2187]
                        tunnel: [w2186] -> w2166
                        tunnel: [w2185] -> w2165
                        tunnel: w2164 -> [w2178]
                        stop <- w2192 stop-if-true
                        w2189 = T14 7 items=["PercentOutput"=0, "Position"=1, "Velocity"=2, "Current"=3, "Follower"=5, "MotionProfile"=6, "MotionMagic"=7, "MotionMagicArc"=8, "MotionProfileArc"=10, "Disabled"=15] ("Control Mode")
                        w2198 = T14 7 items=["PercentOutput"=0, "Position"=1, "Velocity"=2, "Current"=3, "Follower"=5, "MotionProfile"=6, "MotionMagic"=7, "MotionMagicArc"=8, "MotionProfileArc"=10, "Disabled"=15] ("Control Mode")
                        n645 = global write "Robot Global Data.vi" "Elevator Bottom"(TRUE) -> ()
                        n646 = Wait (ms)(milliseconds to wait=u32 50) -> ()  [unwired: 1 out]
                        n647 = global read "Robot Global Data.vi" "Robot Travel"() -> (w2193:dbl)
                        n648 = global read "Robot Global Data.vi" "Robot Yaw"() -> (w2181:dbl)
                        n649 = global write "Robot Global Data.vi" "Zero Travel"(FALSE) -> ()
                        n650 = global write "Robot Global Data.vi" "Zero Yaw"(FALSE) -> ()
                        n651 = Greater?(x=w2193, y=303.5) -> (0:w2192:bool)
                        n652 = Multiply(x=304.5 ("Output"), y=217.294) -> (x*y=w2182:dbl)
                        n653 = call-poly <vilib>:"PID.vi"("process variable"=w2181, "setpoint"=0.0) -> ("output"=w2176:dbl)  [unwired: 8 in, 1 out]
                        n654 = call <vilib>:"CTRE_Phoenix_MotorControl_Set.vi"("Demand1"=w2176, "DemandType"=w2178, "error in (no error)"=w2187, "Output"=w2182, "Control Mode"=w2189, "PhoenixMotorControlDevRef"=w2188) -> ("error out"=w2191:errorcluster, "PhoenixMotorControlDevRef"=w2190:T4)  [unwired: 4 in]
                        n655 = call-poly <vilib>:"CTRE_Phoenix_MotorController_Get_Enhanced.vi"("PhoenixMotorControlDevRef"=w2190, "error in"=w2191) -> ("PhoenixMotorControlDevRef"=w2186:T4, "error out"=w2185:errorcluster)  [unwired: 8 in, 4 out]
                        n656 = Multiply(x=w2176, y=-1.0) -> (x*y=w2175:dbl)
                        n657 = call <vilib>:"CTRE_Phoenix_MotorControl_Set.vi"("Demand1"=w2175, "DemandType"=w2178, "error in (no error)"=w2196, "Output"=w2182, "Control Mode"=w2198, "PhoenixMotorControlDevRef"=w2197) -> ("error out"=w2200:errorcluster, "PhoenixMotorControlDevRef"=w2199:T4)  [unwired: 4 in]
                        n658 = call-poly <vilib>:"CTRE_Phoenix_MotorController_Get_Enhanced.vi"("PhoenixMotorControlDevRef"=w2199, "error in"=w2200) -> ("PhoenixMotorControlDevRef"=w2195:T4, "error out"=w2194:errorcluster)  [unwired: 8 in, 4 out]
                      }
                    }
                    frame #2 {
                      n659 = while {
                        tunnel: w2211 -> [w2234]
                        tunnel: w2210 -> [w2233]
                        tunnel: [w2232] -> w2209
                        tunnel: [w2231] -> w2208
                        tunnel: [w2227] -> w2207
                        tunnel: [w2226] -> w2206
                        tunnel: w2205 -> [w2225]
                        tunnel: w2204 -> [w2224]
                        tunnel: w2203 -> [w2214]
                        stop <- w2223 stop-if-true
                        w2228 = T14 7 items=["PercentOutput"=0, "Position"=1, "Velocity"=2, "Current"=3, "Follower"=5, "MotionProfile"=6, "MotionMagic"=7, "MotionMagicArc"=8, "MotionProfileArc"=10, "Disabled"=15] ("Control Mode")
                        w2235 = T14 7 items=["PercentOutput"=0, "Position"=1, "Velocity"=2, "Current"=3, "Follower"=5, "MotionProfile"=6, "MotionMagic"=7, "MotionMagicArc"=8, "MotionProfileArc"=10, "Disabled"=15] ("Control Mode")
                        n660 = Wait (ms)(milliseconds to wait=u32 50) -> ()  [unwired: 1 out]
                        n661 = global read "Robot Global Data.vi" "Robot Yaw"() -> (w2221:dbl)
                        n662 = global read "Robot Global Data.vi" "Robot Yaw"() -> (w2217:dbl)
                        n663 = Greater?(x=w2221, y=90) -> (0:w2223:bool)
                        n664 = Multiply(x=304.5 ("Output"), y=217.294) -> (x*y=w2218:dbl)
                        n665 = call-poly <vilib>:"PID.vi"("process variable"=w2217, "setpoint"=90.0) -> ("output"=w2213:dbl)  [unwired: 8 in, 1 out]
                        n666 = call <vilib>:"CTRE_Phoenix_MotorControl_Set.vi"("Demand1"=w2213, "DemandType"=w2214, "error in (no error)"=w2224, "Output"=w2218, "Control Mode"=w2228, "PhoenixMotorControlDevRef"=w2225) -> ("error out"=w2230:errorcluster, "PhoenixMotorControlDevRef"=w2229:T4)  [unwired: 4 in]
                        n667 = call-poly <vilib>:"CTRE_Phoenix_MotorController_Get_Enhanced.vi"("PhoenixMotorControlDevRef"=w2229, "error in"=w2230) -> ("PhoenixMotorControlDevRef"=w2227:T4, "error out"=w2226:errorcluster)  [unwired: 8 in, 4 out]
                        n668 = Multiply(x=w2213, y=-1.0) -> (x*y=w2212:dbl)
                        n669 = call <vilib>:"CTRE_Phoenix_MotorControl_Set.vi"("Demand1"=w2212, "DemandType"=w2214, "error in (no error)"=w2233, "Output"=w2218, "Control Mode"=w2235, "PhoenixMotorControlDevRef"=w2234) -> ("error out"=w2237:errorcluster, "PhoenixMotorControlDevRef"=w2236:T4)  [unwired: 4 in]
                        n670 = call-poly <vilib>:"CTRE_Phoenix_MotorController_Get_Enhanced.vi"("PhoenixMotorControlDevRef"=w2236, "error in"=w2237) -> ("PhoenixMotorControlDevRef"=w2232:T4, "error out"=w2231:errorcluster)  [unwired: 8 in, 4 out]
                      }
                    }
                    frame #3 {
                      n671 = while {
                        tunnel: w2247 -> [w2272]
                        tunnel: w2246 -> [w2271]
                        tunnel: [w2268] -> w2243
                        tunnel: [w2267] -> w2241
                        tunnel: [w2263] -> w2242
                        tunnel: [w2262] -> w2240
                        tunnel: w2245 -> [w2261]
                        tunnel: w2244 -> [w2260]
                        tunnel: w2239 -> [w2253]
                        stop <- w2269 stop-if-true
                        w2264 = T14 7 items=["PercentOutput"=0, "Position"=1, "Velocity"=2, "Current"=3, "Follower"=5, "MotionProfile"=6, "MotionMagic"=7, "MotionMagicArc"=8, "MotionProfileArc"=10, "Disabled"=15] ("Control Mode")
                        w2273 = T14 7 items=["PercentOutput"=0, "Position"=1, "Velocity"=2, "Current"=3, "Follower"=5, "MotionProfile"=6, "MotionMagic"=7, "MotionMagicArc"=8, "MotionProfileArc"=10, "Disabled"=15] ("Control Mode")
                        n672 = global read "Robot Global Data.vi" "Robot Travel"() -> (w2270:dbl)
                        n673 = Wait (ms)(milliseconds to wait=u32 50) -> ()  [unwired: 1 out]
                        n674 = global read "Robot Global Data.vi" "Robot Yaw"() -> (w2256:dbl)
                        n675 = Greater?(x=w2270, y=308.5) -> (0:w2269:bool)
                        n676 = global write "Robot Global Data.vi" "Elevator Bottom"(FALSE) -> ()
                        n677 = global write "Robot Global Data.vi" "Elevator Top"(TRUE) -> ()
                        n678 = Multiply(x=309.5 ("Output"), y=217.294) -> (x*y=w2257:dbl)
                        n679 = call-poly <vilib>:"PID.vi"("process variable"=w2256, "setpoint"=90.0) -> ("output"=w2251:dbl)  [unwired: 8 in, 1 out]
                        n680 = call <vilib>:"CTRE_Phoenix_MotorControl_Set.vi"("Demand1"=w2251, "DemandType"=w2253, "error in (no error)"=w2260, "Output"=w2257, "Control Mode"=w2264, "PhoenixMotorControlDevRef"=w2261) -> ("error out"=w2266:errorcluster, "PhoenixMotorControlDevRef"=w2265:T4)  [unwired: 4 in]
                        n681 = call-poly <vilib>:"CTRE_Phoenix_MotorController_Get_Enhanced.vi"("PhoenixMotorControlDevRef"=w2265, "error in"=w2266) -> ("PhoenixMotorControlDevRef"=w2263:T4, "error out"=w2262:errorcluster)  [unwired: 8 in, 4 out]
                        n682 = Multiply(x=w2251, y=-1.0) -> (x*y=w2250:dbl)
                        n683 = call <vilib>:"CTRE_Phoenix_MotorControl_Set.vi"("Demand1"=w2250, "DemandType"=w2253, "error in (no error)"=w2271, "Output"=w2257, "Control Mode"=w2273, "PhoenixMotorControlDevRef"=w2272) -> ("error out"=w2275:errorcluster, "PhoenixMotorControlDevRef"=w2274:T4)  [unwired: 4 in]
                        n684 = call-poly <vilib>:"CTRE_Phoenix_MotorController_Get_Enhanced.vi"("PhoenixMotorControlDevRef"=w2274, "error in"=w2275) -> ("PhoenixMotorControlDevRef"=w2268:T4, "error out"=w2267:errorcluster)  [unwired: 8 in, 4 out]
                      }
                    }
                    frame #4 {
                      n685 = while {
                        tunnel: w2281 -> [w2310]
                        tunnel: w2279 -> [w2309]
                        tunnel: [w2308] -> w2285
                        tunnel: [w2307] -> w2284
                        tunnel: w2280 -> [w2303]
                        tunnel: w2278 -> [w2302]
                        tunnel: [w2301] -> w2283
                        tunnel: [w2300] -> w2282
                        tunnel: w2277 -> [w2289]
                        i -> [w2296]
                        stop <- w2297 stop-if-true
                        w2304 = T14 7 items=["PercentOutput"=0, "Position"=1, "Velocity"=2, "Current"=3, "Follower"=5, "MotionProfile"=6, "MotionMagic"=7, "MotionMagicArc"=8, "MotionProfileArc"=10, "Disabled"=15] ("Control Mode")
                        w2311 = T14 7 items=["PercentOutput"=0, "Position"=1, "Velocity"=2, "Current"=3, "Follower"=5, "MotionProfile"=6, "MotionMagic"=7, "MotionMagicArc"=8, "MotionProfileArc"=10, "Disabled"=15] ("Control Mode")
                        # "ADD INTAKE/ELEVATOR CODE HERE"
                        n686 = Increment(x=w2296) -> (x+1=w2298:i32)
                        n687 = Wait (ms)(milliseconds to wait=u32 50) -> ()  [unwired: 1 out]
                        n688 = global read "Robot Global Data.vi" "Robot Yaw"() -> (w2292:dbl)
                        n689 = Greater Or Equal?(x=w2298, y=20) -> (x >= y?=w2297:bool)
                        n690 = global write "Robot Global Data.vi" "Intake Out Full"(TRUE) -> ()
                        n691 = Multiply(x=309.5 ("Output"), y=217.294) -> (x*y=w2293:dbl)
                        n692 = call-poly <vilib>:"PID.vi"("process variable"=w2292, "setpoint"=90.0) -> ("output"=w2288:dbl)  [unwired: 8 in, 1 out]
                        n693 = call <vilib>:"CTRE_Phoenix_MotorControl_Set.vi"("Demand1"=w2288, "DemandType"=w2289, "error in (no error)"=w2302, "Output"=w2293, "Control Mode"=w2304, "PhoenixMotorControlDevRef"=w2303) -> ("error out"=w2306:errorcluster, "PhoenixMotorControlDevRef"=w2305:T4)  [unwired: 4 in]
                        n694 = call-poly <vilib>:"CTRE_Phoenix_MotorController_Get_Enhanced.vi"("PhoenixMotorControlDevRef"=w2305, "error in"=w2306) -> ("PhoenixMotorControlDevRef"=w2301:T4, "error out"=w2300:errorcluster)  [unwired: 8 in, 4 out]
                        n695 = Multiply(x=w2288, y=-1.0) -> (x*y=w2287:dbl)
                        n696 = call <vilib>:"CTRE_Phoenix_MotorControl_Set.vi"("Demand1"=w2287, "DemandType"=w2289, "error in (no error)"=w2309, "Output"=w2293, "Control Mode"=w2311, "PhoenixMotorControlDevRef"=w2310) -> ("error out"=w2313:errorcluster, "PhoenixMotorControlDevRef"=w2312:T4)  [unwired: 4 in]
                        n697 = call-poly <vilib>:"CTRE_Phoenix_MotorController_Get_Enhanced.vi"("PhoenixMotorControlDevRef"=w2312, "error in"=w2313) -> ("PhoenixMotorControlDevRef"=w2308:T4, "error out"=w2307:errorcluster)  [unwired: 8 in, 4 out]
                      }
                    }
                    frame #5 {
                      n698 = while {
                        tunnel: w2318 -> [w2333]
                        tunnel: w2317 -> [w2332]
                        tunnel: w2316 -> [w2330]
                        tunnel: w2315 -> [w2329]
                        i -> [w2323]
                        stop <- w2324 stop-if-true
                        w2331 = T14 0 items=["PercentOutput"=0, "Position"=1, "Velocity"=2, "Current"=3, "Follower"=5, "MotionProfile"=6, "MotionMagic"=7, "MotionMagicArc"=8, "MotionProfileArc"=10, "Disabled"=15] ("Control Mode")
                        w2334 = T14 0 items=["PercentOutput"=0, "Position"=1, "Velocity"=2, "Current"=3, "Follower"=5, "MotionProfile"=6, "MotionMagic"=7, "MotionMagicArc"=8, "MotionProfileArc"=10, "Disabled"=15] ("Control Mode")
                        n699 = Increment(x=w2323) -> (x+1=w2325:i32)
                        n700 = global write "Robot Global Data.vi" "Intake Out Full"(FALSE) -> ()
                        n701 = global write "Robot Global Data.vi" "Elevator Top"(FALSE) -> ()
                        n702 = Greater Or Equal?(x=w2325, y=1) -> (x >= y?=w2324:bool)
                        n703 = Wait (ms)(milliseconds to wait=u32 15000) -> ()  [unwired: 1 out]
                        n704 = call <vilib>:"CTRE_Phoenix_MotorControl_Set.vi"("DemandType"=T2."DemandType_Neutral", "error in (no error)"=w2329, "Output"=0.0, "Control Mode"=w2331, "PhoenixMotorControlDevRef"=w2330) -> ()  [unwired: 5 in, 2 out]
                        n705 = call <vilib>:"CTRE_Phoenix_MotorControl_Set.vi"("DemandType"=T2."DemandType_Neutral", "error in (no error)"=w2332, "Output"=0.0, "Control Mode"=w2334, "PhoenixMotorControlDevRef"=w2333) -> ()  [unwired: 5 in, 2 out]
                      }
                    }
                  }
                }
              }
            }
            frame 5 {
              n706 = case shown="\"R\"" w2355 {
                tunnel: w2354 -> [w2376 _ w2622]
                tunnel: w2353 -> [w2375 _ w2621]
                tunnel: w2352 -> [w2374 _ w2620]
                tunnel: w2351 -> [w2373 _ w2619]
                tunnel: w2350 -> [w2370 _ w2612]
                tunnel: w2349 -> [w2364 _ w2611]
                tunnel: w2348 -> [w2368 _ w2610]
                tunnel: w2347 -> [w2366 _ w2609]
                tunnel: w2346 -> [_ _ w2608]
                tunnel: w2345 -> [_ _ w2607]
                tunnel: w2344 -> [_ _ w2606]
                tunnel: w2343 -> [w2372 _ w2605]
                tunnel: w2342 -> [_ _ w2604]
                tunnel: w2341 -> [_ _ w2603]
                tunnel: w2340 -> [w2371 _ w2602]
                tunnel: w2339 -> [w2367 _ w2601]
                tunnel: w2338 -> [w2365 _ w2600]
                tunnel: w2337 -> [_ _ w2599]
                tunnel: w2336 -> [w2369 _ w2598]
                frame "R" {
                  n707 = flat-sequence {
                    tunnel: w2364 -> [w2393]
                    tunnel: w2373 -> [w2394]
                    tunnel: w2374 -> [w2395]
                    tunnel: w2375 -> [w2396]
                    tunnel: w2376 -> [w2397]
                    tunnel: [w2397] -> w2360
                    tunnel: [w2396] -> w2359
                    tunnel: [w2395] -> w2358
                    tunnel: [w2394] -> w2357
                    tunnel: [w2393] -> w2356
                    tunnel: [w2413] -> w2392
                    tunnel: [w2412] -> w2391
                    tunnel: [w2409] -> w2390
                    tunnel: [w2408] -> w2389
                    tunnel: w2372 -> [w2407]
                    tunnel: w2371 -> [w2406]
                    tunnel: [w2405] -> w2361
                    tunnel: w2360 -> [w2415]
                    tunnel: w2359 -> [w2414]
                    tunnel: w2358 -> [w2411]
                    tunnel: w2357 -> [w2410]
                    tunnel: w2356 -> [w2405]
                    tunnel: w2392 -> [w2458]
                    tunnel: w2391 -> [w2457]
                    tunnel: [w2456] -> w2388
                    tunnel: [w2455] -> w2387
                    tunnel: [w2454] -> w2386
                    tunnel: [w2453] -> w2385
                    tunnel: w2390 -> [w2452]
                    tunnel: w2389 -> [w2451]
                    tunnel: w2370 -> [w2450]
                    tunnel: w2369 -> [w2449]
                    tunnel: [w2448] -> w2362
                    tunnel: w2361 -> [w2448]
                    tunnel: w2388 -> [w2498]
                    tunnel: w2387 -> [w2497]
                    tunnel: w2386 -> [w2496]
                    tunnel: w2385 -> [w2495]
                    tunnel: [w2494] -> w2384
                    tunnel: [w2493] -> w2383
                    tunnel: [w2492] -> w2382
                    tunnel: [w2491] -> w2381
                    tunnel: w2368 -> [w2490]
                    tunnel: w2367 -> [w2489]
                    tunnel: [w2488] -> w2363
                    tunnel: w2362 -> [w2488]
                    tunnel: [w2540] -> w2380
                    tunnel: [w2539] -> w2379
                    tunnel: [w2538] -> w2378
                    tunnel: [w2537] -> w2377
                    tunnel: w2384 -> [w2536]
                    tunnel: w2383 -> [w2535]
                    tunnel: w2382 -> [w2534]
                    tunnel: w2381 -> [w2533]
                    tunnel: w2366 -> [w2532]
                    tunnel: w2365 -> [w2531]
                    tunnel: w2363 -> [w2530]
                    tunnel: w2380 -> [w2575]
                    tunnel: w2379 -> [w2574]
                    tunnel: w2378 -> [w2573]
                    tunnel: w2377 -> [w2572]
                    frame #0 {
                      n708 = while {
                        i -> [w2399]
                        stop <- w2400 stop-if-true
                        n709 = Increment(x=w2399) -> (x+1=w2401:i32)
                        n710 = global write "Robot Global Data.vi" "Zero Travel"(TRUE) -> ()
                        n711 = global write "Robot Global Data.vi" "Zero Yaw"(TRUE) -> ()
                        n712 = Wait (ms)(milliseconds to wait=u32 10) -> ()  [unwired: 1 out]
                        n713 = Greater Or Equal?(x=w2401, y=1) -> (x >= y?=w2400:bool)
                      }
                    }
                    frame #1 {
                      n714 = while {
                        tunnel: w2415 -> [w2442]
                        tunnel: w2414 -> [w2441]
                        tunnel: [w2440] -> w2413
                        tunnel: [w2439] -> w2412
                        tunnel: w2411 -> [w2433]
                        tunnel: w2410 -> [w2432]
                        tunnel: [w2431] -> w2409
                        tunnel: [w2430] -> w2408
                        tunnel: w2407 -> [w2426]
                        tunnel: w2406 -> [w2425]
                        tunnel: w2405 -> [w2424]
                        stop <- w2437 stop-if-true
                        w2434 = T14 7 items=["PercentOutput"=0, "Position"=1, "Velocity"=2, "Current"=3, "Follower"=5, "MotionProfile"=6, "MotionMagic"=7, "MotionMagicArc"=8, "MotionProfileArc"=10, "Disabled"=15] ("Control Mode")
                        w2443 = T14 7 items=["PercentOutput"=0, "Position"=1, "Velocity"=2, "Current"=3, "Follower"=5, "MotionProfile"=6, "MotionMagic"=7, "MotionMagicArc"=8, "MotionProfileArc"=10, "Disabled"=15] ("Control Mode")
                        n715 = global read "Robot Global Data.vi" "Robot Yaw"() -> (w2423:dbl)
                        n716 = global write "Robot Global Data.vi" "Elevator Bottom"(TRUE) -> ()
                        n717 = Wait (ms)(milliseconds to wait=u32 50) -> ()  [unwired: 1 out]
                        n718 = global write "Robot Global Data.vi" "Zero Travel"(FALSE) -> ()
                        n719 = global write "Robot Global Data.vi" "Zero Yaw"(FALSE) -> ()
                        n720 = global read "Robot Global Data.vi" "Robot Travel"() -> (w2438:dbl)
                        n721 = Greater?(x=w2438, y=303.5) -> (0:w2437:bool)
                        n722 = Multiply(x=304.5 ("Output"), y=217.294) -> (x*y=w2427:dbl)
                        n723 = call-poly <vilib>:"PID.vi"("output range"=w2426, "PID gains"=w2425, "process variable"=w2423, "setpoint"=0.0) -> ("output"=w2420:dbl)  [unwired: 6 in, 1 out]
                        n724 = call <vilib>:"CTRE_Phoenix_MotorControl_Set.vi"("Demand1"=w2420, "DemandType"=w2424, "error in (no error)"=w2432, "Output"=w2427, "Control Mode"=w2434, "PhoenixMotorControlDevRef"=w2433) -> ("error out"=w2436:errorcluster, "PhoenixMotorControlDevRef"=w2435:T4)  [unwired: 4 in]
                        n725 = call-poly <vilib>:"CTRE_Phoenix_MotorController_Get_Enhanced.vi"("PhoenixMotorControlDevRef"=w2435, "error in"=w2436) -> ("PhoenixMotorControlDevRef"=w2431:T4, "error out"=w2430:errorcluster)  [unwired: 8 in, 4 out]
                        n726 = Multiply(x=w2420, y=-1.0) -> (x*y=w2419:dbl)
                        n727 = call <vilib>:"CTRE_Phoenix_MotorControl_Set.vi"("Demand1"=w2419, "DemandType"=w2424, "error in (no error)"=w2441, "Output"=w2427, "Control Mode"=w2443, "PhoenixMotorControlDevRef"=w2442) -> ("error out"=w2445:errorcluster, "PhoenixMotorControlDevRef"=w2444:T4)  [unwired: 4 in]
                        n728 = call-poly <vilib>:"CTRE_Phoenix_MotorController_Get_Enhanced.vi"("PhoenixMotorControlDevRef"=w2444, "error in"=w2445) -> ("PhoenixMotorControlDevRef"=w2440:T4, "error out"=w2439:errorcluster)  [unwired: 8 in, 4 out]
                      }
                    }
                    frame #2 {
                      n729 = while {
                        tunnel: w2458 -> [w2483]
                        tunnel: w2457 -> [w2482]
                        tunnel: [w2481] -> w2456
                        tunnel: [w2480] -> w2455
                        tunnel: [w2476] -> w2454
                        tunnel: [w2475] -> w2453
                        tunnel: w2452 -> [w2474]
                        tunnel: w2451 -> [w2473]
                        tunnel: w2450 -> [w2466]
                        tunnel: w2449 -> [w2465]
                        tunnel: w2448 -> [w2464]
                        stop <- w2472 stop-if-true
                        w2477 = T14 7 items=["PercentOutput"=0, "Position"=1, "Velocity"=2, "Current"=3, "Follower"=5, "MotionProfile"=6, "MotionMagic"=7, "MotionMagicArc"=8, "MotionProfileArc"=10, "Disabled"=15] ("Control Mode")
                        w2484 = T14 7 items=["PercentOutput"=0, "Position"=1, "Velocity"=2, "Current"=3, "Follower"=5, "MotionProfile"=6, "MotionMagic"=7, "MotionMagicArc"=8, "MotionProfileArc"=10, "Disabled"=15] ("Control Mode")
                        n730 = global read "Robot Global Data.vi" "Robot Yaw"() -> (w2463:dbl)
                        n731 = Wait (ms)(milliseconds to wait=u32 50) -> ()  [unwired: 1 out]
                        n732 = global read "Robot Global Data.vi" "Robot Yaw"() -> (w2470:dbl)
                        n733 = Less?(x=w2470, y=-90) -> (x < y?=w2472:bool)
                        n734 = Multiply(x=304.5 ("Output"), y=217.294) -> (x*y=w2467:dbl)
                        n735 = call-poly <vilib>:"PID.vi"("output range"=w2466, "PID gains"=w2465, "process variable"=w2463, "setpoint"=-90.0) -> ("output"=w2460:dbl)  [unwired: 6 in, 1 out]
                        n736 = call <vilib>:"CTRE_Phoenix_MotorControl_Set.vi"("Demand1"=w2460, "DemandType"=w2464, "error in (no error)"=w2473, "Output"=w2467, "Control Mode"=w2477, "PhoenixMotorControlDevRef"=w2474) -> ("error out"=w2479:errorcluster, "PhoenixMotorControlDevRef"=w2478:T4)  [unwired: 4 in]
                        n737 = call-poly <vilib>:"CTRE_Phoenix_MotorController_Get_Enhanced.vi"("PhoenixMotorControlDevRef"=w2478, "error in"=w2479) -> ("PhoenixMotorControlDevRef"=w2476:T4, "error out"=w2475:errorcluster)  [unwired: 8 in, 4 out]
                        n738 = Multiply(x=w2460, y=-1.0) -> (x*y=w2459:dbl)
                        n739 = call <vilib>:"CTRE_Phoenix_MotorControl_Set.vi"("Demand1"=w2459, "DemandType"=w2464, "error in (no error)"=w2482, "Output"=w2467, "Control Mode"=w2484, "PhoenixMotorControlDevRef"=w2483) -> ("error out"=w2486:errorcluster, "PhoenixMotorControlDevRef"=w2485:T4)  [unwired: 4 in]
                        n740 = call-poly <vilib>:"CTRE_Phoenix_MotorController_Get_Enhanced.vi"("PhoenixMotorControlDevRef"=w2485, "error in"=w2486) -> ("PhoenixMotorControlDevRef"=w2481:T4, "error out"=w2480:errorcluster)  [unwired: 8 in, 4 out]
                      }
                    }
                    frame #3 {
                      n741 = while {
                        tunnel: w2498 -> [w2525]
                        tunnel: w2497 -> [w2524]
                        tunnel: [w2521] -> w2494
                        tunnel: [w2520] -> w2492
                        tunnel: [w2516] -> w2493
                        tunnel: [w2515] -> w2491
                        tunnel: w2496 -> [w2514]
                        tunnel: w2495 -> [w2513]
                        tunnel: w2490 -> [w2509]
                        tunnel: w2489 -> [w2508]
                        tunnel: w2488 -> [w2507]
                        stop <- w2522 stop-if-true
                        w2517 = T14 7 items=["PercentOutput"=0, "Position"=1, "Velocity"=2, "Current"=3, "Follower"=5, "MotionProfile"=6, "MotionMagic"=7, "MotionMagicArc"=8, "MotionProfileArc"=10, "Disabled"=15] ("Control Mode")
                        w2526 = T14 7 items=["PercentOutput"=0, "Position"=1, "Velocity"=2, "Current"=3, "Follower"=5, "MotionProfile"=6, "MotionMagic"=7, "MotionMagicArc"=8, "MotionProfileArc"=10, "Disabled"=15] ("Control Mode")
                        n742 = global read "Robot Global Data.vi" "Robot Travel"() -> (w2523:dbl)
                        n743 = Wait (ms)(milliseconds to wait=u32 50) -> ()  [unwired: 1 out]
                        n744 = global read "Robot Global Data.vi" "Robot Yaw"() -> (w2506:dbl)
                        n745 = Greater?(x=w2523, y=308.5) -> (0:w2522:bool)
                        n746 = global write "Robot Global Data.vi" "Elevator Bottom"(FALSE) -> ()
                        n747 = global write "Robot Global Data.vi" "Elevator Top"(TRUE) -> ()
                        n748 = call-poly <vilib>:"PID.vi"("output range"=w2509, "PID gains"=w2508, "process variable"=w2506, "setpoint"=-90.0) -> ("output"=w2503:dbl)  [unwired: 6 in, 1 out]
                        n749 = Multiply(x=w2503, y=-1.0) -> (x*y=w2502:dbl)
                        n750 = Multiply(x=309.5 ("Output"), y=217.294) -> (x*y=w2510:dbl)
                        n751 = call <vilib>:"CTRE_Phoenix_MotorControl_Set.vi"("Demand1"=w2503, "DemandType"=w2507, "error in (no error)"=w2513, "Output"=w2510, "Control Mode"=w2517, "PhoenixMotorControlDevRef"=w2514) -> ("error out"=w2519:errorcluster, "PhoenixMotorControlDevRef"=w2518:T4)  [unwired: 4 in]
                        n752 = call <vilib>:"CTRE_Phoenix_MotorControl_Set.vi"("Demand1"=w2502, "DemandType"=w2507, "error in (no error)"=w2524, "Output"=w2510, "Control Mode"=w2526, "PhoenixMotorControlDevRef"=w2525) -> ("error out"=w2528:errorcluster, "PhoenixMotorControlDevRef"=w2527:T4)  [unwired: 4 in]
                        n753 = call-poly <vilib>:"CTRE_Phoenix_MotorController_Get_Enhanced.vi"("PhoenixMotorControlDevRef"=w2518, "error in"=w2519) -> ("PhoenixMotorControlDevRef"=w2516:T4, "error out"=w2515:errorcluster)  [unwired: 8 in, 4 out]
                        n754 = call-poly <vilib>:"CTRE_Phoenix_MotorController_Get_Enhanced.vi"("PhoenixMotorControlDevRef"=w2527, "error in"=w2528) -> ("PhoenixMotorControlDevRef"=w2521:T4, "error out"=w2520:errorcluster)  [unwired: 8 in, 4 out]
                      }
                    }
                    frame #4 {
                      # "107?"
                      n755 = while {
                        tunnel: w2536 -> [w2567]
                        tunnel: w2534 -> [w2566]
                        tunnel: [w2565] -> w2540
                        tunnel: [w2564] -> w2539
                        tunnel: w2535 -> [w2560]
                        tunnel: w2533 -> [w2559]
                        tunnel: [w2558] -> w2538
                        tunnel: [w2557] -> w2537
                        tunnel: w2532 -> [w2549]
                        tunnel: w2531 -> [w2548]
                        tunnel: w2530 -> [w2547]
                        i -> [w2554]
                        stop <- w2553 stop-if-true
                        w2561 = T14 7 items=["PercentOutput"=0, "Position"=1, "Velocity"=2, "Current"=3, "Follower"=5, "MotionProfile"=6, "MotionMagic"=7, "MotionMagicArc"=8, "MotionProfileArc"=10, "Disabled"=15] ("Control Mode")
                        w2568 = T14 7 items=["PercentOutput"=0, "Position"=1, "Velocity"=2, "Current"=3, "Follower"=5, "MotionProfile"=6, "MotionMagic"=7, "MotionMagicArc"=8, "MotionProfileArc"=10, "Disabled"=15] ("Control Mode")
                        # "ADD INTAKE/ELEVATOR CODE HERE"
                        n756 = Wait (ms)(milliseconds to wait=u32 50) -> ()  [unwired: 1 out]
                        n757 = Increment(x=w2554) -> (x+1=w2555:i32)
                        n758 = global read "Robot Global Data.vi" "Robot Yaw"() -> (w2546:dbl)
                        n759 = Greater Or Equal?(x=w2555, y=20) -> (x >= y?=w2553:bool)
                        n760 = global write "Robot Global Data.vi" "Intake Out Full"(TRUE) -> ()
                        n761 = Multiply(x=309.5 ("Output"), y=217.294) -> (x*y=w2550:dbl)
                        n762 = call-poly <vilib>:"PID.vi"("output range"=w2549, "PID gains"=w2548, "process variable"=w2546, "setpoint"=-90.0) -> ("output"=w2543:dbl)  [unwired: 6 in, 1 out]
                        n763 = call <vilib>:"CTRE_Phoenix_MotorControl_Set.vi"("Demand1"=w2543, "DemandType"=w2547, "error in (no error)"=w2559, "Output"=w2550, "Control Mode"=w2561, "PhoenixMotorControlDevRef"=w2560) -> ("error out"=w2563:errorcluster, "PhoenixMotorControlDevRef"=w2562:T4)  [unwired: 4 in]
                        n764 = call-poly <vilib>:"CTRE_Phoenix_MotorController_Get_Enhanced.vi"("PhoenixMotorControlDevRef"=w2562, "error in"=w2563) -> ("PhoenixMotorControlDevRef"=w2558:T4, "error out"=w2557:errorcluster)  [unwired: 8 in, 4 out]
                        n765 = Multiply(x=w2543, y=-1.0) -> (x*y=w2542:dbl)
                        n766 = call <vilib>:"CTRE_Phoenix_MotorControl_Set.vi"("Demand1"=w2542, "DemandType"=w2547, "error in (no error)"=w2566, "Output"=w2550, "Control Mode"=w2568, "PhoenixMotorControlDevRef"=w2567) -> ("error out"=w2570:errorcluster, "PhoenixMotorControlDevRef"=w2569:T4)  [unwired: 4 in]
                        n767 = call-poly <vilib>:"CTRE_Phoenix_MotorController_Get_Enhanced.vi"("PhoenixMotorControlDevRef"=w2569, "error in"=w2570) -> ("PhoenixMotorControlDevRef"=w2565:T4, "error out"=w2564:errorcluster)  [unwired: 8 in, 4 out]
                      }
                    }
                    frame #5 {
                      n768 = while {
                        tunnel: w2575 -> [w2590]
                        tunnel: w2574 -> [w2589]
                        tunnel: w2573 -> [w2587]
                        tunnel: w2572 -> [w2586]
                        i -> [w2581]
                        stop <- w2580 stop-if-true
                        w2588 = T14 0 items=["PercentOutput"=0, "Position"=1, "Velocity"=2, "Current"=3, "Follower"=5, "MotionProfile"=6, "MotionMagic"=7, "MotionMagicArc"=8, "MotionProfileArc"=10, "Disabled"=15] ("Control Mode")
                        w2591 = T14 0 items=["PercentOutput"=0, "Position"=1, "Velocity"=2, "Current"=3, "Follower"=5, "MotionProfile"=6, "MotionMagic"=7, "MotionMagicArc"=8, "MotionProfileArc"=10, "Disabled"=15] ("Control Mode")
                        n769 = Increment(x=w2581) -> (x+1=w2582:i32)
                        n770 = Wait (ms)(milliseconds to wait=u32 15000) -> ()  [unwired: 1 out]
                        n771 = Greater Or Equal?(x=w2582, y=1) -> (x >= y?=w2580:bool)
                        n772 = global write "Robot Global Data.vi" "Intake Out Full"(FALSE) -> ()
                        n773 = call <vilib>:"CTRE_Phoenix_MotorControl_Set.vi"("DemandType"=T2."DemandType_Neutral", "error in (no error)"=w2586, "Output"=0.0, "Control Mode"=w2588, "PhoenixMotorControlDevRef"=w2587) -> ()  [unwired: 5 in, 2 out]
                        n774 = global write "Robot Global Data.vi" "Elevator Top"(FALSE) -> ()
                        n775 = call <vilib>:"CTRE_Phoenix_MotorControl_Set.vi"("DemandType"=T2."DemandType_Neutral", "error in (no error)"=w2589, "Output"=0.0, "Control Mode"=w2591, "PhoenixMotorControlDevRef"=w2590) -> ()  [unwired: 5 in, 2 out]
                      }
                    }
                  }
                }
                frame Default {
                }
                frame "L" {
                  # "Drive straight"
                  n776 = flat-sequence {
                    tunnel: w2611 -> [w2651]
                    tunnel: w2619 -> [w2652]
                    tunnel: w2620 -> [w2653]
                    tunnel: w2621 -> [w2654]
                    tunnel: w2622 -> [w2655]
                    tunnel: [w2655] -> w2597
                    tunnel: [w2654] -> w2596
                    tunnel: [w2653] -> w2595
                    tunnel: [w2652] -> w2594
                    tunnel: [w2651] -> w2593
                    tunnel: [w2671] -> w2650
                    tunnel: [w2670] -> w2649
                    tunnel: [w2667] -> w2648
                    tunnel: [w2666] -> w2647
                    tunnel: [w2664] -> w2618
                    tunnel: w2606 -> [w2665]
                    tunnel: w2603 -> [w2663]
                    tunnel: w2597 -> [w2673]
                    tunnel: w2596 -> [w2672]
                    tunnel: w2595 -> [w2669]
                    tunnel: w2594 -> [w2668]
                    tunnel: w2593 -> [w2664]
                    tunnel: w2650 -> [w2717]
                    tunnel: w2649 -> [w2716]
                    tunnel: [w2715] -> w2646
                    tunnel: [w2714] -> w2645
                    tunnel: [w2713] -> w2644
                    tunnel: [w2712] -> w2643
                    tunnel: w2648 -> [w2711]
                    tunnel: w2647 -> [w2710]
                    tunnel: w2618 -> [w2709]
                    tunnel: [w2709] -> w2617
                    tunnel: w2605 -> [w2708]
                    tunnel: w2602 -> [w2707]
                    tunnel: w2646 -> [w2758]
                    tunnel: w2645 -> [w2757]
                    tunnel: [w2756] -> w2642
                    tunnel: [w2755] -> w2641
                    tunnel: [w2754] -> w2640
                    tunnel: [w2753] -> w2639
                    tunnel: w2644 -> [w2752]
                    tunnel: w2643 -> [w2751]
                    tunnel: w2617 -> [w2750]
                    tunnel: [w2750] -> w2616
                    tunnel: w2612 -> [w2749]
                    tunnel: w2598 -> [w2748]
                    tunnel: w2642 -> [w2799]
                    tunnel: w2641 -> [w2798]
                    tunnel: [w2797] -> w2638
                    tunnel: [w2796] -> w2637
                    tunnel: [w2795] -> w2636
                    tunnel: [w2794] -> w2635
                    tunnel: w2640 -> [w2793]
                    tunnel: w2639 -> [w2792]
                    tunnel: w2616 -> [w2791]
                    tunnel: [w2791] -> w2615
                    tunnel: w2610 -> [w2790]
                    tunnel: w2601 -> [w2789]
                    tunnel: w2638 -> [w2840]
                    tunnel: w2637 -> [w2839]
                    tunnel: [w2838] -> w2634
                    tunnel: [w2837] -> w2633
                    tunnel: w2636 -> [w2836]
                    tunnel: w2635 -> [w2835]
                    tunnel: [w2834] -> w2632
                    tunnel: [w2833] -> w2631
                    tunnel: w2615 -> [w2832]
                    tunnel: [w2832] -> w2614
                    tunnel: w2609 -> [w2831]
                    tunnel: w2600 -> [w2830]
                    tunnel: w2634 -> [w2883]
                    tunnel: w2633 -> [w2882]
                    tunnel: w2632 -> [w2881]
                    tunnel: w2631 -> [w2880]
                    tunnel: [w2879] -> w2630
                    tunnel: [w2878] -> w2629
                    tunnel: [w2877] -> w2628
                    tunnel: [w2876] -> w2627
                    tunnel: w2614 -> [w2875]
                    tunnel: [w2875] -> w2613
                    tunnel: w2608 -> [w2874]
                    tunnel: w2599 -> [w2873]
                    tunnel: [w2924] -> w2626
                    tunnel: [w2923] -> w2625
                    tunnel: [w2922] -> w2624
                    tunnel: [w2921] -> w2623
                    tunnel: w2630 -> [w2920]
                    tunnel: w2629 -> [w2919]
                    tunnel: w2628 -> [w2918]
                    tunnel: w2627 -> [w2917]
                    tunnel: w2613 -> [w2916]
                    tunnel: w2607 -> [w2915]
                    tunnel: w2604 -> [w2914]
                    tunnel: w2626 -> [w2960]
                    tunnel: w2625 -> [w2959]
                    tunnel: w2624 -> [w2958]
                    tunnel: w2623 -> [w2957]
                    frame #0 {
                      n777 = while {
                        i -> [w2657]
                        stop <- w2658 stop-if-true
                        n778 = Increment(x=w2657) -> (x+1=w2659:i32)
                        n779 = global write "Robot Global Data.vi" "Zero Travel"(TRUE) -> ()
                        n780 = global write "Robot Global Data.vi" "Zero Yaw"(TRUE) -> ()
                        n781 = Wait (ms)(milliseconds to wait=u32 10) -> ()  [unwired: 1 out]
                        n782 = Greater Or Equal?(x=w2659, y=1) -> (x >= y?=w2658:bool)
                      }
                    }
                    frame #1 {
                      n783 = while {
                        tunnel: w2673 -> [w2701]
                        tunnel: w2672 -> [w2700]
                        tunnel: [w2699] -> w2671
                        tunnel: [w2698] -> w2670
                        tunnel: w2669 -> [w2692]
                        tunnel: w2668 -> [w2691]
                        tunnel: [w2690] -> w2667
                        tunnel: [w2689] -> w2666
                        tunnel: w2665 -> [w2683]
                        tunnel: w2664 -> [w2682]
                        tunnel: w2664 -> [w2681]
                        tunnel: w2663 -> [w2680]
                        stop <- w2696 stop-if-true
                        w2693 = T14 7 items=["PercentOutput"=0, "Position"=1, "Velocity"=2, "Current"=3, "Follower"=5, "MotionProfile"=6, "MotionMagic"=7, "MotionMagicArc"=8, "MotionProfileArc"=10, "Disabled"=15] ("Control Mode")
                        w2702 = T14 7 items=["PercentOutput"=0, "Position"=1, "Velocity"=2, "Current"=3, "Follower"=5, "MotionProfile"=6, "MotionMagic"=7, "MotionMagicArc"=8, "MotionProfileArc"=10, "Disabled"=15] ("Control Mode")
                        n784 = global read "Robot Global Data.vi" "Robot Yaw"() -> (w2685:dbl)
                        n785 = global write "Robot Global Data.vi" "Elevator Bottom"(TRUE) -> ()
                        n786 = Wait (ms)(milliseconds to wait=u32 50) -> ()  [unwired: 1 out]
                        n787 = global read "Robot Global Data.vi" "Robot Travel"() -> (w2697:dbl)
                        n788 = global write "Robot Global Data.vi" "Zero Travel"(FALSE) -> ()
                        n789 = global write "Robot Global Data.vi" "Zero Yaw"(FALSE) -> ()
                        n790 = Greater?(x=w2697, y=214.75) -> (0:w2696:bool)
                        n791 = Multiply(x=215.75 ("Output"), y=217.294) -> (x*y=w2686:dbl)
                        n792 = call-poly <vilib>:"PID.vi"("output range"=w2683, "PID gains"=w2680, "process variable"=w2685, "setpoint"=0.0) -> ("output"=w2677:dbl)  [unwired: 6 in, 1 out]
                        n793 = call <vilib>:"CTRE_Phoenix_MotorControl_Set.vi"("Demand1"=w2677, "DemandType"=w2682, "error in (no error)"=w2691, "Output"=w2686, "Control Mode"=w2693, "PhoenixMotorControlDevRef"=w2692) -> ("error out"=w2695:errorcluster, "PhoenixMotorControlDevRef"=w2694:T4)  [unwired: 4 in]
                        n794 = call-poly <vilib>:"CTRE_Phoenix_MotorController_Get_Enhanced.vi"("PhoenixMotorControlDevRef"=w2694, "error in"=w2695) -> ("PhoenixMotorControlDevRef"=w2690:T4, "error out"=w2689:errorcluster)  [unwired: 8 in, 4 out]
                        n795 = Multiply(x=w2677, y=-1.0) -> (x*y=w2678:dbl)
                        n796 = call <vilib>:"CTRE_Phoenix_MotorControl_Set.vi"("Demand1"=w2678, "DemandType"=w2681, "error in (no error)"=w2700, "Output"=w2686, "Control Mode"=w2702, "PhoenixMotorControlDevRef"=w2701) -> ("error out"=w2704:errorcluster, "PhoenixMotorControlDevRef"=w2703:T4)  [unwired: 4 in]
                        n797 = call-poly <vilib>:"CTRE_Phoenix_MotorController_Get_Enhanced.vi"("PhoenixMotorControlDevRef"=w2703, "error in"=w2704) -> ("PhoenixMotorControlDevRef"=w2699:T4, "error out"=w2698:errorcluster)  [unwired: 8 in, 4 out]
                      }
                    }
                    frame #2 {
                      n798 = while {
                        tunnel: w2717 -> [w2743]
                        tunnel: w2716 -> [w2742]
                        tunnel: [w2741] -> w2715
                        tunnel: [w2740] -> w2714
                        tunnel: [w2736] -> w2713
                        tunnel: [w2735] -> w2712
                        tunnel: w2711 -> [w2734]
                        tunnel: w2710 -> [w2733]
                        tunnel: w2709 -> [w2726]
                        tunnel: w2709 -> [w2725]
                        tunnel: w2708 -> [w2722]
                        tunnel: w2707 -> [w2721]
                        stop <- w2732 stop-if-true
                        w2737 = T14 7 items=["PercentOutput"=0, "Position"=1, "Velocity"=2, "Current"=3, "Follower"=5, "MotionProfile"=6, "MotionMagic"=7, "MotionMagicArc"=8, "MotionProfileArc"=10, "Disabled"=15] ("Control Mode")
                        w2744 = T14 7 items=["PercentOutput"=0, "Position"=1, "Velocity"=2, "Current"=3, "Follower"=5, "MotionProfile"=6, "MotionMagic"=7, "MotionMagicArc"=8, "MotionProfileArc"=10, "Disabled"=15] ("Control Mode")
                        n799 = global read "Robot Global Data.vi" "Robot Yaw"() -> (w2724:dbl)
                        n800 = Wait (ms)(milliseconds to wait=u32 50) -> ()  [unwired: 1 out]
                        n801 = global read "Robot Global Data.vi" "Robot Yaw"() -> (w2730:dbl)
                        n802 = Less?(x=w2730, y=-90) -> (x < y?=w2732:bool)
                        n803 = Multiply(x=215.75 ("Output"), y=217.294) -> (x*y=w2727:dbl)
                        n804 = call-poly <vilib>:"PID.vi"("output range"=w2722, "PID gains"=w2721, "process variable"=w2724, "setpoint"=-90.0) -> ("output"=w2718:dbl)  [unwired: 6 in, 1 out]
                        n805 = call <vilib>:"CTRE_Phoenix_MotorControl_Set.vi"("Demand1"=w2718, "DemandType"=w2726, "error in (no error)"=w2733, "Output"=w2727, "Control Mode"=w2737, "PhoenixMotorControlDevRef"=w2734) -> ("error out"=w2739:errorcluster, "PhoenixMotorControlDevRef"=w2738:T4)  [unwired: 4 in]
                        n806 = call-poly <vilib>:"CTRE_Phoenix_MotorController_Get_Enhanced.vi"("PhoenixMotorControlDevRef"=w2738, "error in"=w2739) -> ("PhoenixMotorControlDevRef"=w2736:T4, "error out"=w2735:errorcluster)  [unwired: 8 in, 4 out]
                        n807 = Multiply(x=w2718, y=-1.0) -> (x*y=w2719:dbl)
                        n808 = call <vilib>:"CTRE_Phoenix_MotorControl_Set.vi"("Demand1"=w2719, "DemandType"=w2725, "error in (no error)"=w2742, "Output"=w2727, "Control Mode"=w2744, "PhoenixMotorControlDevRef"=w2743) -> ("error out"=w2746:errorcluster, "PhoenixMotorControlDevRef"=w2745:T4)  [unwired: 4 in]
                        n809 = call-poly <vilib>:"CTRE_Phoenix_MotorController_Get_Enhanced.vi"("PhoenixMotorControlDevRef"=w2745, "error in"=w2746) -> ("PhoenixMotorControlDevRef"=w2741:T4, "error out"=w2740:errorcluster)  [unwired: 8 in, 4 out]
                      }
                    }
                    frame #3 {
                      n810 = while {
                        tunnel: w2758 -> [w2784]
                        tunnel: w2757 -> [w2783]
                        tunnel: [w2780] -> w2756
                        tunnel: [w2779] -> w2755
                        tunnel: [w2775] -> w2754
                        tunnel: [w2774] -> w2753
                        tunnel: w2752 -> [w2773]
                        tunnel: w2751 -> [w2772]
                        tunnel: w2750 -> [w2768]
                        tunnel: w2750 -> [w2767]
                        tunnel: w2749 -> [w2764]
                        tunnel: w2748 -> [w2763]
                        stop <- w2781 stop-if-true
                        w2776 = T14 7 items=["PercentOutput"=0, "Position"=1, "Velocity"=2, "Current"=3, "Follower"=5, "MotionProfile"=6, "MotionMagic"=7, "MotionMagicArc"=8, "MotionProfileArc"=10, "Disabled"=15] ("Control Mode")
                        w2785 = T14 7 items=["PercentOutput"=0, "Position"=1, "Velocity"=2, "Current"=3, "Follower"=5, "MotionProfile"=6, "MotionMagic"=7, "MotionMagicArc"=8, "MotionProfileArc"=10, "Disabled"=15] ("Control Mode")
                        n811 = global read "Robot Global Data.vi" "Robot Travel"() -> (w2782:dbl)
                        n812 = global read "Robot Global Data.vi" "Robot Yaw"() -> (w2766:dbl)
                        n813 = Wait (ms)(milliseconds to wait=u32 50) -> ()  [unwired: 1 out]
                        n814 = Greater?(x=w2782, y=439.75) -> (0:w2781:bool)
                        n815 = Multiply(x=440.75 ("Output"), y=217.294) -> (x*y=w2769:dbl)
                        n816 = call-poly <vilib>:"PID.vi"("output range"=w2764, "PID gains"=w2763, "process variable"=w2766, "setpoint"=-90.0) -> ("output"=w2760:dbl)  [unwired: 6 in, 1 out]
                        n817 = call <vilib>:"CTRE_Phoenix_MotorControl_Set.vi"("Demand1"=w2760, "DemandType"=w2768, "error in (no error)"=w2772, "Output"=w2769, "Control Mode"=w2776, "PhoenixMotorControlDevRef"=w2773) -> ("error out"=w2778:errorcluster, "PhoenixMotorControlDevRef"=w2777:T4)  [unwired: 4 in]
                        n818 = call-poly <vilib>:"CTRE_Phoenix_MotorController_Get_Enhanced.vi"("PhoenixMotorControlDevRef"=w2777, "error in"=w2778) -> ("PhoenixMotorControlDevRef"=w2775:T4, "error out"=w2774:errorcluster)  [unwired: 8 in, 4 out]
                        n819 = Multiply(x=w2760, y=-1.0) -> (x*y=w2761:dbl)
                        n820 = call <vilib>:"CTRE_Phoenix_MotorControl_Set.vi"("Demand1"=w2761, "DemandType"=w2767, "error in (no error)"=w2783, "Output"=w2769, "Control Mode"=w2785, "PhoenixMotorControlDevRef"=w2784) -> ("error out"=w2787:errorcluster, "PhoenixMotorControlDevRef"=w2786:T4)  [unwired: 4 in]
                        n821 = call-poly <vilib>:"CTRE_Phoenix_MotorController_Get_Enhanced.vi"("PhoenixMotorControlDevRef"=w2786, "error in"=w2787) -> ("PhoenixMotorControlDevRef"=w2780:T4, "error out"=w2779:errorcluster)  [unwired: 8 in, 4 out]
                      }
                    }
                    frame #4 {
                      n822 = while {
                        tunnel: w2799 -> [w2825]
                        tunnel: w2798 -> [w2824]
                        tunnel: [w2823] -> w2797
                        tunnel: [w2822] -> w2796
                        tunnel: [w2818] -> w2795
                        tunnel: [w2817] -> w2794
                        tunnel: w2793 -> [w2816]
                        tunnel: w2792 -> [w2815]
                        tunnel: w2791 -> [w2808]
                        tunnel: w2791 -> [w2807]
                        tunnel: w2790 -> [w2804]
                        tunnel: w2789 -> [w2803]
                        stop <- w2812 stop-if-true
                        w2819 = T14 7 items=["PercentOutput"=0, "Position"=1, "Velocity"=2, "Current"=3, "Follower"=5, "MotionProfile"=6, "MotionMagic"=7, "MotionMagicArc"=8, "MotionProfileArc"=10, "Disabled"=15] ("Control Mode")
                        w2826 = T14 7 items=["PercentOutput"=0, "Position"=1, "Velocity"=2, "Current"=3, "Follower"=5, "MotionProfile"=6, "MotionMagic"=7, "MotionMagicArc"=8, "MotionProfileArc"=10, "Disabled"=15] ("Control Mode")
                        n823 = global read "Robot Global Data.vi" "Robot Yaw"() -> (w2813:dbl)
                        n824 = global read "Robot Global Data.vi" "Robot Yaw"() -> (w2806:dbl)
                        n825 = Wait (ms)(milliseconds to wait=u32 50) -> ()  [unwired: 1 out]
                        n826 = Greater?(x=w2813, y=0) -> (0:w2812:bool)
                        n827 = Multiply(x=440.75 ("Output"), y=217.294) -> (x*y=w2809:dbl)
                        n828 = call-poly <vilib>:"PID.vi"("output range"=w2804, "PID gains"=w2803, "process variable"=w2806, "setpoint"=0.0) -> ("output"=w2800:dbl)  [unwired: 6 in, 1 out]
                        n829 = call <vilib>:"CTRE_Phoenix_MotorControl_Set.vi"("Demand1"=w2800, "DemandType"=w2808, "error in (no error)"=w2815, "Output"=w2809, "Control Mode"=w2819, "PhoenixMotorControlDevRef"=w2816) -> ("error out"=w2821:errorcluster, "PhoenixMotorControlDevRef"=w2820:T4)  [unwired: 4 in]
                        n830 = call-poly <vilib>:"CTRE_Phoenix_MotorController_Get_Enhanced.vi"("PhoenixMotorControlDevRef"=w2820, "error in"=w2821) -> ("PhoenixMotorControlDevRef"=w2818:T4, "error out"=w2817:errorcluster)  [unwired: 8 in, 4 out]
                        n831 = Multiply(x=w2800, y=-1.0) -> (x*y=w2801:dbl)
                        n832 = call <vilib>:"CTRE_Phoenix_MotorControl_Set.vi"("Demand1"=w2801, "DemandType"=w2807, "error in (no error)"=w2824, "Output"=w2809, "Control Mode"=w2826, "PhoenixMotorControlDevRef"=w2825) -> ("error out"=w2828:errorcluster, "PhoenixMotorControlDevRef"=w2827:T4)  [unwired: 4 in]
                        n833 = call-poly <vilib>:"CTRE_Phoenix_MotorController_Get_Enhanced.vi"("PhoenixMotorControlDevRef"=w2827, "error in"=w2828) -> ("PhoenixMotorControlDevRef"=w2823:T4, "error out"=w2822:errorcluster)  [unwired: 8 in, 4 out]
                      }
                    }
                    frame #5 {
                      n834 = while {
                        tunnel: w2840 -> [w2868]
                        tunnel: w2839 -> [w2867]
                        tunnel: [w2864] -> w2838
                        tunnel: [w2863] -> w2837
                        tunnel: w2836 -> [w2859]
                        tunnel: w2835 -> [w2858]
                        tunnel: [w2857] -> w2834
                        tunnel: [w2856] -> w2833
                        tunnel: w2832 -> [w2852]
                        tunnel: w2832 -> [w2851]
                        tunnel: w2831 -> [w2848]
                        tunnel: w2830 -> [w2847]
                        stop <- w2865 stop-if-true
                        w2860 = T14 7 items=["PercentOutput"=0, "Position"=1, "Velocity"=2, "Current"=3, "Follower"=5, "MotionProfile"=6, "MotionMagic"=7, "MotionMagicArc"=8, "MotionProfileArc"=10, "Disabled"=15] ("Control Mode")
                        w2869 = T14 7 items=["PercentOutput"=0, "Position"=1, "Velocity"=2, "Current"=3, "Follower"=5, "MotionProfile"=6, "MotionMagic"=7, "MotionMagicArc"=8, "MotionProfileArc"=10, "Disabled"=15] ("Control Mode")
                        n835 = global read "Robot Global Data.vi" "Robot Travel"() -> (w2866:dbl)
                        n836 = global read "Robot Global Data.vi" "Robot Yaw"() -> (w2850:dbl)
                        n837 = Wait (ms)(milliseconds to wait=u32 50) -> ()  [unwired: 1 out]
                        n838 = Greater?(x=w2866, y=528.5) -> (0:w2865:bool)
                        n839 = global write "Robot Global Data.vi" "Elevator Bottom"(FALSE) -> ()
                        n840 = global write "Robot Global Data.vi" "Elevator Top"(TRUE) -> ()
                        n841 = Multiply(x=529.5 ("Output"), y=217.294) -> (x*y=w2853:dbl)
                        n842 = call-poly <vilib>:"PID.vi"("output range"=w2848, "PID gains"=w2847, "process variable"=w2850, "setpoint"=0.0) -> ("output"=w2844:dbl)  [unwired: 6 in, 1 out]
                        n843 = call <vilib>:"CTRE_Phoenix_MotorControl_Set.vi"("Demand1"=w2844, "DemandType"=w2852, "error in (no error)"=w2858, "Output"=w2853, "Control Mode"=w2860, "PhoenixMotorControlDevRef"=w2859) -> ("error out"=w2862:errorcluster, "PhoenixMotorControlDevRef"=w2861:T4)  [unwired: 4 in]
                        n844 = call-poly <vilib>:"CTRE_Phoenix_MotorController_Get_Enhanced.vi"("PhoenixMotorControlDevRef"=w2861, "error in"=w2862) -> ("PhoenixMotorControlDevRef"=w2857:T4, "error out"=w2856:errorcluster)  [unwired: 8 in, 4 out]
                        n845 = Multiply(x=w2844, y=-1.0) -> (x*y=w2845:dbl)
                        n846 = call <vilib>:"CTRE_Phoenix_MotorControl_Set.vi"("Demand1"=w2845, "DemandType"=w2851, "error in (no error)"=w2867, "Output"=w2853, "Control Mode"=w2869, "PhoenixMotorControlDevRef"=w2868) -> ("error out"=w2871:errorcluster, "PhoenixMotorControlDevRef"=w2870:T4)  [unwired: 4 in]
                        n847 = call-poly <vilib>:"CTRE_Phoenix_MotorController_Get_Enhanced.vi"("PhoenixMotorControlDevRef"=w2870, "error in"=w2871) -> ("PhoenixMotorControlDevRef"=w2864:T4, "error out"=w2863:errorcluster)  [unwired: 8 in, 4 out]
                      }
                    }
                    frame #6 {
                      n848 = while {
                        tunnel: w2883 -> [w2909]
                        tunnel: w2882 -> [w2908]
                        tunnel: [w2907] -> w2879
                        tunnel: [w2906] -> w2878
                        tunnel: [w2902] -> w2877
                        tunnel: [w2901] -> w2876
                        tunnel: w2881 -> [w2900]
                        tunnel: w2880 -> [w2899]
                        tunnel: w2875 -> [w2892]
                        tunnel: w2875 -> [w2891]
                        tunnel: w2874 -> [w2888]
                        tunnel: w2873 -> [w2887]
                        stop <- w2896 stop-if-true
                        w2903 = T14 7 items=["PercentOutput"=0, "Position"=1, "Velocity"=2, "Current"=3, "Follower"=5, "MotionProfile"=6, "MotionMagic"=7, "MotionMagicArc"=8, "MotionProfileArc"=10, "Disabled"=15] ("Control Mode")
                        w2910 = T14 7 items=["PercentOutput"=0, "Position"=1, "Velocity"=2, "Current"=3, "Follower"=5, "MotionProfile"=6, "MotionMagic"=7, "MotionMagicArc"=8, "MotionProfileArc"=10, "Disabled"=15] ("Control Mode")
                        n849 = global read "Robot Global Data.vi" "Robot Yaw"() -> (w2897:dbl)
                        n850 = global read "Robot Global Data.vi" "Robot Yaw"() -> (w2890:dbl)
                        n851 = Wait (ms)(milliseconds to wait=u32 50) -> ()  [unwired: 1 out]
                        n852 = Greater?(x=w2897, y=90) -> (0:w2896:bool)
                        n853 = Multiply(x=529.5 ("Output"), y=217.294) -> (x*y=w2893:dbl)
                        n854 = call-poly <vilib>:"PID.vi"("output range"=w2888, "PID gains"=w2887, "process variable"=w2890, "setpoint"=90.0) -> ("output"=w2884:dbl)  [unwired: 6 in, 1 out]
                        n855 = call <vilib>:"CTRE_Phoenix_MotorControl_Set.vi"("Demand1"=w2884, "DemandType"=w2892, "error in (no error)"=w2899, "Output"=w2893, "Control Mode"=w2903, "PhoenixMotorControlDevRef"=w2900) -> ("error out"=w2905:errorcluster, "PhoenixMotorControlDevRef"=w2904:T4)  [unwired: 4 in]
                        n856 = call-poly <vilib>:"CTRE_Phoenix_MotorController_Get_Enhanced.vi"("PhoenixMotorControlDevRef"=w2904, "error in"=w2905) -> ("PhoenixMotorControlDevRef"=w2902:T4, "error out"=w2901:errorcluster)  [unwired: 8 in, 4 out]
                        n857 = Multiply(x=w2884, y=-1.0) -> (x*y=w2885:dbl)
                        n858 = call <vilib>:"CTRE_Phoenix_MotorControl_Set.vi"("Demand1"=w2885, "DemandType"=w2891, "error in (no error)"=w2908, "Output"=w2893, "Control Mode"=w2910, "PhoenixMotorControlDevRef"=w2909) -> ("error out"=w2912:errorcluster, "PhoenixMotorControlDevRef"=w2911:T4)  [unwired: 4 in]
                        n859 = call-poly <vilib>:"CTRE_Phoenix_MotorController_Get_Enhanced.vi"("PhoenixMotorControlDevRef"=w2911, "error in"=w2912) -> ("PhoenixMotorControlDevRef"=w2907:T4, "error out"=w2906:errorcluster)  [unwired: 8 in, 4 out]
                      }
                    }
                    frame #7 {
                      n860 = while {
                        tunnel: [w2952] -> w2924
                        tunnel: [w2951] -> w2923
                        tunnel: [w2947] -> w2922
                        tunnel: [w2946] -> w2921
                        tunnel: w2920 -> [w2945]
                        tunnel: w2919 -> [w2944]
                        tunnel: w2918 -> [w2943]
                        tunnel: w2917 -> [w2942]
                        tunnel: w2916 -> [w2934]
                        tunnel: w2916 -> [w2933]
                        tunnel: w2915 -> [w2930]
                        tunnel: w2914 -> [w2929]
                        i -> [w2939]
                        stop <- w2938 stop-if-true
                        w2948 = T14 7 items=["PercentOutput"=0, "Position"=1, "Velocity"=2, "Current"=3, "Follower"=5, "MotionProfile"=6, "MotionMagic"=7, "MotionMagicArc"=8, "MotionProfileArc"=10, "Disabled"=15] ("Control Mode")
                        w2953 = T14 7 items=["PercentOutput"=0, "Position"=1, "Velocity"=2, "Current"=3, "Follower"=5, "MotionProfile"=6, "MotionMagic"=7, "MotionMagicArc"=8, "MotionProfileArc"=10, "Disabled"=15] ("Control Mode")
                        # "ADD INTAKE/ELEVATOR CODE HERE"
                        n861 = global read "Robot Global Data.vi" "Robot Yaw"() -> (w2932:dbl)
                        n862 = Increment(x=w2939) -> (x+1=w2940:i32)
                        n863 = Wait (ms)(milliseconds to wait=u32 50) -> ()  [unwired: 1 out]
                        n864 = Greater Or Equal?(x=w2940, y=20) -> (x >= y?=w2938:bool)
                        n865 = global write "Robot Global Data.vi" "Intake Out Full"(TRUE) -> ()
                        n866 = Multiply(x=529.5 ("Output"), y=217.294) -> (x*y=w2935:dbl)
                        n867 = call-poly <vilib>:"PID.vi"("output range"=w2930, "PID gains"=w2929, "process variable"=w2932, "setpoint"=90.0) -> ("output"=w2926:dbl)  [unwired: 6 in, 1 out]
                        n868 = call <vilib>:"CTRE_Phoenix_MotorControl_Set.vi"("Demand1"=w2926, "DemandType"=w2934, "error in (no error)"=w2942, "Output"=w2935, "Control Mode"=w2948, "PhoenixMotorControlDevRef"=w2943) -> ("error out"=w2950:errorcluster, "PhoenixMotorControlDevRef"=w2949:T4)  [unwired: 4 in]
                        n869 = call-poly <vilib>:"CTRE_Phoenix_MotorController_Get_Enhanced.vi"("PhoenixMotorControlDevRef"=w2949, "error in"=w2950) -> ("PhoenixMotorControlDevRef"=w2947:T4, "error out"=w2946:errorcluster)  [unwired: 8 in, 4 out]
                        n870 = Multiply(x=w2926, y=-1.0) -> (x*y=w2927:dbl)
                        n871 = call <vilib>:"CTRE_Phoenix_MotorControl_Set.vi"("Demand1"=w2927, "DemandType"=w2933, "error in (no error)"=w2944, "Output"=w2935, "Control Mode"=w2953, "PhoenixMotorControlDevRef"=w2945) -> ("error out"=w2955:errorcluster, "PhoenixMotorControlDevRef"=w2954:T4)  [unwired: 4 in]
                        n872 = call-poly <vilib>:"CTRE_Phoenix_MotorController_Get_Enhanced.vi"("PhoenixMotorControlDevRef"=w2954, "error in"=w2955) -> ("PhoenixMotorControlDevRef"=w2952:T4, "error out"=w2951:errorcluster)  [unwired: 8 in, 4 out]
                      }
                    }
                    frame #8 {
                      n873 = while {
                        tunnel: w2960 -> [w2975]
                        tunnel: w2959 -> [w2974]
                        tunnel: w2958 -> [w2972]
                        tunnel: w2957 -> [w2971]
                        i -> [w2965]
                        stop <- w2966 stop-if-true
                        w2973 = T14 0 items=["PercentOutput"=0, "Position"=1, "Velocity"=2, "Current"=3, "Follower"=5, "MotionProfile"=6, "MotionMagic"=7, "MotionMagicArc"=8, "MotionProfileArc"=10, "Disabled"=15] ("Control Mode")
                        w2976 = T14 0 items=["PercentOutput"=0, "Position"=1, "Velocity"=2, "Current"=3, "Follower"=5, "MotionProfile"=6, "MotionMagic"=7, "MotionMagicArc"=8, "MotionProfileArc"=10, "Disabled"=15] ("Control Mode")
                        n874 = Increment(x=w2965) -> (x+1=w2967:i32)
                        n875 = Wait (ms)(milliseconds to wait=u32 15000) -> ()  [unwired: 1 out]
                        n876 = call <vilib>:"CTRE_Phoenix_MotorControl_Set.vi"("DemandType"=T2."DemandType_Neutral", "error in (no error)"=w2971, "Output"=0.0, "Control Mode"=w2973, "PhoenixMotorControlDevRef"=w2972) -> ()  [unwired: 5 in, 2 out]
                        n877 = Greater Or Equal?(x=w2967, y=1) -> (x >= y?=w2966:bool)
                        n878 = call <vilib>:"CTRE_Phoenix_MotorControl_Set.vi"("DemandType"=T2."DemandType_Neutral", "error in (no error)"=w2974, "Output"=0.0, "Control Mode"=w2976, "PhoenixMotorControlDevRef"=w2975) -> ()  [unwired: 5 in, 2 out]
                        n879 = global write "Robot Global Data.vi" "Intake Out Full"(FALSE) -> ()
                        n880 = global write "Robot Global Data.vi" "Elevator Top"(FALSE) -> ()
                      }
                    }
                  }
                }
              }
            }
          }
        }
        frame True {
          # "Autonomous disabled"
          # "PUT NOTHING IN HERE\n\n(AUSTIN, THIS MEANS YOU!!!)"
        }
      }
    }
  }
